vi "Actor Core.vi"(8 "error in":errorcluster, 11 "Machine Interface Actor in":refnum<class "Machine Interface.lvclass">) -> (0 "error out":errorcluster, 3 "Actor out":refnum<class "Actor.lvclass">)   [LabVIEW 2019, in "Machine Interface.lvclass"]
doc: "(<B>Filename</B>: Actor Framework.lvlib:Actor.lvclass:Actor Core.vi)\n\nReceives messages to the actor, reacts to them, and initiates any error handling that may shut the actor down.\n\nDescendant classes may override this VI to append parallel tasks for the actor to complete while it handles messages. Overrides use the Call Parent Method node."
uses:
  Machine Interface.lvclass
  <vilib>/event_ctls.llb/usereventprio.ctl
  <vilib>/ActorFramework/Actor/Actor.lvclass
  <vilib>/ActorFramework/Message Enqueuer/Message Enqueuer.lvclass
  Common/Controls/Acknowledgement.ctl
  Controls/Machine Interface Config File Structure_MI.ctl
  Controls/Local Data_MI.ctl
  Controls/Output Cluster_MI.ctl
  Common/Controls/Diagnostics Result.ctl
  <vilib>/Instr/_visa.llb/VISA Configure Serial Port (Instr).vi
  Controls/Response from Hardware_MI.ctl
  Common/Controls/Pop-up Input.ctl
  C:/Program Files/National Instruments/LabVIEW 2019/vi.lib/ActorFramework/Actor/Actor.lvclass
panel:
  out "LightCamSeqTriggerCount":i32
  in  "MI Offline?":bool
  out "VISA":refnum<visa-resource-name>
  out "VISA resource":refnum<visa-resource-name>
  in  "Message from Arduino":string(combo)
  out "Arduino Read buffer":string
  out "Bytes at Port":u32
  out "Number of Racks":i32
  out "Ping Response, Button Press, Incorrect Opcode":T1
  out "Rack1 Response":T2
  out "Rack2 Response":T2
  in  "OK":bool
  in  "Part Name":string(combo)
  in  "Inspection Status":string(combo)
  out "Label.Text":string
  in  "State Message from Inspection Statemachine":string(combo)
  # "Used for Offline MI Testing"
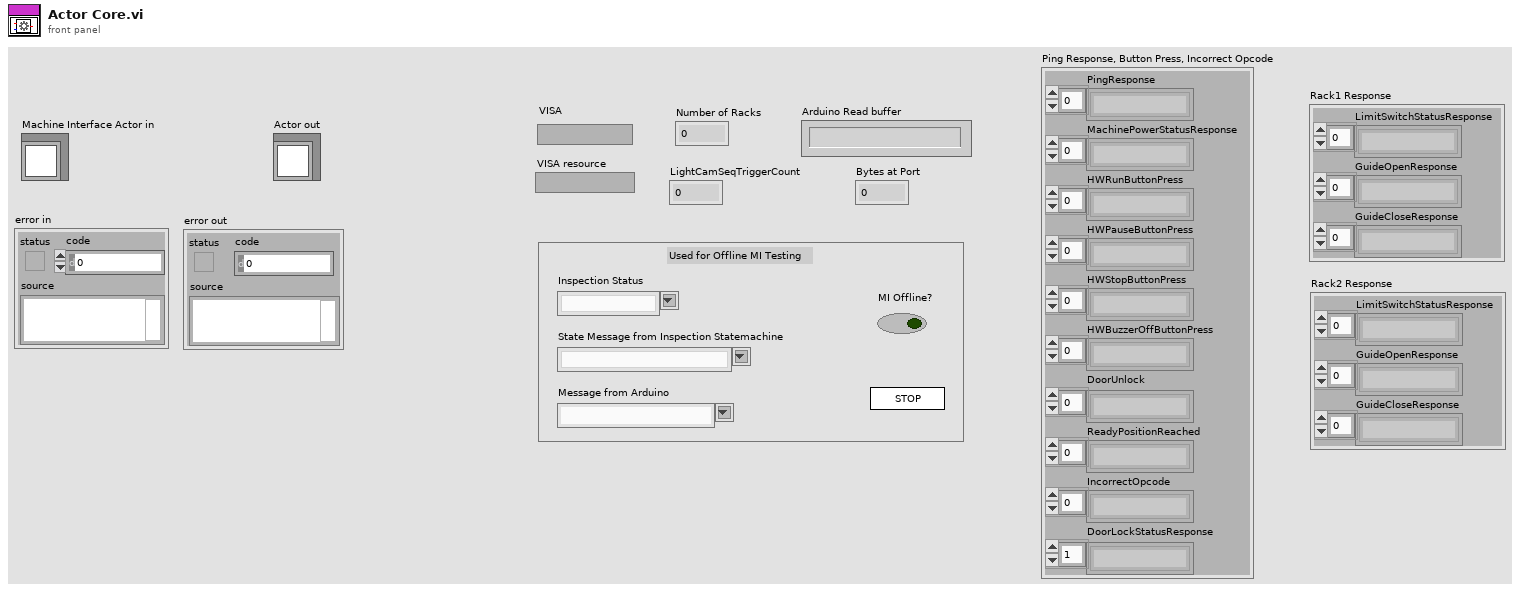
[diagram p1: front panel]
types:
  T1 = typedef "Machine Interface.lvclass/Response from Hardware_MI.ctl" = cluster{"PingResponse":string[], "MachinePowerStatusResponse":string[], "HWRunButtonPress":string[], "HWPauseButtonPress":string[], "HWStopButtonPress":string[], "HWBuzzerOffButtonPress":string[], "DoorUnlock":string[], "ReadyPositionReached":string[], "IncorrectOpcode":string[], "DoorLockStatusResponse":string[]}
  T2 = cluster{"LimitSwitchStatusResponse":string[], "GuideOpenResponse":string[], "GuideCloseResponse":string[]}
  T3 = typedef "Machine Interface.lvclass/Local Data_MI.ctl" = cluster{"Timeout":i32, "Core":cluster{"Current VI Reference":refnum<vi>, "Close Panel on Exit?":bool}, "MIParameters":T4, "Number of Racks":i32, "First Call?":bool, "Message to SM on Timeout":string, "Message from Hardware":string, "Part details":cluster{"Name":string, "RackDependentOpcodes":cluster{"MotorStepsForReadyToInsert":string[], "MotorStepsForReadyToRun":string[], "SetIndex":string[], "EnableSensor":string[], "PowerOnSensor":string[], "DisableSensor":string[], "StartReelerMotor":string[], "StopReelerMotor":string[]}[]}, "State":string, "Ping Response, Button Press, Incorrect Opcode":refnum<vi>[], "Rack1 Response":refnum<vi>[], "Rack2 Response":refnum<vi>[], "LightCamSeqTriggerCount":i32, "Pass after Pause on Fail":bool, "MI Offline?":bool, "Ping Response, Button Press, Incorrect Opcode":T1, "Rack1 Response":cluster{"LimitSwitchStatusResponse":string[], "GuideOpenResponse":string[], "GuideCloseResponse":string[]}, "Rack2 Response":cluster{"LimitSwitchStatusResponse":string[], "GuideOpenResponse":string[], "GuideCloseResponse":string[]}, "Output Cluster_MI":T5, "DisableRun":bool}
  T4 = typedef "Machine Interface.lvclass/Machine Interface Config File Structure_MI.ctl" = cluster{"SpecificationVersion":string, "CompatibleSoftwareVersions":string[], "FrontPanelOpen":bool, "DelayValuesInms":cluster{"TimingUnitSetup":i32, "Strobing":i32, "TowerLampDiagnostics":i32, "Run":i32, "DisableSensors":i32}, "HardwareConfigurationParameters":cluster{"BaudRate":dbl}, "MIRecipeOpcodes":cluster{"DeviceReadiness":cluster{"Ping":string[], "PingResponse":string[]}, "Initialization":cluster{string[]}[], "MachinePowerStatus":cluster{"MachinePowerStatusCheck":string[], "MachinePowerStatusResponse":string[]}, "DoorLockStatus":cluster{"DoorLockStatusCheck":string[], "DoorLockStatusResponse":string[], "Enable":string[], "Disable":string[]}, "OpenLimitSwitchStatus":cluster{"LimitSwitchStatusCheck":string[], "LimitSwitchStatusResponse":string[]}[], "MotorDiagnostics":cluster{"GuideOpen":string[], "GuideOpenResponse":string[], "GuideClose":string[], "GuideCloseResponse":string[], "RotateReelerMotor":string[]}[], "HardwareButtonDiagnostics":cluster{"Run":string[], "Pause":string[], "Stop":string[], "BuzzerOff":string[]}, "TriggerLightCameraSequence":cluster{"Name":string, "On":string[], "Off":string[]}[], "SensorDiagnostics":cluster{"Name":string, "Opcodes":string[]}[], "TowerLampDiagnostics":cluster{"RedLamp":string[], "YellowLamp":string[], "GreenLamp":string[], "Buzzer":string[]}, "Select":cluster{string[]}[], "Run":cluster{"HardwareButtonStatus":string[], "Pass":cluster{"TowerLampStatus":string[]}}, "Pause":cluster{"PauseButtonPress":cluster{string[]}[], "Fail":cluster{string[]}[], "BuzzerOffButtonPress":string[]}, "Exit":cluster{"Shutdown":string[]}, "DHBLS":cluster{string[]}[], "PartsList":cluster{"Name":string, "RackDependentOpcodes":cluster{"MotorStepsForReadyToInsert":string[], "MotorStepsForReadyToRun":string[], "SetIndex":string[], "EnableSensor":string[], "PowerOnSensor":string[], "DisableSensor":string[], "StartReelerMotor":string[], "StopReelerMotor":string[]}[]}[], "HardwareButtonPressed":cluster{"RunButtonPress":string[], "PauseButtonPress":string[], "StopButtonPress":string[], "BuzzerOffButtonPress":string[], "DoorUnlock":string[]}, "ReadyPositionReached":string[], "IncorrectOpcode":string[]}}
  T5 = typedef "Machine Interface.lvclass/Output Cluster_MI.ctl" = cluster{"Acknowledgement":T6, "Diagnostics Result":T7, "Message to SM":string, "Button Press":string, "Error Message":string, "Loading bar cluster":T8}
  T6 = typedef "Acknowledgement.ctl" = cluster{"Enqueuer":refnum<class "Message Enqueuer.lvclass">, "VIReference":refnum<vi>, "VIName":string}
  T7 = typedef "Diagnostics Result.ctl" = cluster{"Result":bool, "StateMessage":string}
  T8 = typedef "Pop-up Input.ctl" = cluster{"Pop-up Type":enum16{"Open Logo Display", "Close Logo Display", "Open Loading Bar", "Close Loading Bar", "Open Alert Display", "Close Alert Display", "One button dialog box", "Two button dialog box", "User Authentication"}, "Title":string, "Message":string, "Button 1 Text":string, "Button 2 Text":string, "Show Close? T/F":bool, "Title Blink? T/F":bool, "Title Blink Colour":u32}
  T9 = enum32{"invalid app kind", "Development System", "Run Time System", "Student Edition", "Embedded LabVIEW", "Evaluation", "Custom"}
  T10 = cluster{"Current VI Reference":refnum<vi>, "Close Panel on Exit?":bool}
  T11 = enum32{"Invalid", "Standard", "Closed", "Hidden", "Minimized", "Maximized"}
  T12 = cluster{"Name":string, "RackDependentOpcodes":cluster{"MotorStepsForReadyToInsert":string[], "MotorStepsForReadyToRun":string[], "SetIndex":string[], "EnableSensor":string[], "PowerOnSensor":string[], "DisableSensor":string[], "StartReelerMotor":string[], "StopReelerMotor":string[]}[]}
  T13 = cluster{"Name":string, "RackDependentOpcodes":cluster{"MotorStepsForReadyToInsert":string[], "MotorStepsForReadyToRun":string[], "SetIndex":string[], "EnableSensor":string[], "PowerOnSensor":string[], "DisableSensor":string[], "StartReelerMotor":string[], "StopReelerMotor":string[]}[]}[]
  T14 = cluster{"MotorStepsForReadyToInsert":string[], "MotorStepsForReadyToRun":string[], "SetIndex":string[], "EnableSensor":string[], "PowerOnSensor":string[], "DisableSensor":string[], "StartReelerMotor":string[], "StopReelerMotor":string[]}[]
  T15 = cluster{"MotorStepsForReadyToInsert":string[], "MotorStepsForReadyToRun":string[], "SetIndex":string[], "EnableSensor":string[], "PowerOnSensor":string[], "DisableSensor":string[], "StartReelerMotor":string[], "StopReelerMotor":string[]}
  T16 = typedef "usereventprio.ctl" = enum32{"high priority", "normal priority"}
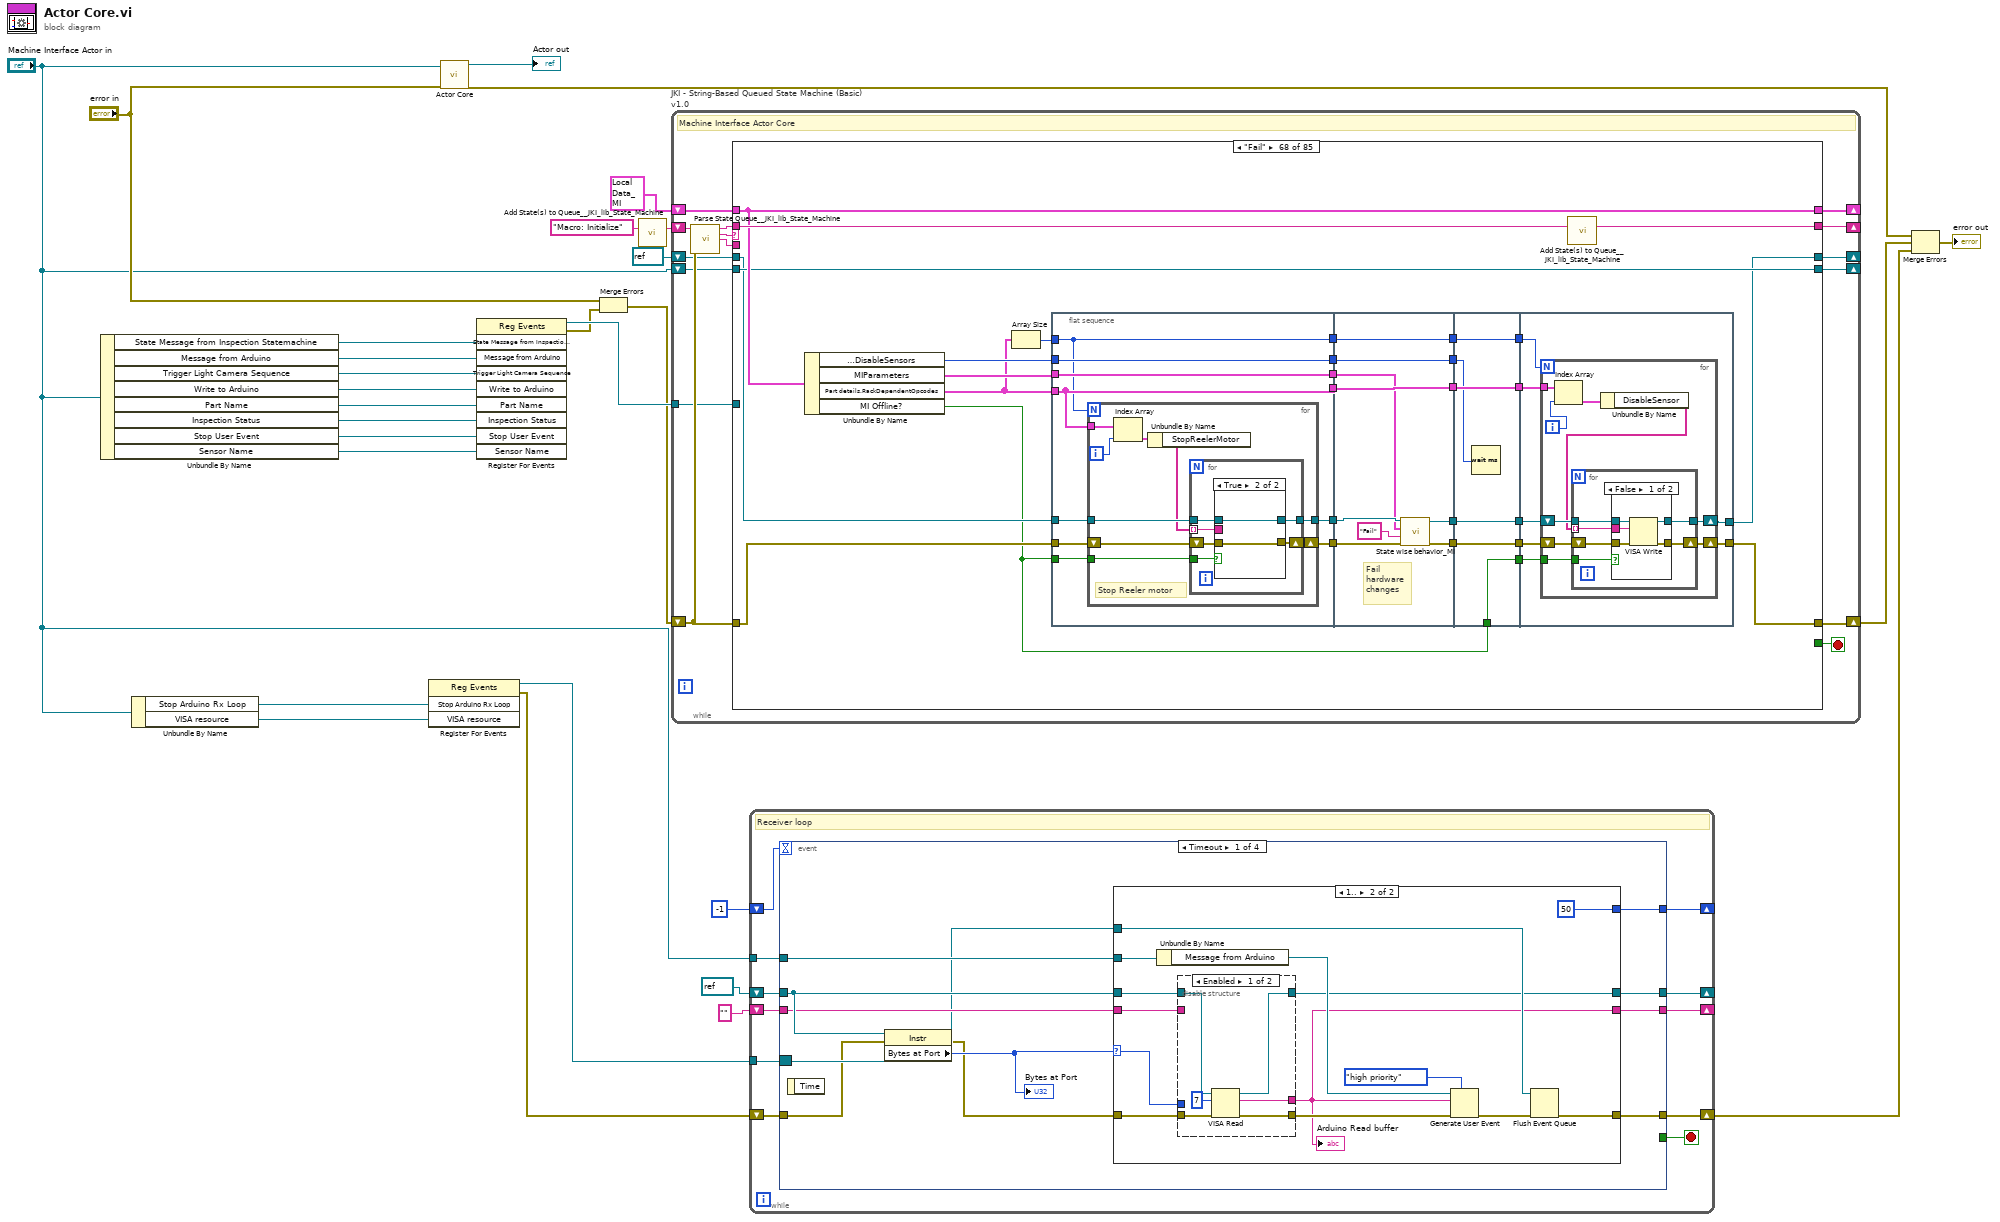
[diagram p0: block diagram]
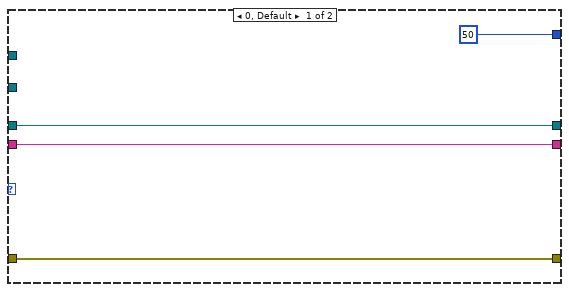
[diagram p2: hidden frame]
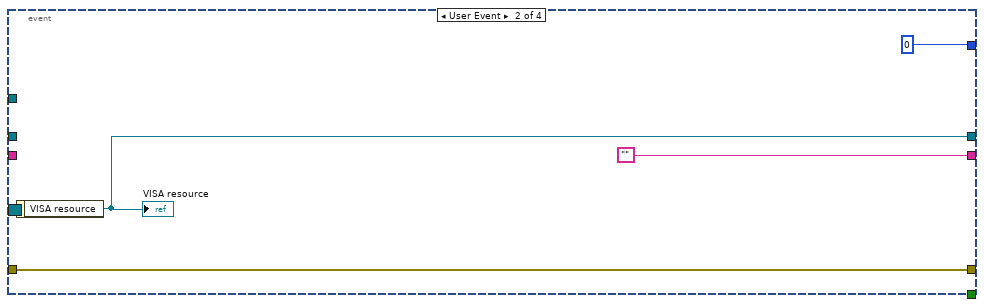
[diagram p4: hidden frame]
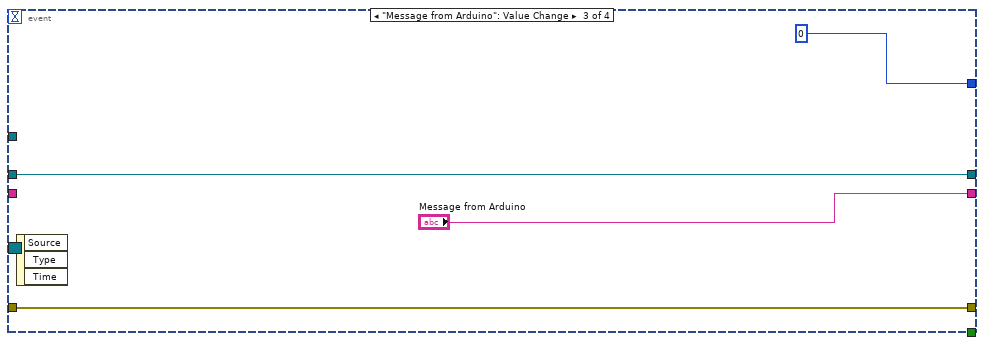
[diagram p5: hidden frame]
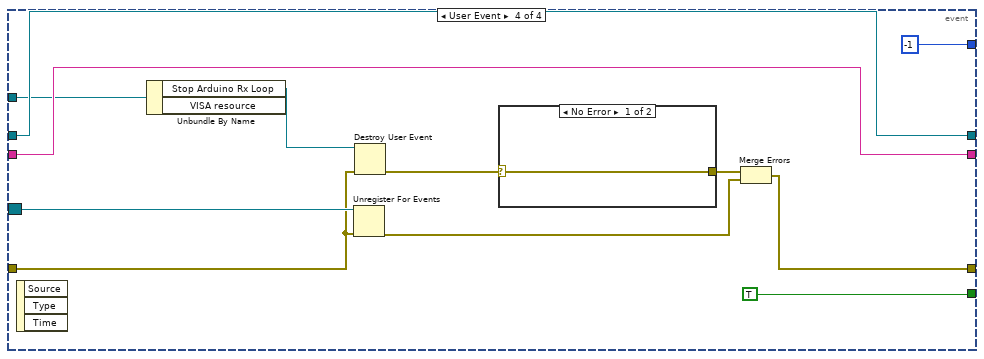
[diagram p6: hidden frame]
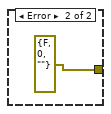
[diagram p7: hidden frame]
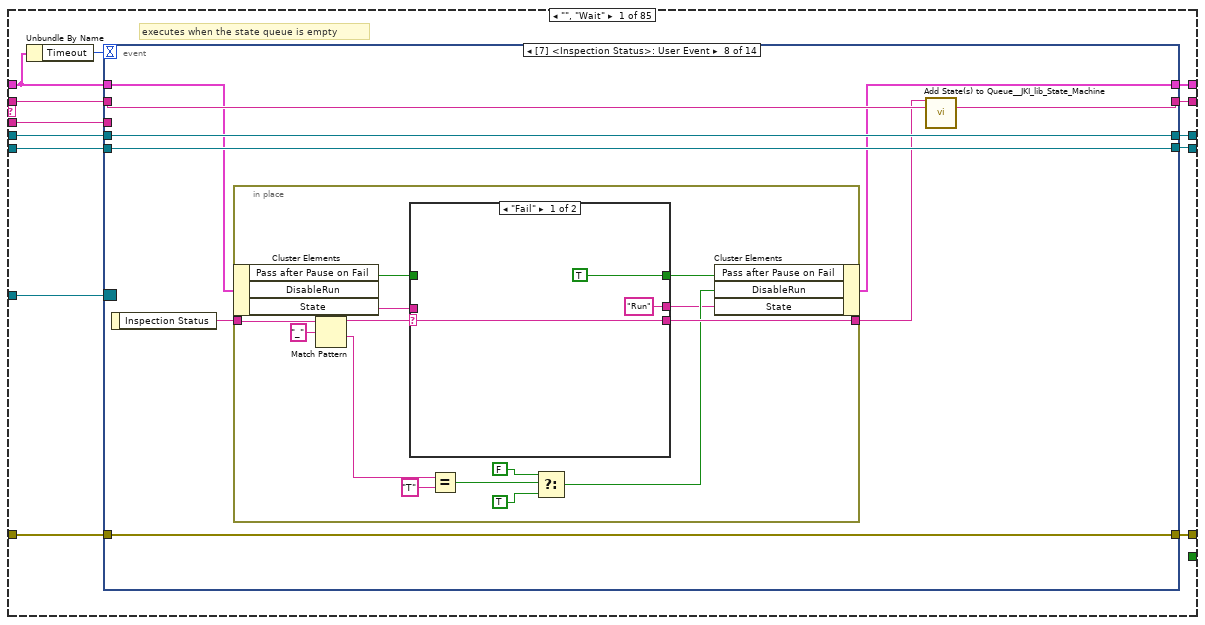
[diagram p8: hidden frame]
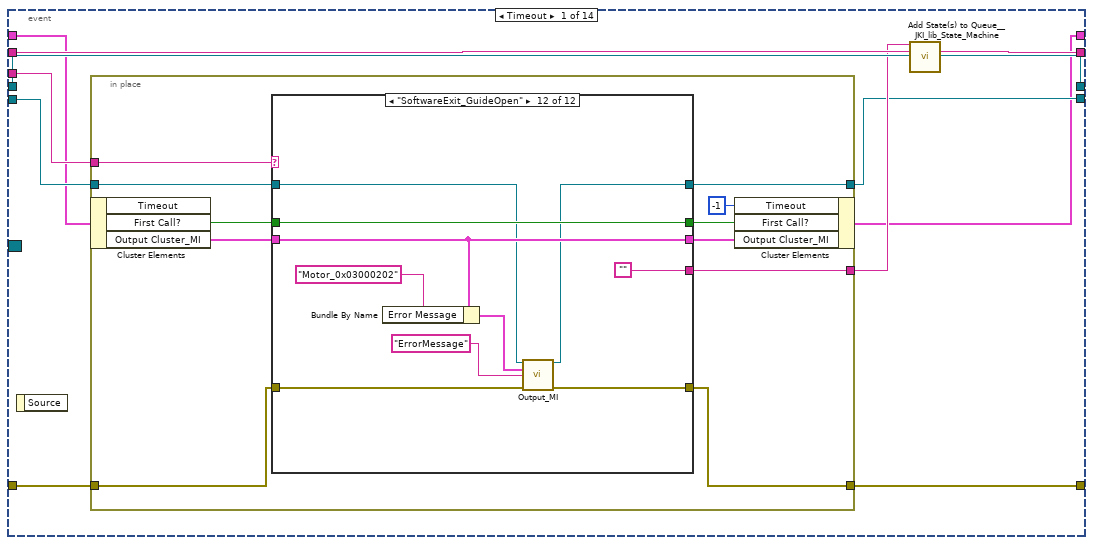
[diagram p9: hidden frame]
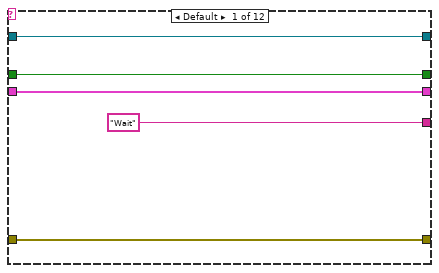
[diagram p10: hidden frame]
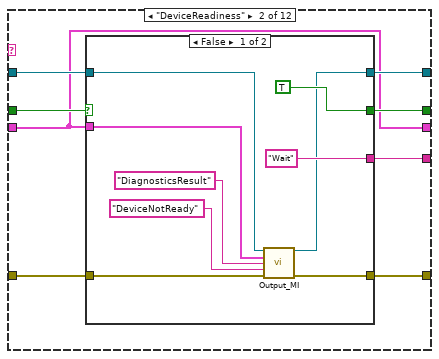
[diagram p11: hidden frame]
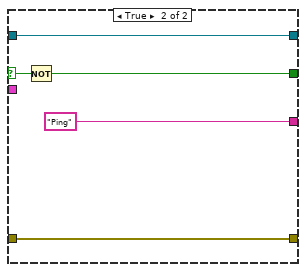
[diagram p12: hidden frame]
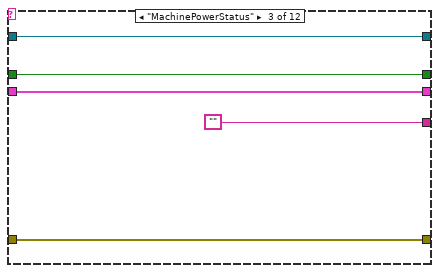
[diagram p13: hidden frame]
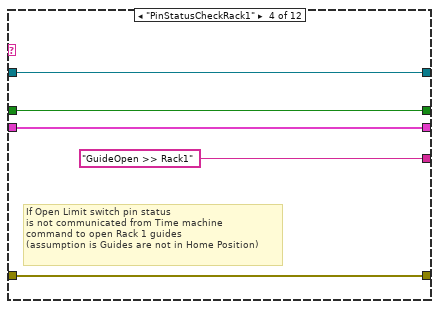
[diagram p14: hidden frame]
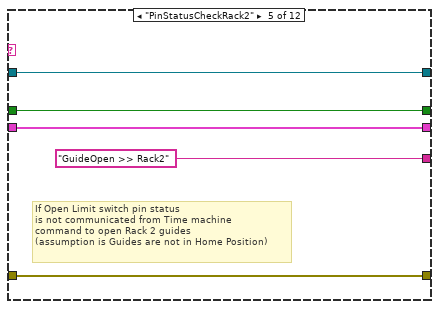
[diagram p15: hidden frame]
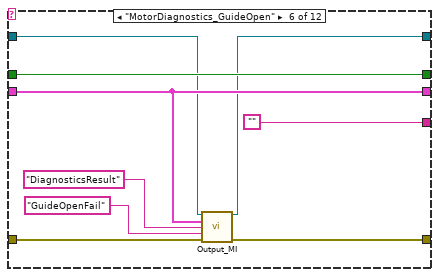
[diagram p16: hidden frame]
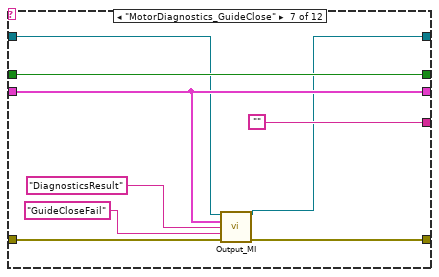
[diagram p17: hidden frame]
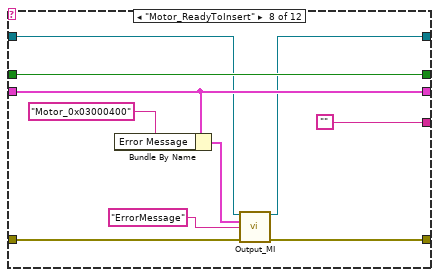
[diagram p18: hidden frame]
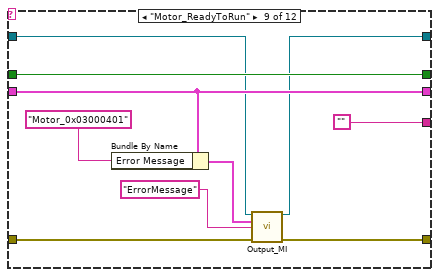
[diagram p19: hidden frame]
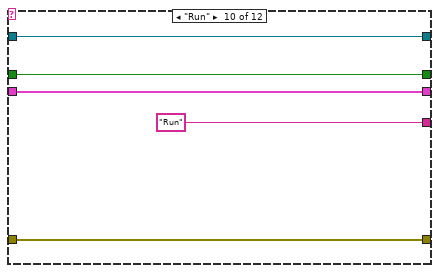
[diagram p20: hidden frame]
diagram:
  n1 = Unbundle By Name("Machine Interface Actor in") -> ("State Message from Inspection Statemachine"=w20:refnum<user-event>, "Message from Arduino"=w19:refnum<user-event>, "Trigger Light Camera Sequence"=w18:refnum<user-event>, "Write to Arduino"=w17:refnum<user-event>, "Part Name"=w16:refnum<user-event>, "Inspection Status"=w15:refnum<user-event>, "Stop User Event"=w12:refnum<user-event>, "Sensor Name"=w8:refnum<user-event>)
  n2 = Unbundle By Name("Machine Interface Actor in") -> ("Stop Arduino Rx Loop"=w6:refnum<user-event>, "VISA resource"=w5:refnum<user-event>)
  n3 = register-events(w6, w5) -> (reference out=w23:refnum<event-registration>, error out=w22:errorcluster)  [unwired: 2 in]
  n4 = call-parent "Actor Core.vi"("error in"="error in", "Actor in"="Machine Interface Actor in") -> ("error out"=w28:errorcluster, "Actor out"=→"Actor out":refnum<class "Actor.lvclass">)  [unwired: 8 in]
  n5 = register-events(w20, w19, w18, w17, w16, w15, w12, w8) -> (reference out=w24:refnum<event-registration>, error out=w14:errorcluster)  [unwired: 2 in]
  n6 = Merge Errors("error in", w14) -> (w13:errorcluster)
  n7 = call <vilib>:"Add State(s) to Queue__JKI_lib_State_Machine.vi"("State(s) in (\"\")"="Macro: Initialize") -> ("States Out"=w26:string)  [unwired: 14 in]
  n8 = while "JKI - String-Based Queued State Machine (Basic) v1.0" {
    shift-right: [w37] -> _
    shift-left: T3 {"Timeout"=0, "Core"={"Current VI Reference"=refnum, "Close Panel on Exit?"=FALSE}, "MIParameters"={"SpecificationVersion"="", "CompatibleSoftwareVersions"=[], "FrontPanelOpen"=FALSE, "DelayValuesInms"={"TimingUnitSetup"=0, "Strobing"=0, "TowerLampDiagnostics"=0, "Run"=0, "DisableSensors"=0}, "HardwareConfigurationParameters"={"BaudRate"=0.0}, "MIRecipeOpcodes"={"DeviceReadiness"={"Ping"=[], "PingResponse"=[]}, "Initialization"=[], "MachinePowerStatus"={"MachinePowerStatusCheck"=[], "MachinePowerStatusResponse"=[]}, "DoorLockStatus"={"DoorLockStatusCheck"=[], "DoorLockStatusResponse"=[], "Enable"=[], "Disable"=[]}, "OpenLimitSwitchStatus"=[], "MotorDiagnostics"=[], "HardwareButtonDiagnostics"={"Run"=[], "Pause"=[], "Stop"=[], "BuzzerOff"=[]}, "TriggerLightCameraSequence"=[], "SensorDiagnostics"=[], "TowerLampDiagnostics"={"RedLamp"=[], "YellowLamp"=[], "GreenLamp"=[], "Buzzer"=[]}, "Select"=[], "Run"={"HardwareButtonStatus"=[], "Pass"={"TowerLampStatus"=[]}}, "Pause"={"PauseButtonPress"=[], "Fail"=[], "BuzzerOffButtonPress"=[]}, "Exit"={"Shutdown"=[]}, "DHBLS"=[], "PartsList"=[], "HardwareButtonPressed"={"RunButtonPress"=[], "PauseButtonPress"=[], "StopButtonPress"=[], "BuzzerOffButtonPress"=[], "DoorUnlock"=[]}, "ReadyPositionReached"=[], "IncorrectOpcode"=[]}}, "Number of Racks"=0, "First Call?"=FALSE, "Message to SM on Timeout"="", "Message from Hardware"="", "Part details"={"Name"="", "RackDependentOpcodes"=[]}, "State"="", "Ping Response, Button Press, Incorrect Opcode"=[], "Rack1 Response"=[], "Rack2 Response"=[], "LightCamSeqTriggerCount"=0, "Pass after Pause on Fail"=FALSE, "MI Offline?"=FALSE, "Ping Response, Button Press, Incorrect Opcode"={"PingResponse"=[], "MachinePowerStatusResponse"=[], "HWRunButtonPress"=[], "HWPauseButtonPress"=[], "HWStopButtonPress"=[], "HWBuzzerOffButtonPress"=[], "DoorUnlock"=[], "ReadyPositionReached"=[], "IncorrectOpcode"=[], "DoorLockStatusResponse"=[]}, "Rack1 Response"={"LimitSwitchStatusResponse"=[], "GuideOpenResponse"=[], "GuideCloseResponse"=[]}, "Rack2 Response"={"LimitSwitchStatusResponse"=[], "GuideOpenResponse"=[], "GuideCloseResponse"=[]}, "Output Cluster_MI"={"Acknowledgement"={"Enqueuer"=refnum, "VIReference"=refnum, "VIName"=""}, "Diagnostics Result"={"Result"=FALSE, "StateMessage"=""}, "Message to SM"="", "Button Press"="", "Error Message"="", "Loading bar cluster"={"Pop-up Type"=enum."Open Logo Display", "Title"="", "Message"="", "Button 1 Text"="", "Button 2 Text"="", "Show Close? T/F"=FALSE, "Title Blink? T/F"=FALSE, "Title Blink Colour"=0}}, "DisableRun"=FALSE} ("Local Data_MI") -> [w36]
    shift-right: [w40] -> w10
    shift-left: w13 -> [w35]
    shift-right: [w39] -> _
    shift-left: w26 -> [w41]
    shift-right: [w34] -> _
    shift-left: refnum<visa-resource-name> refnum ("VISA resource name out") -> [w33]
    tunnel: w24 -> [w32]
    shift-right: [w30] -> _
    shift-left: "Machine Interface Actor in" -> [w31]
    stop <- w38 stop-if-true
    # "Machine Interface Actor Core"
    n9 = call <vilib>:"Parse State Queue__JKI_lib_State_Machine.vi"("State Queue"=w41, "Error In (no error)"=w35) -> ("Remaining States"=w43:string, "Current State"=w44:string, "Arguments"=w42:string)  [unwired: 11 in]
    n10 = case shown="\"Fail\"" w44 {
      selector: w44 -> [_ _ w475 _ _ _ _ _ _ _ _ _ _ _ _ _ _ _ _ _ _ _ _ _ _ _ _ _ _ _ _ _ _ _ _ _ _ _ _ _ _ _ _ _ _ _ _ _ _ _ _ _ _ _ _ _ _ _ _ _ _ _ _ _ _ _ _ _ _ _ _ _ _ _ _ _ _ _ _ _ _ _ _ _ _]
      tunnel: w43 -> [w57 w472 w479 w499 w509 w579 w585 w617 w650 w660 w666 w675 w703 w717 w729 w735 w751 w790 w804 w818 w824 w838 w844 w857 w873 w893 w903 w916 w936 w952 w960 w982 w998 w1052 w1100 w1344 w1372 w1427 w1434 w1449 w1455 w1468 w1474 w1485 w1491 w1501 w1513 w1522 w1537 w1593 w1605 w1658 w1670 w1676 w1685 w1700 w1715 w1749 w1804 w1818 w1870 w1922 w1977 w1987 w1993 w2008 w2058 w2162 w2253 w2285 w2300 w2331 w2341 w2351 w2361 w2368 w2374 w2387 w2402 w2409 w2415 w2428 w2437 w2455 w2470]
      tunnel: w42 -> [w49 _ _ _ _ _ _ _ _ _ _ w669 _ _ _ _ _ _ _ _ _ _ _ _ _ _ _ _ _ w944 w955 _ w988 w1046 w1093 w1338 w1369 w1420 _ _ _ _ _ _ _ _ w1505 _ w1535 _ w1603 _ _ _ _ _ _ w1747 _ w1816 w1868 w1920 _ _ _ _ _ _ _ _ _ _ _ _ _ _ _ _ _ _ _ _ _ _ _]
      tunnel: w36 -> [w45 w469 w477 w490 w503 w577 w582 _ w646 w657 w664 w671 w700 w709 w721 w732 w742 w787 w798 w811 w821 w833 w841 w848 w861 w890 w896 w910 w933 w940 w953 w979 w993 w1041 w1088 w1331 w1365 w1425 w1431 w1444 w1452 w1465 w1471 w1479 w1488 w1499 w1503 w1519 w1526 w1585 w1596 w1656 w1668 w1673 w1678 w1695 w1710 w1738 w1801 w1807 w1861 w1913 w1963 w1985 w1990 w2003 w2052 w2157 w2251 w2282 w2295 w2329 w2332 w2342 w2352 w2362 w2371 w2379 w2400 w2404 w2410 w2420 w2430 w2450 w2465]
      tunnel: [w55 w470 w481 w496 errorcluster {"status"=FALSE, "code"=0, "source"=""} ("error out") w576 w583 w592 w647 w658 w663 w672 w701 w712 w720 w733 w744 w788 w796 w810 w822 w832 w842 w852 w866 w891 w897 w906 w934 w946 w958 w980 w991 w1051 w1091 w1342 w1366 w1416 w1432 w1438 w1453 w1464 w1472 w1480 w1489 w1495 w1506 w1515 w1533 w1587 w1600 w1653 w1661 w1674 w1683 w1698 w1711 w1745 w1799 w1813 w1865 w1917 w1975 w1980 w1991 w2004 w2055 w2159 w2246 w2283 w2296 w2322 w2335 w2345 w2355 w2364 w2372 w2377 w2397 w2407 w2413 w2421 w2433 w2451 w2461] -> w40
      tunnel: w35 -> [w54 w470 w480 w496 w504 w576 w583 w602 w623 w658 w663 w673 w701 w713 w720 w733 w745 w788 w797 w812 w822 w829 w842 w853 w867 w891 w898 w907 w934 w947 w958 w980 w992 w1044 w1092 w1335 w1367 w1422 w1432 w1442 w1453 w1463 w1472 w1481 w1489 w1496 w1507 w1515 w1534 w1586 w1601 w1648 w1664 w1674 w1683 w1698 w1712 w1746 w1800 w1814 w1866 w1918 w1970 w1981 w1991 w2005 w2056 w2160 w2247 w2283 w2297 w2323 w2336 w2346 w2356 w2364 w2372 w2378 w2393 w2407 w2413 w2422 w2434 w2451 w2462]
      tunnel: [w56 w471 w478 w498 w508 w578 w584 w616 w649 w659 w665 w674 w702 w716 w728 w734 w750 w789 w803 w817 w823 w837 w843 w856 w872 w892 w902 w915 w935 w951 w959 w981 w997 w1053 w1099 w1343 w1371 w1428 w1433 w1448 w1454 w1467 w1473 w1484 w1490 w1500 w1512 w1521 w1536 w1592 w1604 w1657 w1669 w1675 w1684 w1699 w1714 w1748 w1803 w1817 w1869 w1921 w1976 w1986 w1992 w2007 w2057 w2161 w2252 w2284 w2299 w2330 w2340 w2350 w2360 w2367 w2373 w2386 w2401 w2408 w2414 w2427 w2436 w2454 w2469] -> w39
      tunnel: [_ _ _ _ _ TRUE _ _ _ _ _ _ _ _ _ _ _ _ _ _ _ _ _ _ _ _ _ _ _ _ _ _ _ _ _ _ _ _ _ _ _ _ _ _ _ _ _ _ _ _ _ _ _ _ _ _ _ _ _ _ _ _ _ _ _ _ _ _ _ _ _ _ _ _ _ _ _ _ _ _ _ _ _ _ _] -> w38
      tunnel: [w53 w469 w477 w497 w503 w577 w582 w615 w646 w657 w664 w671 w700 w709 w721 w732 w742 w787 w800 w814 w821 w833 w841 w847 w869 w890 w896 w910 w933 w939 w953 w979 w995 w1040 w1095 w1330 w1365 w1424 w1431 w1446 w1452 w1465 w1471 w1479 w1488 w1499 w1510 w1518 w1525 w1590 w1596 w1655 w1667 w1673 w1677 w1694 w1710 w1737 w1801 w1806 w1861 w1913 w1963 w1985 w1990 w2003 w2051 w2157 w2251 w2282 w2295 w2328 w2332 w2342 w2352 w2362 w2371 w2384 w2400 w2404 w2410 w2420 w2430 w2449 w2465] -> w37
      tunnel: w33 -> [w52 w468 w474 w488 w505 w575 w581 w603 w624 w656 w662 w668 w699 w714 w719 w731 _ w786 w792 w816 w820 w826 w840 w846 w871 w889 w895 w914 w932 w938 w957 w978 w989 w1038 w1098 w1329 w1370 w1413 w1430 w1436 w1451 w1458 w1470 w1476 w1487 w1493 w1511 w1520 w1532 w1588 w1599 w1649 w1660 w1672 w1682 w1697 w1705 w1744 w1802 w1812 w1864 w1916 w1967 w1979 w1989 w1998 w2049 w2155 w2249 w2281 w2290 w2321 w2334 w2344 w2354 w2366 w2370 w2376 w2391 w2406 w2412 w2426 w2435 w2453 w2468]
      tunnel: [w51 w468 w474 w488 w505 w575 w581 w603 w624 w656 w662 w668 w699 w714 w719 w731 w743 w786 w791 w816 w820 w825 w840 w845 w871 w889 w894 w914 w932 w937 w957 w978 w990 w1037 w1098 w1328 w1370 w1414 w1430 w1435 w1451 w1457 w1470 w1475 w1487 w1492 w1511 w1520 w1531 w1588 w1598 w1649 w1659 w1672 w1682 w1697 w1704 w1743 w1802 w1811 w1863 w1915 w1966 w1978 w1989 w1997 w2048 w2154 w2248 w2281 w2289 w2320 w2333 w2343 w2353 w2366 w2370 w2375 w2390 w2406 w2412 w2426 w2435 w2453 w2468] -> w34
      tunnel: w32 -> [w50 _ _ _ _ _ _ _ w622 _ _ _ _ _ _ _ _ _ _ _ _ _ _ _ _ _ _ _ _ _ _ _ _ _ _ _ _ _ _ _ _ _ _ _ _ _ _ _ _ _ _ _ _ _ _ _ _ _ _ _ _ _ _ _ _ _ _ _ _ _ _ _ _ _ _ _ _ _ _ _ _ _ _ _ _]
      tunnel: w31 -> [w48 w467 w473 w486 w501 w573 w580 w605 w621 w655 w661 w667 w698 w705 w718 w730 w737 w785 w799 w806 w819 w835 w839 w854 w859 w888 w901 w905 w931 w948 w954 w977 w984 w1036 w1085 w1327 w1359 w1426 w1429 w1445 w1450 w1466 w1469 w1482 w1486 w1498 w1509 w1517 w1528 w1581 w1595 w1647 w1665 w1671 w1679 w1696 w1702 w1740 w1795 w1809 w1860 w1912 w1965 w1984 w1988 w1995 w2050 w2156 w2240 w2280 w2287 w2326 w2339 w2349 w2359 w2363 w2369 w2382 w2389 w2403 w2411 w2417 w2432 w2452 w2457]
      tunnel: [w47 w467 w473 w486 w500 w573 w580 w605 w621 w655 w661 w667 w698 w704 w718 w730 w736 w785 w799 w805 w819 w835 w839 w854 w858 w888 w901 w904 w931 w948 w954 w977 w983 w1035 w1084 w1326 w1358 w1426 w1429 w1445 w1450 w1466 w1469 w1482 w1486 w1498 w1509 w1517 w1528 w1580 w1595 w1646 w1665 w1671 w1679 w1696 w1701 w1740 w1794 w1809 w1860 w1912 w1964 w1984 w1988 w1994 w2050 w2156 w2239 w2280 w2286 w2326 w2339 w2349 w2359 w2363 w2369 w2382 w2388 w2403 w2411 w2416 w2431 w2452 w2456] -> w30
      frame "", "Wait" {
        # "executes when the state queue is empty"
        # "executes when the state queue is empty"
        n11 = Unbundle By Name(w45) -> ("Timeout"=w46:i32)
        n12 = event shown="[7] <Inspection Status>: User Event" {
          selector: w50 -> [_ _ _ w269 _ _ _ _ _ _ _ _ _ _]
          dyn-events: _ -> [_ _ _ _ _ _ _ _ _ _ _ _ _ _]
          timeout: w46 -> [_ _ _ _ _ _ _ _ _ _ _ _ _ _]
          tunnel: w57 -> [w66 w196 w225 w278 w325 w354 w374 w383 w421 w432 w439 w442 w455 w464]
          tunnel: [w68 w195 w226 w277 w326 w353 w375 w384 w423 w431 w438 w441 w456 w465] -> w56
          tunnel: w45 -> [w59 w186 w212 w263 w315 w346 w376 w378 w424 w429 w434 w444 w457 w466]
          tunnel: [w61 w193 w217 w275 w320 w347 w372 w382 w419 w430 w437 w445 w451 w462] -> w55
          tunnel: w54 -> [w62 w193 w215 w276 w323 w352 w372 w382 w419 w430 w437 w446 w452 w463]
          tunnel: [w58 w188 w211 w266 w313 w346 w376 w377 w424 w429 w434 w444 w457 w466] -> w53
          tunnel: w52 -> [w67 w194 w221 w268 w324 w340 w373 w385 w422 w426 w435 w443 w450 w459]
          tunnel: [w67 w194 w221 w267 w322 w349 w373 w385 w422 w426 w435 w443 w450 w459] -> w51
          tunnel: w49 -> [w64 _ _ _ w312 _ _ _ _ _ _ _ _ _]
          tunnel: w48 -> [w63 w192 w208 w264 w316 w348 w368 w381 w418 w425 w433 w440 w449 w458]
          tunnel: [w60 w192 w208 w264 w316 w348 w368 w381 w418 w425 w433 w440 w449 w458] -> w47
          event Timeout {
            n13 = event-data() -> ()  [unwired: 1 in, 1 out]
            n14 = in-place {
              in-place-border: [w79] -> w65
              in-place-border: w64 -> [w78]
              in-place-border: w63 -> [w77]
              in-place-border: w62 -> [w76]
              in-place-border: [w75] -> w61
              in-place-border: [w74] -> w60
              n15 = in-place-cluster #1(w59) -> ("First Call?"=w73:bool, "Output Cluster_MI"=w72:T5)  [unwired: 1 out]
              n16 = case shown="\"SoftwareExit_GuideOpen\"" w78 {
                tunnel: ["Wait" w92 "" "GuideOpen >> Rack1" "GuideOpen >> Rack2" "" "" "" "" "Run" "" ""] -> w79
                tunnel: w73 -> [w83 w91 w111 w116 w121 w129 w138 w148 w159 w163 w173 w183]
                tunnel: [w83 w90 w111 w116 w121 w129 w138 w148 w159 w163 w173 w183] -> w71
                tunnel: w77 -> [w81 w89 w108 w113 w118 w123 w132 w141 w151 w162 w166 w176]
                tunnel: w76 -> [w82 w88 w109 w114 w119 w128 w136 w147 w154 w164 w168 w179]
                tunnel: [w82 w87 w109 w114 w119 w127 w137 w146 w153 w164 w167 w178] -> w75
                tunnel: [w81 w86 w108 w113 w118 w122 w131 w140 w150 w162 w165 w175] -> w74
                tunnel: w72 -> [w80 w85 w107 w112 w117 w124 w135 w144 w155 w160 w169 w177]
                tunnel: [w80 w85 w107 w112 w117 w124 w135 w144 w155 w160 w169 w177] -> w69
                frame Default {
                }
                frame "DeviceReadiness" {
                  n17 = case shown="False" w91 {
                    selector: w91 -> [_ w105]
                    tunnel: ["Wait" "Ping"] -> w92
                    tunnel: [TRUE w104] -> w90
                    tunnel: w89 -> [w94 w102]
                    tunnel: w88 -> [w99 w103]
                    tunnel: [w98 w103] -> w87
                    tunnel: [w93 w102] -> w86
                    tunnel: w85 -> [w97 _]
                    frame False {
                      n18 = call "Output_MI.vi"("Machine Interface Actor in"=w94, "Output Cluster_MI"=w97, "State"="DiagnosticsResult", "Sub State"="DeviceNotReady", "error in (no error)"=w99) -> ("Machine Interface Actor out"=w93:refnum<class "Machine Interface.lvclass">, "error out"=w98:errorcluster)  [unwired: 9 in]
                    }
                    frame True {
                      n19 = Not(x=w105) -> (.not. x?=w104:bool)
                    }
                  }
                }
                frame "MachinePowerStatus" {
                }
                frame "PinStatusCheckRack1" {
                  # "If Open Limit switch pin status\nis not communicated from Time machine\ncommand to open Rack 1 guides \n(assumption is Guides are not in Home Position)"
                }
                frame "PinStatusCheckRack2" {
                  # "If Open Limit switch pin status\nis not communicated from Time machine\ncommand to open Rack 2 guides \n(assumption is Guides are not in Home Position)"
                }
                frame "MotorDiagnostics_GuideOpen" {
                  n20 = call "Output_MI.vi"("Machine Interface Actor in"=w123, "Output Cluster_MI"=w124, "State"="DiagnosticsResult", "Sub State"="GuideOpenFail", "error in (no error)"=w128) -> ("Machine Interface Actor out"=w122:refnum<class "Machine Interface.lvclass">, "error out"=w127:errorcluster)  [unwired: 9 in]
                }
                frame "MotorDiagnostics_GuideClose" {
                  n21 = call "Output_MI.vi"("Machine Interface Actor in"=w132, "Output Cluster_MI"=w135, "State"="DiagnosticsResult", "Sub State"="GuideCloseFail", "error in (no error)"=w136) -> ("Machine Interface Actor out"=w131:refnum<class "Machine Interface.lvclass">, "error out"=w137:errorcluster)  [unwired: 9 in]
                }
                frame "Motor_ReadyToInsert" {
                  n22 = Bundle By Name(cluster=w144, "Error Message"="Motor_0x03000400") -> (w143:T5)
                  n23 = call "Output_MI.vi"("Machine Interface Actor in"=w141, "Output Cluster_MI"=w143, "State"="ErrorMessage", "error in (no error)"=w147) -> ("Machine Interface Actor out"=w140:refnum<class "Machine Interface.lvclass">, "error out"=w146:errorcluster)  [unwired: 10 in]
                }
                frame "Motor_ReadyToRun" {
                  n24 = Bundle By Name(cluster=w155, "Error Message"="Motor_0x03000401") -> (w158:T5)
                  n25 = call "Output_MI.vi"("Machine Interface Actor in"=w151, "Output Cluster_MI"=w158, "State"="ErrorMessage", "error in (no error)"=w154) -> ("Machine Interface Actor out"=w150:refnum<class "Machine Interface.lvclass">, "error out"=w153:errorcluster)  [unwired: 10 in]
                }
                frame "Run" {
                }
                frame "Stop_GuideOpen" {
                  n26 = Bundle By Name(cluster=w169, "Error Message"="Motor_0x03000201") -> (w172:T5)
                  n27 = call "Output_MI.vi"("Machine Interface Actor in"=w166, "Output Cluster_MI"=w172, "State"="ErrorMessage", "error in (no error)"=w168) -> ("Machine Interface Actor out"=w165:refnum<class "Machine Interface.lvclass">, "error out"=w167:errorcluster)  [unwired: 10 in]
                }
                frame "SoftwareExit_GuideOpen" {
                  n28 = Bundle By Name(cluster=w177, "Error Message"="Motor_0x03000202") -> (w182:T5)
                  n29 = call "Output_MI.vi"("Machine Interface Actor in"=w176, "Output Cluster_MI"=w182, "State"="ErrorMessage", "error in (no error)"=w179) -> ("Machine Interface Actor out"=w175:refnum<class "Machine Interface.lvclass">, "error out"=w178:errorcluster)  [unwired: 10 in]
                }
              }
              n30 = in-place-cluster #1("Timeout"=-1, "First Call?"=w71, "Output Cluster_MI"=w69) -> (w58:T3)
            }
            n31 = call <vilib>:"Add State(s) to Queue__JKI_lib_State_Machine.vi"("State(s) in Front (\"\")"=w65, "State(s) in (\"\")"=w66) -> ("States Out"=w68:string)  [unwired: 13 in]
          }
          event User Event {
            n32 = event-data() -> ("State Message from Inspection Statemachine"=w191:string)  [unwired: 1 in]
            n33 = Unbundle By Name(w186) -> ("MIParameters.DelayValuesInms.Run"=w189:i32)
            n34 = case shown="Default" w191 {
              selector: w191 -> [w198 _ w203]
              tunnel: [-1 w201 -1 ("Run")] -> w187
              tunnel: [w198 "Wait >> Run" ""] -> w190
              tunnel: w189 -> [_ w201 _]
              tunnel: w186 -> [w197 w200 w205]
              tunnel: [w197 w200 w204] -> w185
              frame Default {
              }
              frame "Run" {
                # "Run command will be executed after\ndelay of 50 ms. This is done to process\nqueued results (if any) before executing \nRun"
              }
              frame "MasterSample" {
                n35 = Bundle By Name(cluster=w205, "State"=w203) -> (w204:T3)
              }
            }
            n36 = Bundle By Name(cluster=w185, "Timeout"=w187) -> (w188:T3)
            n37 = call <vilib>:"Add State(s) to Queue__JKI_lib_State_Machine.vi"("State(s) in Front (\"\")"=w190, "State(s) in (\"\")"=w196) -> ("States Out"=w195:string)  [unwired: 13 in]
          }
          event User Event {
            # "Checks if message from Time Machine\nis Ping Response or Button press\nor incorrect opcode"
            n38 = event-data() -> ("Message from Arduino"=w210:string)  [unwired: 1 in]
            n39 = Unbundle By Name(w212) -> ("Ping Response, Button Press, Incorrect Opcode"=w209:refnum<vi>[], "Rack1 Response"=w214:refnum<vi>[], "Rack2 Response"=w213:refnum<vi>[])
            n40 = call "Response from Arduino_MI.vi"("error in (no error)"=w215, "Message from Arduino"=w210, "Controls[]"=w209) -> ("error out"=w222:errorcluster, "Opcode Present"=w223:bool, "Index"=w224:i32)  [unwired: 6 in]
            n41 = case shown="True" w223 {
              tunnel: w224 -> [_ w257]
              tunnel: [w250 w254] -> w216
              tunnel: w209 -> [_ w255]
              tunnel: w222 -> [w244 w253]
              tunnel: w210 -> [w249 _]
              tunnel: [w248 w253] -> w218
              tunnel: [w246 TRUE ("Opcode Present")] -> w219
              tunnel: w214 -> [w245 _]
              frame False {
                # "Rack 1 Response"
                n42 = call "Response from Arduino_MI.vi"("error in (no error)"=w244, "Message from Arduino"=w249, "Controls[]"=w245) -> ("error out"=w248:errorcluster, "Opcode Present"=w246:bool, "Index"=w247:i32)  [unwired: 6 in]
                n43 = Index Array(array=w245, index=w247) -> (element=w251:refnum<vi>)
                n44 = property class="Ctl"(reference=w251) -> ("Label.Text"=w243:string)  [unwired: 1 in, 2 out]
                n45 = Concatenate Strings(w243, " >> Rack1" ("string")) -> (w250:string)
              }
              frame True {
                n46 = Index Array(array=w255, index=w257) -> (element=w256:refnum<vi>)
                n47 = property class="Ctl"(reference=w256) -> ("Label.Text"=w254:string)  [unwired: 1 in, 2 out]
              }
            }
            n48 = case shown="False" w219 {
              tunnel: [w229 w240] -> w220
              tunnel: w218 -> [w232 w241]
              tunnel: w210 -> [w236 _]
              tunnel: [w235 w241] -> w217
              tunnel: w213 -> [w233 _]
              tunnel: w216 -> [_ w240]
              frame False {
                # "Rack 2 Response"
                n49 = call "Response from Arduino_MI.vi"("error in (no error)"=w232, "Message from Arduino"=w236, "Controls[]"=w233) -> ("error out"=w235:errorcluster, "Opcode Present"=w231:bool, "Index"=w234:i32)  [unwired: 6 in]
                n50 = Index Array(array=w233, index=w234) -> (element=w237:refnum<vi>)
                n51 = property class="Ctl"(reference=w237) -> ("Label.Text"=w228:string)  [unwired: 1 in, 2 out]
                n52 = Concatenate Strings(w228, " >> Rack2" ("string")) -> (w230:string)
                n53 = case shown="False" w231 {
                  tunnel: w230 -> [_ w239]
                  tunnel: ["Unknown Response" w239] -> w229
                  frame False {
                  }
                  frame True {
                  }
                }
              }
              frame True {
              }
            }
            "Label.Text" <- w220
            n54 = Bundle By Name(cluster=w212, "Message from Hardware"=w210) -> (w211:T3)
            n55 = call <vilib>:"Add State(s) to Queue__JKI_lib_State_Machine.vi"("State(s) in Front (\"\")"=w220, "State(s) in (\"\")"=w225) -> ("States Out"=w226:string)  [unwired: 13 in]
          }
          event User Event {
            n56 = event-data() -> ("Mode"=w260:string, "Light Sequence Trigger"=w274:string, "Status"=w273:string)  [unwired: 1 in]
            n57 = in-place {
              in-place-border: [w279] -> w262
              n58 = in-place-cluster #2(w263) -> ("LightCamSeqTriggerCount"=w281:i32, "MIParameters"=w279:T4)
              n59 = Increment(x=w281) -> (x+1=w280:i32)
              n60 = in-place-cluster #2("LightCamSeqTriggerCount"=w280, "MIParameters"=w279) -> (w261:T3)
            }
            n61 = call "Read Trigger Light Camera Sequence Opcode_MI.vi"("error in (no error)"=w276, "Status"=w273, "Light Sequence Trigger"=w274, "MachineInterfaceRecipeOpcodes"=w262) -> ("error out"=w272:errorcluster, "Trigger Light Camera Sequence Opcode"=w271:string[])  [unwired: 6 in]
            n62 = Unbundle By Name(w262) -> ("DelayValuesInms.Strobing"=w265:i32)
            n63 = Unbundle By Name(w264) -> ("Write to Arduino"=w270:refnum<user-event>)
            n64 = case shown="\"On\"" w273 {
              tunnel: w272 -> [w287 w303]
              tunnel: [w289 w302] -> w275
              tunnel: w271 -> [w291 w301]
              tunnel: w270 -> [_ w300]
              tunnel: w269 -> [w290 _]
              tunnel: w268 -> [w288 w298]
              tunnel: [w285 w298] -> w267
              tunnel: w261 -> [w284 w299]
              tunnel: [w283 w299] -> w266
              tunnel: w265 -> [_ w297]
              frame "Off", Default {
                n65 = for {
                  tunnel: w291 -> [w292] mode=indexing
                  tunnel: w288 -> [w296]
                  tunnel: [w293] -> w285
                  shift-right: [w294] -> w286
                  shift-left: w287 -> [w295]
                  n66 = VISA Write(VISA resource name=w296, write buffer=w292, error in (no error)=w295) -> (VISA resource name out=w293:refnum<visa-resource-name>, error out=w294:errorcluster)  [unwired: 1 out]
                }
                n67 = Bundle By Name(cluster=w284, "LightCamSeqTriggerCount"=0) -> (w283:T3)
                n68 = Flush Event Queue(0:w290, 3:w286) -> (11:w289:errorcluster)  [unwired: 4 in, 2 out]
              }
              frame "On" {
                n69 = for {
                  tunnel: w301 -> [w305] mode=indexing
                  tunnel: w300 -> [w307]
                  shift-right: [w308] -> w302
                  shift-left: w303 -> [w306]
                  tunnel: w297 -> [w304]
                  n70 = Wait (ms)(milliseconds to wait=w304) -> ()  [unwired: 1 out]
                  n71 = Generate User Event(user event=w307, event data cluster=w305, error in=w306) -> (error out=w308:errorcluster)  [unwired: 1 in, 1 out]
                }
              }
            }
            n72 = call <vilib>:"Build State String with Arguments__JKI_lib_State_Machine.vi"("Arguments (\"\")"=w260, "State"="Wait") -> ("State with Arguments"=w258:string)  [unwired: 4 in]
            n73 = call <vilib>:"Add State(s) to Queue__JKI_lib_State_Machine.vi"("State(s) in Front (\"\")"=w258, "State(s) in (\"\")"=w278) -> ("States Out"=w277:string)  [unwired: 13 in]
          }
          event User Event {
            n74 = event-data() -> ("Write to Arduino"=w321:string)  [unwired: 1 in]
            n75 = Unbundle By Name(w316) -> ("Write to Arduino"=w319:refnum<user-event>)
            n76 = in-place {
              in-place-border: [w334] -> w314
              n77 = in-place-cluster #3(w315) -> ("LightCamSeqTriggerCount"=w335:i32, "MIParameters.DelayValuesInms.Strobing"=w334:i32)
              "LightCamSeqTriggerCount" <- w335
              n78 = Increment(x=w335) -> (x+1=w336:i32)
              n79 = in-place-cluster #3("LightCamSeqTriggerCount"=w336, "MIParameters.DelayValuesInms.Strobing"=w334) -> (w313:T3)
            }
            n80 = VISA Write(VISA resource name=w324, write buffer=w321, error in (no error)=w323) -> (VISA resource name out=w322:refnum<visa-resource-name>, error out=w317:errorcluster)  [unwired: 1 out]
            n81 = flat-sequence {
              tunnel: [w338] -> w318
              tunnel: w317 -> [w338]
              tunnel: w314 -> [w337]
              frame #0 {
                n82 = Wait (ms)(milliseconds to wait=w337) -> ()  [unwired: 1 out]
              }
            }
            n83 = case shown="\"Continuous\"" w312 {
              selector: w312 -> [_ w329]
              tunnel: w321 -> [_ w333]
              tunnel: [w328 w332] -> w320
              tunnel: w319 -> [_ w331]
              tunnel: w318 -> [w328 w330]
              tunnel: ["" w329] -> w310
              frame "OneShot", Default {
              }
              frame "Continuous" {
                n84 = Generate User Event(user event=w331, event data cluster=w333, error in=w330) -> (error out=w332:errorcluster)  [unwired: 1 in, 1 out]
              }
            }
            n85 = call <vilib>:"Build State String with Arguments__JKI_lib_State_Machine.vi"("Arguments (\"\")"=w310, "State"="Wait" ("State(s) in Front (\"\")")) -> ("State with Arguments"=w309:string)  [unwired: 4 in]
            n86 = call <vilib>:"Add State(s) to Queue__JKI_lib_State_Machine.vi"("State(s) in Front (\"\")"=w309, "State(s) in (\"\")"=w325) -> ("States Out"=w326:string)  [unwired: 13 in]
          }
          event User Event {
            n87 = event-data() -> ("Sensor"=w351:string)  [unwired: 1 in]
            n88 = Unbundle By Name(w346) -> ("MIParameters"=w345:T4, "MI Offline?"=w341:bool)
            n89 = call "Read Enable and Power On Sensor Opcode_MI.vi"("error in (no error)"=w352, "Sensor name"=w351, "MachineInterfaceRecipeOpcodes"=w345) -> ("error out"=w343:errorcluster, "Enable and Power On Sensor Opcodes"=w350:string[])  [unwired: 7 in]
            n90 = call "State wise behavior_MI.vi"("error in (no error)"=w343, "State"="DHBLS", "MIRecipeOpcodes"=w345, "VISA Refnum in"=w340) -> ("error out"=w342:errorcluster, "VISA Refnum out"=w339:refnum<visa-resource-name>)  [unwired: 6 in]
            n91 = for {
              tunnel: w350 -> [w360] mode=indexing
              tunnel: w339 -> [w359]
              tunnel: [w356] -> w349
              shift-right: [w357] -> w347
              shift-left: w342 -> [w358]
              tunnel: w341 -> [w355]
              n92 = case shown="True" w355 {
                tunnel: w360 -> [w365 _]
                tunnel: w359 -> [w364 w367]
                tunnel: w358 -> [w363 w366]
                tunnel: [w362 w366] -> w357
                tunnel: [w361 w367] -> w356
                frame False {
                  n93 = VISA Write(VISA resource name=w364, write buffer=w365, error in (no error)=w363) -> (VISA resource name out=w361:refnum<visa-resource-name>, error out=w362:errorcluster)  [unwired: 1 out]
                }
                frame True {
                }
              }
            }
            n94 = call <vilib>:"Add State(s) to Queue__JKI_lib_State_Machine.vi"("State(s) in (\"\")"=w354) -> ("States Out"=w353:string)  [unwired: 14 in]
          }
          event User Event {
            n95 = event-data() -> ("Part Name"=w370:string)  [unwired: 1 in]
            n96 = Concatenate Strings("PartSelected >> " ("string"), w370) -> (w369:string)
            n97 = call <vilib>:"Add State(s) to Queue__JKI_lib_State_Machine.vi"("State(s) in Front (\"\")"=w369, "State(s) in (\"\")"=w374) -> ("States Out"=w375:string)  [unwired: 13 in]
          }
          event User Event {
            n98 = event-data() -> ("Inspection Status"=w380:string)  [unwired: 1 in]
            n99 = in-place {
              in-place-border: w380 -> [w395]
              in-place-border: [w399] -> w379
              n100 = in-place-cluster #4(w378) -> ("Pass after Pause on Fail"=w398:bool, "State"=w387:string)  [unwired: 1 out]
              n101 = Match Pattern(string=w395, regular expression="_") -> (before substring=w394:string, after substring=w393:string)  [unwired: 1 in, 2 out]
              n102 = case shown="\"Fail\"" w394 {
                selector: w394 -> [w402 w406]
                tunnel: w398 -> [_ w408]
                tunnel: [w402 w407] -> w399
                tunnel: [TRUE FALSE] -> w397
                tunnel: w387 -> [_ w404]
                tunnel: ["Run" w403] -> w386
                frame "Fail" {
                }
                frame "Pass", Default {
                  n103 = case shown="True" w408 {
                    tunnel: [w410 w413] -> w407
                    tunnel: w406 -> [w410 _]
                    tunnel: w404 -> [_ w412]
                    tunnel: ["Run" w411] -> w403
                    frame False {
                    }
                    frame True {
                      n104 = case shown="Default" w412 {
                        selector: w412 -> [w414 _]
                        tunnel: ["Pass" "Pass"] -> w413
                        tunnel: [w414 "Run"] -> w411
                        frame "MasterSample" {
                        }
                        frame Default {
                        }
                      }
                    }
                  }
                }
              }
              n105 = Equal?(x=w393, y="T") -> (x = y?=w391:bool)
              n106 = Select(t=FALSE, s=w391, f=TRUE) -> (s? t:f=w388:bool)
              n107 = in-place-cluster #4("Pass after Pause on Fail"=w397, "DisableRun"=w388, "State"=w386) -> (w377:T3)
            }
            n108 = call <vilib>:"Add State(s) to Queue__JKI_lib_State_Machine.vi"("State(s) in Front (\"\")"=w379, "State(s) in (\"\")"=w383) -> ("States Out"=w384:string)  [unwired: 13 in]
          }
          event User Event {
            n109 = event-data() -> ()  [unwired: 1 in, 1 out]
            n110 = call <vilib>:"Add State(s) to Queue__JKI_lib_State_Machine.vi"("State(s) in Front (\"\")"="Macro: Exit" ("State(s) in Front (\"\")"), "State(s) in (\"\")"=w421) -> ("States Out"=w423:string)  [unwired: 13 in]
          }
          event Panel Close? {
            # "Close Panel button (pressed) Event\n(this executes Macro: Exit to terminate the VI)"
            n111 = event-data() -> ()  [unwired: 1 in, 1 out]
            n112 = call <vilib>:"Add State(s) to Queue__JKI_lib_State_Machine.vi"("State(s) in Front (\"\")"="Macro: Exit", "State(s) in (\"\")"=w432) -> ("States Out"=w431:string)  [unwired: 13 in]
            n113 = event-data("Discard?"=TRUE) -> ()  [unwired: 1 in, 1 out]
          }
          event "OK": Value Change {
            # "Exit Button Value Change (pressed) Event\n(this executes Macro: Exit to terminate the VI)"
            n114 = event-data() -> ()  [unwired: 1 in, 1 out]
            n115 = call <vilib>:"Add State(s) to Queue__JKI_lib_State_Machine.vi"("State(s) in Front (\"\")"="Macro: Exit", "State(s) in (\"\")"=w439) -> ("States Out"=w438:string)  [unwired: 13 in]
          }
          event "State Message from Inspection Statemachine": Value Change {
            n116 = event-data() -> ()  [unwired: 1 in, 2 out]
            n117 = Unbundle By Name(w440) -> ("State Message from Inspection Statemachine"=w447:refnum<user-event>)
            n118 = Generate User Event(user event=w447, event data cluster="State Message from Inspection Statemachine", error in=w446) -> (error out=w445:errorcluster)  [unwired: 1 in, 1 out]
            n119 = call <vilib>:"Add State(s) to Queue__JKI_lib_State_Machine.vi"("State(s) in (\"\")"=w442) -> ("States Out"=w441:string)  [unwired: 14 in]
          }
          event "Part Name": Value Change {
            n120 = event-data() -> ("NewVal"=w453:string)  [unwired: 1 in]
            n121 = Unbundle By Name(w449) -> ("Part Name"=w454:refnum<user-event>)
            n122 = Generate User Event(user event=w454, event data cluster=w453, error in=w452) -> (error out=w451:errorcluster)  [unwired: 1 in, 1 out]
            n123 = call <vilib>:"Add State(s) to Queue__JKI_lib_State_Machine.vi"("State(s) in (\"\")"=w455) -> ("States Out"=w456:string)  [unwired: 14 in]
          }
          event "Inspection Status": Value Change {
            n124 = event-data() -> ()  [unwired: 1 in, 1 out]
            n125 = Unbundle By Name(w458) -> ("Inspection Status"=w460:refnum<user-event>)
            n126 = Generate User Event(user event=w460, event data cluster="Inspection Status", error in=w463) -> (error out=w462:errorcluster)  [unwired: 1 in, 1 out]
            n127 = call <vilib>:"Add State(s) to Queue__JKI_lib_State_Machine.vi"("State(s) in (\"\")"=w464) -> ("States Out"=w465:string)  [unwired: 14 in]
          }
        }
      }
      frame "---------- Core ----------" {
        # "Do not put any code in this frame.\n(It is a separator no-op. You can make a copy of this frame to create a new Data frame)"
        n128 = call <vilib>:"Add State(s) to Queue__JKI_lib_State_Machine.vi"("State(s) in (\"\")"=w472) -> ("States Out"=w471:string)  [unwired: 14 in]
      }
      frame Default {
        w484 = 42 items=["No error", "Argument error", "Memory is full", "Out of zone", "End of file", "File already open", "Generic file I/O error", "File not found", "File permission error", "Disk is full", "Duplicate path", "Too many files open", "System feature not enabled", "Resource file not found", "Cannot add resource", "Resource not found", "Image not found", "Image memory error", "Pen does not exist", "Config type invalid", "Config token not found", "Config parse error", "Config memory error", "Bad external code format", "Bad external code offset", "External code not present", "Null window", "Destroy window error", "Null menu", "Print aborted", "Bad print record", "Print driver error", "Windows error during printing", "Memory error during printing", "Print dialog error", "Generic print error", "Invalid device refnum", "Device not found", "Device parameter error", "Device unit error", "Cannot open device", "Device call aborted", "Generic error", "Cancelled by user", "Object ID too low", "Object ID too high", "Object not in heap", "Unknown heap", "Unknown object (invalid DefProc)", "Unknown object (DefProc not in table)", "Message out of range", "Invalid (null) method", "Unknown message", "Manager call not supported", "Bad address", "Network operation in progress", "Network operation timed out", "Connection is busy", "Network attribute not supported", "Network error", "Address in use", "System out of memory", "Connection aborted", "Connection refused", "Not connected", "Already connected", "Connection closed", "Initialization error (interapplication manager)", "Bad occurrence", "Wait on unbound occurrence handler", "Occurrence queue overflow", "Datalog type conflict", "Unused", "Unrecognized type (interapplication manager)", "Memory corrupt", "Failed to make temporary DLL", "Old CIN version", "Drag socket not found", "Failed to load drop-object", "Failed to register OLE object", "Failed to release OLE object", "Format specifier type mismatch", "Unknown format specifier", "Too few format specifiers", "Too many format specifiers", "Scan failed", "Newer CIN version", "Error converting to variant", "Runtime menu error", "Password tampered", "Variant attribute not found", "Incompatible variant data type", "Event data is not available", "Event Store is not present", "Occurrence is not found", "Event Queue is not created", "Event info is not available", "Refnum passed is NULL", "Error retrieving Class GUID", "Error retrieving CoClass GUID", "Error retrieving TypeLib GUID.", "Bad built application magic bytes.", "Specific driver is different from the specific driver associated with the Logical Name.", "There is no session opened to the class driver.", "Max Error", "MAX - Error with config objects", "MAX - Error loading configuration", "MAX - Group not supported"]
        # "Current State"
        # "Do not delete, rename, or modify this frame.\n(this is used to capture unhandled states and typos)"
        # "Handle mistyped state name (developer tool)"
        n129 = Format Into String(format string="Software Exception: Unhandled State \"%s\"." ("message"), error in=w480, w475) -> (resulting string=w483:string, error out=w482:errorcluster)  [unwired: 1 in]
        n130 = call <vilib>:"Error Cluster From Error Code.vi"("show call chain? (False)"=TRUE, "error in (no error)"=w482, "error message (\"\")"=w483, "error code (0)"=w484) -> ("error out"=w481:errorcluster)  [unwired: 5 in]
        n131 = call <vilib>:"Add State(s) to Queue__JKI_lib_State_Machine.vi"("State(s) in (\"\")"=w479) -> ("States Out"=w478:string)  [unwired: 14 in]
      }
      frame "Initialize Core Data" {
        # "Do not delete, rename, or modify this frame.\n(this is used to determine panel behavior on exit)"
        # "originally closed?"
        # "exe?"
        # "If panel starts closed or is an EXE, then close it when we exit"
        n132 = property class="VI"() -> ("Front Panel.Open"=w495:bool)  [unwired: 2 in, 2 out]
        n133 = property class="App"() -> ("App.Kind"=w494:T9)  [unwired: 2 in, 2 out]
        n134 = control-ref of="Current VI Reference"() -> (w489:refnum<vi>)
        n135 = Not(x=w495) -> (.not. x?=w492:bool)
        n136 = Equal?(x=w494, y=T9."Run Time System" ("Application:Kind")) -> (x = y?=w491:bool)
        n137 = Or(x=w492, y=w491) -> (x .or. y?=w487:bool)
        n138 = Bundle By Name(cluster=w490, "Core.Current VI Reference"=w489, "Core.Close Panel on Exit?"=w487) -> (w497:T3)
        n139 = call <vilib>:"Add State(s) to Queue__JKI_lib_State_Machine.vi"("State(s) in (\"\")"=w499) -> ("States Out"=w498:string)  [unwired: 14 in]
      }
      frame "Error Handler" {
        # "Handle any errors here.\nYou can also output any states to clean-up after errors occur"
        n140 = Unbundle By Name(w503) -> ("Output Cluster_MI"=w502:T5)
        n141 = case shown="Error" w504 {
          selector: w504 -> [_ w515]
          tunnel: w501 -> [w510 w514]
          tunnel: w502 -> [_ w512]
          tunnel: [w510 w511] -> w500
          frame No Error {
          }
          frame Error {
            n142 = Unbundle By Name(w515) -> ("code"=w513:i32)
            n143 = case shown="91" w513 {
              selector: w513 -> [w524 w533 w540 w549 w558 _ _]
              tunnel: w514 -> [w518 w528 w536 w544 w554 w563 w569]
              tunnel: w512 -> [w517 w527 w537 w545 w555 w564 w570]
              tunnel: [w516 w525 w534 w543 w552 w561 w567] -> w511
              frame Default {
                # "Unknown Error"
                n144 = Number To Decimal String(number=w524) -> (decimal integer string=w522:string)  [unwired: 1 in]
                n145 = Concatenate Strings("0x03000105_", w522) -> (w519:string)
                n146 = Bundle By Name(cluster=w517, "Error Message"=w519) -> (w521:T5)
                n147 = call "Output_MI.vi"("Machine Interface Actor in"=w518, "Output Cluster_MI"=w521, "State"="ErrorMessage") -> ("Machine Interface Actor out"=w516:refnum<class "Machine Interface.lvclass">)  [unwired: 11 in, 1 out]
              }
              frame -1073807346 {
                # "The given session or object reference is invalid"
                n148 = Number To Decimal String(number=w533) -> (decimal integer string=w532:string)  [unwired: 1 in]
                n149 = Concatenate Strings("ArduinoDisconnection_0x03000104", w532) -> (w526:string)
                n150 = Bundle By Name(cluster=w527, "Error Message"=w526) -> (w530:T5)
                n151 = call "Output_MI.vi"("Machine Interface Actor in"=w528, "Output Cluster_MI"=w530, "State"="ErrorMessage") -> ("Machine Interface Actor out"=w525:refnum<class "Machine Interface.lvclass">)  [unwired: 11 in, 1 out]
              }
              frame -1073807339 {
                # "Timeout expired before operation completed"
                n152 = Number To Decimal String(number=w540) -> (decimal integer string=w542:string)  [unwired: 1 in]
                n153 = Concatenate Strings("ArduinoError_0x03000106", w542) -> (w535:string)
                n154 = Bundle By Name(cluster=w537, "Error Message"=w535) -> (w539:T5)
                n155 = call "Output_MI.vi"("Machine Interface Actor in"=w536, "Output Cluster_MI"=w539, "State"="ErrorMessage") -> ("Machine Interface Actor out"=w534:refnum<class "Machine Interface.lvclass">)  [unwired: 11 in, 1 out]
              }
              frame -1073807246 {
                # "The resource is valid, but VISA cannot currently access it"
                n156 = Number To Decimal String(number=w549) -> (decimal integer string=w551:string)  [unwired: 1 in]
                n157 = Concatenate Strings("ArduinoError_0x03000107", w551) -> (w546:string)
                n158 = Bundle By Name(cluster=w545, "Error Message"=w546) -> (w548:T5)
                n159 = call "Output_MI.vi"("Machine Interface Actor in"=w544, "Output Cluster_MI"=w548, "State"="ErrorMessage") -> ("Machine Interface Actor out"=w543:refnum<class "Machine Interface.lvclass">)  [unwired: 11 in, 1 out]
              }
              frame -1073807194 {
                # "The connection for the given session has been lost"
                n160 = Number To Decimal String(number=w558) -> (decimal integer string=w560:string)  [unwired: 1 in]
                n161 = Concatenate Strings("ArduinoError_0x03000108", w560) -> (w553:string)
                n162 = Bundle By Name(cluster=w555, "Error Message"=w553) -> (w557:T5)
                n163 = call "Output_MI.vi"("Machine Interface Actor in"=w554, "Output Cluster_MI"=w557, "State"="ErrorMessage") -> ("Machine Interface Actor out"=w552:refnum<class "Machine Interface.lvclass">)  [unwired: 11 in, 1 out]
              }
              frame 3000001 {
                # "MI Software is not compatible"
                n164 = Bundle By Name(cluster=w564, "Error Message"="0x03000001") -> (w566:T5)
                n165 = call "Output_MI.vi"("Machine Interface Actor in"=w563, "Output Cluster_MI"=w566, "State"="ErrorMessage") -> ("Machine Interface Actor out"=w561:refnum<class "Machine Interface.lvclass">)  [unwired: 11 in, 1 out]
              }
              frame 91 {
                # "Variant To Data conversion error"
                n166 = Bundle By Name(cluster=w570, "Error Message"="0x03000002") -> (w572:T5)
                n167 = call "Output_MI.vi"("Machine Interface Actor in"=w569, "Output Cluster_MI"=w572, "State"="ErrorMessage") -> ("Machine Interface Actor out"=w567:refnum<class "Machine Interface.lvclass">)  [unwired: 11 in, 1 out]
              }
            }
          }
        }
        n168 = call <vilib>:"Add State(s) to Queue__JKI_lib_State_Machine.vi"("State(s) in Front (\"\")"="/* Post Error States", "State(s) in (\"\")"=w509) -> ("States Out"=w508:string)  [unwired: 13 in]
      }
      frame "Exit" {
        # "Do not put any code in this frame.\n(No errors that occur here will be handled.)"
        n169 = call <vilib>:"Add State(s) to Queue__JKI_lib_State_Machine.vi"("State(s) in (\"\")"=w579) -> ("States Out"=w578:string)  [unwired: 14 in]
      }
      frame "---------- Data ----------" {
        # "Do not put any code in this frame.\n(It is a separator no-op. You can make a copy of this frame to create a new Data frame)"
        n170 = call <vilib>:"Add State(s) to Queue__JKI_lib_State_Machine.vi"("State(s) in (\"\")"=w585) -> ("States Out"=w584:string)  [unwired: 14 in]
      }
      frame "Data: Initialize" {
        w588 = "UI: Front Panel State >> Close"  # UI: Front Panel State >> Close
        w589 = "UI: Front Panel State >> Open"  # UI: Front Panel State >> Open
        w594 = T5 {"Acknowledgement"={"Enqueuer"=refnum, "VIReference"=refnum, "VIName"=""}, "Diagnostics Result"={"Result"=FALSE, "StateMessage"=""}, "Message to SM"="", "Button Press"="", "Error Message"="", "Loading bar cluster"={"Pop-up Type"=enum."Open Logo Display", "Title"="", "Message"="", "Button 1 Text"="", "Button 2 Text"="", "Show Close? T/F"=FALSE, "Title Blink? T/F"=FALSE, "Title Blink Colour"=0}}  # Output Cluster_MI
        w593 = T3 {"Timeout"=0, "Core"={"Current VI Reference"=refnum, "Close Panel on Exit?"=FALSE}, "MIParameters"={"SpecificationVersion"="", "CompatibleSoftwareVersions"=[], "FrontPanelOpen"=FALSE, "DelayValuesInms"={"TimingUnitSetup"=0, "Strobing"=0, "TowerLampDiagnostics"=0, "Run"=0, "DisableSensors"=0}, "HardwareConfigurationParameters"={"BaudRate"=0.0}, "MIRecipeOpcodes"={"DeviceReadiness"={"Ping"=[], "PingResponse"=[]}, "Initialization"=[], "MachinePowerStatus"={"MachinePowerStatusCheck"=[], "MachinePowerStatusResponse"=[]}, "DoorLockStatus"={"DoorLockStatusCheck"=[], "DoorLockStatusResponse"=[], "Enable"=[], "Disable"=[]}, "OpenLimitSwitchStatus"=[], "MotorDiagnostics"=[], "HardwareButtonDiagnostics"={"Run"=[], "Pause"=[], "Stop"=[], "BuzzerOff"=[]}, "TriggerLightCameraSequence"=[], "SensorDiagnostics"=[], "TowerLampDiagnostics"={"RedLamp"=[], "YellowLamp"=[], "GreenLamp"=[], "Buzzer"=[]}, "Select"=[], "Run"={"HardwareButtonStatus"=[], "Pass"={"TowerLampStatus"=[]}}, "Pause"={"PauseButtonPress"=[], "Fail"=[], "BuzzerOffButtonPress"=[]}, "Exit"={"Shutdown"=[]}, "DHBLS"=[], "PartsList"=[], "HardwareButtonPressed"={"RunButtonPress"=[], "PauseButtonPress"=[], "StopButtonPress"=[], "BuzzerOffButtonPress"=[], "DoorUnlock"=[]}, "ReadyPositionReached"=[], "IncorrectOpcode"=[]}}, "Number of Racks"=0, "First Call?"=FALSE, "Message to SM on Timeout"="", "Message from Hardware"="", "Part details"={"Name"="", "RackDependentOpcodes"=[]}, "State"="", "Ping Response, Button Press, Incorrect Opcode"=[], "Rack1 Response"=[], "Rack2 Response"=[], "LightCamSeqTriggerCount"=0, "Pass after Pause on Fail"=FALSE, "MI Offline?"=FALSE, "Ping Response, Button Press, Incorrect Opcode"={"PingResponse"=[], "MachinePowerStatusResponse"=[], "HWRunButtonPress"=[], "HWPauseButtonPress"=[], "HWStopButtonPress"=[], "HWBuzzerOffButtonPress"=[], "DoorUnlock"=[], "ReadyPositionReached"=[], "IncorrectOpcode"=[], "DoorLockStatusResponse"=[]}, "Rack1 Response"={"LimitSwitchStatusResponse"=[], "GuideOpenResponse"=[], "GuideCloseResponse"=[]}, "Rack2 Response"={"LimitSwitchStatusResponse"=[], "GuideOpenResponse"=[], "GuideCloseResponse"=[]}, "Output Cluster_MI"={"Acknowledgement"={"Enqueuer"=refnum, "VIReference"=refnum, "VIName"=""}, "Diagnostics Result"={"Result"=FALSE, "StateMessage"=""}, "Message to SM"="", "Button Press"="", "Error Message"="", "Loading bar cluster"={"Pop-up Type"=enum."Open Logo Display", "Title"="", "Message"="", "Button 1 Text"="", "Button 2 Text"="", "Show Close? T/F"=FALSE, "Title Blink? T/F"=FALSE, "Title Blink Colour"=0}}, "DisableRun"=FALSE}  # Local Data_MI
        w598 = T12 {"Name"="", "RackDependentOpcodes"=[]}  # Part details
        w600 = FALSE  # Pass after Pause on Fail
        w606 = 0  # LightCamSeqTriggerCount
        w607 = ""  # State
        w612 = ""  # Message from Hardware
        w613 = ""  # Message to SM on Timeout
        w614 = TRUE  # First Call?
        w586 = -1  # Timeout
        # "Initialize the shift-register data, here.\n(data names are defined by what you wire into the bundle function)"
        n171 = Unbundle By Name(w605) -> ("Machine Interface Parameters File Path"=w601:path)
        n172 = call "Read Machine Interface Opcodes_MI.vi"("error in (no error)"=w602, "Machine Interface Parameters File Path"=w601) -> ("error out"=w592:errorcluster, "MachineInterfaceParameters"=w591:T4)  [unwired: 7 in]
        n173 = call "Arduino Response List_MI.vi"("MachineInterfaceRecipeOpcodes"=w591) -> ("Number of Racks"=w604:i32, "Rack2 Response"=w595:T2, "Rack1 Response"=w596:T2, "Ping Response, Button Press, Incorrect Opcode"=w597:T1)  [unwired: 7 in]
        "Number of Racks" <- w604
        "Ping Response, Button Press, Incorrect Opcode" <- w597
        "Rack1 Response" <- w596
        "Rack2 Response" <- w595
        n174 = Unbundle By Name(w591) -> ("FrontPanelOpen"=w590:bool)
        n175 = property on="Ping Response, Button Press, Incorrect Opcode" class="Clust (strict)"() -> ("Controls[]"=w608:refnum<vi>[])  [unwired: 2 in, 2 out]
        n176 = property on="Rack1 Response" class="Clust (strict)"() -> ("Controls[]"=w609:refnum<vi>[])  [unwired: 2 in, 2 out]
        n177 = property on="Rack2 Response" class="Clust (strict)"() -> ("Controls[]"=w610:refnum<vi>[])  [unwired: 2 in, 2 out]
        n178 = Select(t=w589, s=w590, f=w588) -> (s? t:f=w587:string)
        n179 = Bundle(cluster=w593, "Timeout"=w586, "Core"=T10 {"Current VI Reference"=refnum, "Close Panel on Exit?"=FALSE}, "MIParameters"=w591, "Number of Racks"=w604, "First Call?"=w614, "Message to SM on Timeout"=w613, "Message from Hardware"=w612, "Part details"=w598, "State"=w607, "Ping Response, Button Press, Incorrect Opcode"=w608, "Rack1 Response"=w609, "Rack2 Response"=w610, "LightCamSeqTriggerCount"=w606, "Pass after Pause on Fail"=w600, "MI Offline?"="MI Offline?", "Ping Response, Button Press, Incorrect Opcode"=w597, "Rack1 Response"=w596, "Rack2 Response"=w595, "Output Cluster_MI"=w594) -> (w615:T3)  [unwired: 1 in]
        n180 = call <vilib>:"Add State(s) to Queue__JKI_lib_State_Machine.vi"("State(s) in (\"\")"=w617, "State(s) at Back (\"\")"=w587) -> ("States Out"=w616:string)  [unwired: 13 in]
      }
      frame "Data: Cleanup" {
        # "Cleanup any data and references, here.\n(this is called automatically, by the Macro: Exit)"
        n181 = Unbundle By Name(w646) -> ("Core.Current VI Reference"=w648:refnum<vi>)
        n182 = Unbundle By Name(w621) -> ("Sensor Name"=w620:refnum<user-event>, "State Message from Inspection Statemachine"=w645:refnum<user-event>, "Message from Arduino"=w644:refnum<user-event>, "Trigger Light Camera Sequence"=w643:refnum<user-event>, "Write to Arduino"=w642:refnum<user-event>, "Part Name"=w641:refnum<user-event>, "Inspection Status"=w640:refnum<user-event>, "VISA resource"=w639:refnum<user-event>, "Stop Arduino Rx Loop"=w630:refnum<user-event>)
        n183 = VISA Flush I/O Buffer(VISA resource name=w624, error in (no error)=w623) -> (VISA resource name out=w627:refnum<visa-resource-name>, error out=w626:errorcluster)  [unwired: 1 in]
        n184 = case shown="No Error" w626 {
          selector: w626 -> [w652 _]
          tunnel: [w651 errorcluster {"status"=FALSE, "code"=0, "source"=""} ("error constant")] -> w628
          tunnel: w627 -> [w653 _]
          frame No Error {
            n185 = VISA Close(VISA resource name=w653, error in (no error)=w652) -> (error out=w651:errorcluster)
          }
          frame Error {
          }
        }
        n186 = Generate User Event(user event=w630, event data cluster=TRUE, error in=w628) -> (error out=w629:errorcluster)  [unwired: 1 in, 1 out]
        n187 = Unregister For Events(event registration refnum=w622, error in=w629) -> (error out=w619:errorcluster)
        n188 = Destroy User Event(user event=w645, error in=w619) -> (error out=w638:errorcluster)
        n189 = Destroy User Event(user event=w644, error in=w619) -> (error out=w637:errorcluster)
        n190 = Destroy User Event(user event=w643, error in=w619) -> (error out=w636:errorcluster)
        n191 = Destroy User Event(user event=w642, error in=w619) -> (error out=w635:errorcluster)
        n192 = Destroy User Event(user event=w641, error in=w619) -> (error out=w634:errorcluster)
        n193 = Destroy User Event(user event=w640, error in=w619) -> (error out=w633:errorcluster)
        n194 = Destroy User Event(user event=w639, error in=w619) -> (error out=w632:errorcluster)
        n195 = Destroy User Event(user event=w620, error in=w619) -> (error out=w618:errorcluster)
        n196 = Merge Errors(w618, w638, w637, w636, w635, w634, w633, w632) -> (w625:errorcluster)
        n197 = Close Reference(reference=w648, error in (no error)=w625) -> (error out=w647:errorcluster)
        n198 = call <vilib>:"Add State(s) to Queue__JKI_lib_State_Machine.vi"("State(s) in (\"\")"=w650) -> ("States Out"=w649:string)  [unwired: 14 in]
      }
      frame "---------- UI ----------" {
        # "Do not put any code in this frame.\n(It is a separator no-op. You can make a copy of this frame to create a new UI frame)"
        n199 = call <vilib>:"Add State(s) to Queue__JKI_lib_State_Machine.vi"("State(s) in (\"\")"=w660) -> ("States Out"=w659:string)  [unwired: 14 in]
      }
      frame "UI: Initialize" {
        # "Initialize the User Interface, here.\n(this is called automatically, by the Macro: Init)"
        n200 = call <vilib>:"Add State(s) to Queue__JKI_lib_State_Machine.vi"("State(s) in (\"\")"=w666) -> ("States Out"=w665:string)  [unwired: 14 in]
      }
      frame "UI: Front Panel State" {
        # "Argument"
        # "Set Front Panel Open or Closed\n(Usage: \"UI: Front Panel State >> Open|Close\")"
        n201 = Unbundle By Name(w671) -> ("Core.Current VI Reference"=w670:refnum<vi>)
        n202 = case shown="\"Close\"" w669 {
          tunnel: w673 -> [w679 w692]
          tunnel: [w681 w693] -> w672
          tunnel: w670 -> [w680 w690]
          frame "Open", Default {
            n203 = property class="VI"(reference=w680, error in=w679) -> (reference out=w677:refnum<vi>, error out=w678:errorcluster, "Front Panel.Open"=w676:bool)
            n204 = case shown="False" w676 {
              tunnel: [w684 w687] -> w681
              tunnel: w678 -> [w683 w687]
              tunnel: w677 -> [w682 _]
              frame False {
                n205 = invoke class="VI" method="FP.Open"(reference=w682, error in=w683, "Activate"=TRUE, "State"=T11."Standard") -> (error out=w684:errorcluster)  [unwired: 1 in, 4 out]
              }
              frame True {
              }
            }
          }
          frame "Close" {
            n206 = property class="VI"(reference=w690, error in=w692) -> (reference out=w689:refnum<vi>, error out=w691:errorcluster, "Front Panel.Open"=w688:bool)
            n207 = case shown="True" w688 {
              tunnel: [w694 w697] -> w693
              tunnel: w691 -> [w694 w696]
              tunnel: w689 -> [_ w695]
              frame False {
              }
              frame True {
                n208 = invoke class="VI" method="FP.Close"(reference=w695, error in=w696) -> (error out=w697:errorcluster)  [unwired: 1 in, 2 out]
              }
            }
          }
        }
        n209 = call <vilib>:"Add State(s) to Queue__JKI_lib_State_Machine.vi"("State(s) in (\"\")"=w675) -> ("States Out"=w674:string)  [unwired: 14 in]
      }
      frame "---------- Macro ----------" {
        # "Do not put any code in this frame.\n(It is a separator )"
        n210 = call <vilib>:"Add State(s) to Queue__JKI_lib_State_Machine.vi"("State(s) in (\"\")"=w703) -> ("States Out"=w702:string)  [unwired: 14 in]
      }
      frame "Macro: Initialize" {
        # "Initialization Macro\n(This is called once, when the VI starts)"
        n211 = control-ref of="This VI"() -> (w710:refnum<vi>)
        n212 = call <vilib>:"Read Self Enqueuer.vi"("Actor"=w705) -> ("Self Enqueuer"=w711:refnum<class "Message Enqueuer.lvclass">)  [unwired: 10 in]
        n213 = Unbundle By Name(w709) -> ("Output Cluster_MI"=w708:T5)
        n214 = Bundle By Name(cluster=w708, "Acknowledgement.Enqueuer"=w711, "Acknowledgement.VIReference"=w710) -> (w707:T5)
        n215 = call "Output_MI.vi"("Machine Interface Actor in"=w705, "Output Cluster_MI"=w707, "State"="Acknowledgement", "error in (no error)"=w713) -> ("Machine Interface Actor out"=w704:refnum<class "Machine Interface.lvclass">, "error out"=w712:errorcluster)  [unwired: 10 in]
        n216 = call <vilib>:"Add State(s) to Queue__JKI_lib_State_Machine.vi"("State(s) in Front (\"\")"="Data: Initialize\nInitialize Core Data\nUI: Initialize", "State(s) in (\"\")"=w717) -> ("States Out"=w716:string)  [unwired: 13 in]
      }
      frame "Macro: Exit" {
        # "Exit Macro\n(This is called once, when the VI exits)"
        n217 = Unbundle By Name(w721) -> ("Core.Close Panel on Exit?"=w727:bool)
        n218 = Select(t="UI: Front Panel State >> Close", s=w727, f="") -> (s? t:f=w724:string)
        n219 = call <vilib>:"Add State(s) to Queue__JKI_lib_State_Machine.vi"("State(s) in (\"\")"=w724, "State(s) at Back (\"\")"="Data: Cleanup\nExit") -> ("States Out"=w722:string)  [unwired: 13 in]
        n220 = call <vilib>:"Add State(s) to Queue__JKI_lib_State_Machine.vi"("State(s) in Front (\"\")"=w722, "State(s) in (\"\")"=w729) -> ("States Out"=w728:string)  [unwired: 13 in]
      }
      frame "---------- Device Readiness State ----------" {
        # "Do not put any code in this frame.\n(It is a separator )"
        n221 = call <vilib>:"Add State(s) to Queue__JKI_lib_State_Machine.vi"("State(s) in (\"\")"=w735) -> ("States Out"=w734:string)  [unwired: 14 in]
      }
      frame "CheckArduinoPort" {
        # "Ping State is added to State-Queue"
        n222 = Unbundle By Name(w742) -> ("Output Cluster_MI"=w739:T5, "MI Offline?"=w741:bool, "MIParameters.HardwareConfigurationParameters.BaudRate"=w740:dbl, "MIParameters.DelayValuesInms.TimingUnitSetup"=w738:i32)
        n223 = case shown="False" w741 {
          tunnel: [w755 w765] -> w748
          tunnel: [w761 refnum<visa-resource-name> refnum ("VISA resource name out")] -> w746
          tunnel: w745 -> [w760 w765]
          tunnel: w740 -> [w753 _]
          tunnel: w738 -> [w752 _]
          frame False {
            # "MI Online"
            n224 = call "Check Arduino Port_MI.vi"("error in (no error)"=w760) -> ("error out"=w758:errorcluster, "VISA Refnum out"=w759:refnum<visa-resource-name>)  [unwired: 7 in, 2 out]
            n225 = VISA Open(error in (no error)=w758, VISA resource name=w759) -> (VISA resource name=w757:refnum<visa-resource-name>, error out=w756:errorcluster)  [unwired: 3 in]
            n226 = call-poly "VISA Configure Serial Port"("VISA resource name"=w757, "baud rate (9600)"=w753, "error in (no error)"=w756) -> ("VISA resource name out"=w761:refnum<visa-resource-name>, "error out"=w754:errorcluster)  [unwired: 11 in]
            "VISA" <- w761
            n227 = flat-sequence {
              tunnel: [w763] -> w755
              tunnel: w754 -> [w763]
              tunnel: w752 -> [w762]
              frame #0 {
                n228 = Wait (ms)(milliseconds to wait=w762) -> ()  [unwired: 1 out]
              }
            }
          }
          frame True {
            # "MI Offline"
          }
        }
        n229 = Unbundle By Name(w737) -> ("VISA resource"=w747:refnum<user-event>)
        n230 = case shown="Error" w748 {
          selector: w748 -> [w774 _]
          tunnel: w747 -> [w775 _]
          tunnel: w746 -> [w773 w783]
          tunnel: [w772 w780] -> w744
          tunnel: [w773 w783] -> w743
          tunnel: w737 -> [w770 w782]
          tunnel: w739 -> [w767 w777]
          tunnel: [w766 w776] -> w736
          frame No Error {
            n231 = Generate User Event(user event=w775, event data cluster=w773, error in=w774) -> (error out=w771:errorcluster)  [unwired: 1 in, 1 out]
            n232 = call "Output_MI.vi"("Machine Interface Actor in"=w770, "Output Cluster_MI"=w767, "State"="DiagnosticsResult", "Sub State"="ComPortAvailable", "error in (no error)"=w771) -> ("Machine Interface Actor out"=w766:refnum<class "Machine Interface.lvclass">, "error out"=w772:errorcluster)  [unwired: 9 in]
          }
          frame Error {
            n233 = call "Output_MI.vi"("Machine Interface Actor in"=w782, "Output Cluster_MI"=w777, "State"="DiagnosticsResult", "Sub State"="ComPortNotAvailable", "error in (no error)"=errorcluster {"status"=FALSE, "code"=0, "source"=""} ("error constant")) -> ("Machine Interface Actor out"=w776:refnum<class "Machine Interface.lvclass">, "error out"=w780:errorcluster)  [unwired: 9 in]
          }
        }
        n234 = call <vilib>:"Add State(s) to Queue__JKI_lib_State_Machine.vi"("State(s) in Front (\"\")"="Wait" ("State(s) in Front (\"\")"), "State(s) in (\"\")"=w751) -> ("States Out"=w750:string)  [unwired: 13 in]
      }
      frame "DeviceReadiness" {
        n235 = call <vilib>:"Add State(s) to Queue__JKI_lib_State_Machine.vi"("State(s) in Front (\"\")"="Ping" ("State(s) in Front (\"\")"), "State(s) in (\"\")"=w790) -> ("States Out"=w789:string)  [unwired: 13 in]
      }
      frame "Ping" {
        # "Wait for Ping Response"
        n236 = Unbundle By Name(w798) -> ("MIParameters"=w795:T4)
        n237 = call "State wise behavior_MI.vi"("error in (no error)"=w797, "State"="Ping", "MIRecipeOpcodes"=w795, "VISA Refnum in"=w792) -> ("error out"=w796:errorcluster, "VISA Refnum out"=w791:refnum<visa-resource-name>)  [unwired: 6 in]
        n238 = Bundle By Name(cluster=w798, "Message to SM on Timeout"="Arduino Not Connected", "Timeout"=5000) -> (w800:T3)
        n239 = call <vilib>:"Add State(s) to Queue__JKI_lib_State_Machine.vi"("State(s) in Front (\"\")"="Wait >> DeviceReadiness" ("State(s) in Front (\"\")"), "State(s) in (\"\")"=w804) -> ("States Out"=w803:string)  [unwired: 13 in]
      }
      frame "PingResponse" {
        n240 = Unbundle By Name(w811) -> ("Output Cluster_MI"=w807:T5)
        n241 = Bundle By Name(cluster=w811, "State"="DeviceReadiness") -> (w814:T3)
        n242 = call "Output_MI.vi"("Machine Interface Actor in"=w806, "Output Cluster_MI"=w807, "State"="DiagnosticsResult", "Sub State"="DeviceReady", "error in (no error)"=w812) -> ("Machine Interface Actor out"=w805:refnum<class "Machine Interface.lvclass">, "error out"=w810:errorcluster)  [unwired: 9 in]
        n243 = call <vilib>:"Add State(s) to Queue__JKI_lib_State_Machine.vi"("State(s) in Front (\"\")"="Wait" ("State(s) in Front (\"\")"), "State(s) in (\"\")"=w818) -> ("States Out"=w817:string)  [unwired: 13 in]
      }
      frame "---------- Initialization State ----------" {
        # "Do not put any code in this frame.\n(It is a separator )"
        n244 = call <vilib>:"Add State(s) to Queue__JKI_lib_State_Machine.vi"("State(s) in (\"\")"=w824) -> ("States Out"=w823:string)  [unwired: 14 in]
      }
      frame "Initialization" {
        n245 = Unbundle By Name(w833) -> ("MIParameters"=w831:T4)
        n246 = call "State wise behavior_MI.vi"("error in (no error)"=w829, "State"="Initialization", "MIRecipeOpcodes"=w831, "VISA Refnum in"=w826) -> ("error out"=w828:errorcluster, "VISA Refnum out"=w827:refnum<visa-resource-name>)  [unwired: 6 in]
        n247 = call "State wise behavior_MI.vi"("error in (no error)"=w828, "State"="DHBLS", "MIRecipeOpcodes"=w831, "VISA Refnum in"=w827) -> ("error out"=w832:errorcluster, "VISA Refnum out"=w825:refnum<visa-resource-name>)  [unwired: 6 in]
        n248 = call <vilib>:"Add State(s) to Queue__JKI_lib_State_Machine.vi"("State(s) in Front (\"\")"="Wait" ("State(s) in Front (\"\")"), "State(s) in (\"\")"=w838) -> ("States Out"=w837:string)  [unwired: 13 in]
      }
      frame "---------- Machine Power Status Check State----------" {
        # "Do not put any code in this frame.\n(It is a separator )"
        n249 = call <vilib>:"Add State(s) to Queue__JKI_lib_State_Machine.vi"("State(s) in (\"\")"=w844) -> ("States Out"=w843:string)  [unwired: 14 in]
      }
      frame "MachinePowerStatusCheck" {
        # "Wait for MachinePowerStatusResponse"
        n250 = Unbundle By Name(w848) -> ("MIParameters"=w851:T4)
        n251 = call "State wise behavior_MI.vi"("error in (no error)"=w853, "State"="MachinePowerStatusCheck", "MIRecipeOpcodes"=w851, "VISA Refnum in"=w846) -> ("error out"=w852:errorcluster, "VISA Refnum out"=w845:refnum<visa-resource-name>)  [unwired: 6 in]
        n252 = Bundle By Name(cluster=w848, "Timeout"=5000) -> (w847:T3)
        n253 = call <vilib>:"Add State(s) to Queue__JKI_lib_State_Machine.vi"("State(s) in Front (\"\")"="Wait >> MachinePowerStatus" ("State(s) in Front (\"\")"), "State(s) in (\"\")"=w857) -> ("States Out"=w856:string)  [unwired: 13 in]
      }
      frame "MachinePowerStatusResponse" {
        n254 = Unbundle By Name(w861) -> ("Output Cluster_MI"=w860:T5, "Message from Hardware"=w865:string)
        n255 = String Subset(string=w865, offset (0)=4, length (rest)=1 ("length (rest)")) -> (substring=w862:string)
        n256 = case shown="\"1\"" w862 {
          tunnel: w867 -> [w880 w887]
          tunnel: [w879 w886] -> w866
          tunnel: w859 -> [w876 w885]
          tunnel: w860 -> [w875 w882]
          tunnel: [w874 w881] -> w858
          frame Default {
            # "Machine not powered ON"
            n257 = call "Output_MI.vi"("Machine Interface Actor in"=w876, "Output Cluster_MI"=w875, "State"="DiagnosticsResult", "Sub State"="MachineNotPoweredON", "error in (no error)"=w880) -> ("Machine Interface Actor out"=w874:refnum<class "Machine Interface.lvclass">, "error out"=w879:errorcluster)  [unwired: 9 in]
          }
          frame "1" {
            # "Machine Powered ON"
            n258 = call "Output_MI.vi"("Machine Interface Actor in"=w885, "Output Cluster_MI"=w882, "State"="DiagnosticsResult", "Sub State"="MachinePoweredOn", "error in (no error)"=w887) -> ("Machine Interface Actor out"=w881:refnum<class "Machine Interface.lvclass">, "error out"=w886:errorcluster)  [unwired: 9 in]
          }
        }
        n259 = Bundle By Name(cluster=w861, "State"="MachinePowerStatus") -> (w869:T3)
        n260 = call <vilib>:"Add State(s) to Queue__JKI_lib_State_Machine.vi"("State(s) in Front (\"\")"="Wait" ("State(s) in Front (\"\")"), "State(s) in (\"\")"=w873) -> ("States Out"=w872:string)  [unwired: 13 in]
      }
      frame "---------- Door Lock Status Check ----------" {
        # "Do not put any code in this frame.\n(It is a separator )"
        n261 = call <vilib>:"Add State(s) to Queue__JKI_lib_State_Machine.vi"("State(s) in (\"\")"=w893) -> ("States Out"=w892:string)  [unwired: 14 in]
      }
      frame "DoorLockStatusCheck" {
        n262 = Unbundle By Name(w896) -> ("MIParameters"=w900:T4)
        n263 = call "State wise behavior_MI.vi"("error in (no error)"=w898, "State"="DoorLockStatusCheck", "MIRecipeOpcodes"=w900, "VISA Refnum in"=w895) -> ("error out"=w897:errorcluster, "VISA Refnum out"=w894:refnum<visa-resource-name>)  [unwired: 6 in]
        n264 = call <vilib>:"Add State(s) to Queue__JKI_lib_State_Machine.vi"("State(s) in (\"\")"=w903) -> ("States Out"=w902:string)  [unwired: 14 in]
      }
      frame "DoorLockStatusResponse" {
        n265 = Unbundle By Name(w910) -> ("Output Cluster_MI"=w908:T5, "Message from Hardware"=w912:string, "MIParameters.MIRecipeOpcodes.DoorLockStatus.DoorLockStatusResponse"=w913:string[])
        n266 = Index Array(array=w913) -> (element=w911:string)  [unwired: 1 in]
        n267 = Equal?(x=w912, y=w911) -> (x = y?=w909:bool)
        n268 = case shown="False" w909 {
          tunnel: w907 -> [w923 w930]
          tunnel: [w922 w929] -> w906
          tunnel: w905 -> [w921 w926]
          tunnel: w908 -> [w918 w925]
          tunnel: [w917 w924] -> w904
          frame True {
            # "Door Locked"
            n269 = call "Output_MI.vi"("Machine Interface Actor in"=w921, "Output Cluster_MI"=w918, "State"="DiagnosticsResult", "Sub State"="DoorLocked", "error in (no error)"=w923) -> ("Machine Interface Actor out"=w917:refnum<class "Machine Interface.lvclass">, "error out"=w922:errorcluster)  [unwired: 9 in]
          }
          frame False {
            # "Door Unlock"
            n270 = call "Output_MI.vi"("Machine Interface Actor in"=w926, "Output Cluster_MI"=w925, "State"="DiagnosticsResult", "Sub State"="DoorUnlocked", "error in (no error)"=w930) -> ("Machine Interface Actor out"=w924:refnum<class "Machine Interface.lvclass">, "error out"=w929:errorcluster)  [unwired: 9 in]
          }
        }
        n271 = call <vilib>:"Add State(s) to Queue__JKI_lib_State_Machine.vi"("State(s) in (\"\")"=w916) -> ("States Out"=w915:string)  [unwired: 14 in]
      }
      frame "---------- Limit Switch Status Check State----------" {
        # "Do not put any code in this frame.\n(It is a separator )"
        n272 = call <vilib>:"Add State(s) to Queue__JKI_lib_State_Machine.vi"("State(s) in (\"\")"=w936) -> ("States Out"=w935:string)  [unwired: 14 in]
      }
      frame "LimitSwitchStatusCheck" {
        n273 = Unbundle By Name(w940) -> ("MIParameters"=w945:T4)
        n274 = Concatenate Strings("LimitSwitchStatusCheck >>" ("string"), w944) -> (w943:string)
        n275 = call "State wise behavior_MI.vi"("error in (no error)"=w947, "State"=w943, "MIRecipeOpcodes"=w945, "VISA Refnum in"=w938) -> ("error out"=w946:errorcluster, "VISA Refnum out"=w937:refnum<visa-resource-name>)  [unwired: 6 in]
        n276 = Bundle By Name(cluster=w940, "Timeout"=2000) -> (w939:T3)
        n277 = Concatenate Strings("Wait >> PinStatusCheck" ("State(s) in Front (\"\")"), w944) -> (w949:string)
        n278 = call <vilib>:"Add State(s) to Queue__JKI_lib_State_Machine.vi"("State(s) in Front (\"\")"=w949, "State(s) in (\"\")"=w952) -> ("States Out"=w951:string)  [unwired: 13 in]
      }
      frame "LimitSwitchStatusResponse" {
        n279 = case shown="\"Rack1\", Default" w955 {
          tunnel: [w966 w974] -> w956
          tunnel: w953 -> [w965 w973]
          frame "Rack1", Default {
            # "Rack 1 Open Limit switch status response"
            n280 = Unbundle By Name(w965) -> ("Message from Hardware"=w963:string, "Rack1 Response.LimitSwitchStatusResponse"=w964:string[])
            n281 = Index Array(array=w964) -> (element=w962:string)  [unwired: 1 in]
            n282 = Equal?(x=w963, y=w962) -> (x = y?=w961:bool)
            n283 = case shown="False" w961 {
              tunnel: ["GuideOpen >> Rack1" "GuideOpenResponse >> Rack1"] -> w966
              frame True {
                # "Guides are not in Home position"
              }
              frame False {
                # "Guides are in Home position"
              }
            }
          }
          frame "Rack2" {
            # "Rack 2 Open Limit switch status response"
            n284 = Unbundle By Name(w973) -> ("Message from Hardware"=w971:string, "Rack2 Response.LimitSwitchStatusResponse"=w972:string[])
            n285 = Index Array(array=w972) -> (element=w970:string)  [unwired: 1 in]
            n286 = Equal?(x=w971, y=w970) -> (x = y?=w969:bool)
            n287 = case shown="True" w969 {
              tunnel: ["GuideOpen >> Rack2" "GuideOpenResponse >> Rack2"] -> w974
              frame True {
                # "Guides are not in Home position"
              }
              frame False {
                # "Guides are in Home position"
              }
            }
          }
        }
        n288 = call <vilib>:"Add State(s) to Queue__JKI_lib_State_Machine.vi"("State(s) in Front (\"\")"=w956, "State(s) in (\"\")"=w960) -> ("States Out"=w959:string)  [unwired: 13 in]
      }
      frame "---------- Motor Diagnostics State ----------" {
        # "Do not put any code in this frame.\n(It is a separator )"
        n289 = call <vilib>:"Add State(s) to Queue__JKI_lib_State_Machine.vi"("State(s) in (\"\")"=w982) -> ("States Out"=w981:string)  [unwired: 14 in]
      }
      frame "MotorDiagnostics" {
        n290 = Unbundle By Name(w993) -> ("Output Cluster_MI"=w987:T5, "Number of Racks"=w985:i32, "MIParameters"=w986:T4)
        n291 = case shown="\"Rack2 Diagnostics Done\"" w988 {
          tunnel: [w1006 "Wait" ("State(s) in Front (\"\")") "LimitSwitchStatusCheck >> Rack1 " ("State(s) in Front (\"\")")] -> w996
          tunnel: w985 -> [w1005 _ _]
          tunnel: w992 -> [w1002 w1023 w1032]
          tunnel: [w1001 w1022 w1031] -> w991
          tunnel: [w1004 w1025 w1028] -> w990
          tunnel: w989 -> [w1004 w1025 w1029]
          tunnel: w984 -> [w1003 w1024 w1027]
          tunnel: w987 -> [w1000 w1021 _]
          tunnel: w986 -> [_ _ w1030]
          tunnel: [w999 w1018 w1027] -> w983
          frame "Rack1 Diagnostics Done" {
            n292 = case shown="1, Default" w1005 {
              tunnel: ["Wait" ("State(s) in Front (\"\")") "LimitSwitchStatusCheck >> Rack2 " ("State(s) in Front (\"\")")] -> w1006
              tunnel: w1003 -> [w1013 w1015]
              tunnel: w1002 -> [w1012 w1016]
              tunnel: [w1011 w1016] -> w1001
              tunnel: w1000 -> [w1008 _]
              tunnel: [w1007 w1015] -> w999
              frame 1, Default {
                n293 = call "Output_MI.vi"("Machine Interface Actor in"=w1013, "Output Cluster_MI"=w1008, "State"="DiagnosticsResult", "Sub State"="MotorDiagnosticsDone", "error in (no error)"=w1012) -> ("Machine Interface Actor out"=w1007:refnum<class "Machine Interface.lvclass">, "error out"=w1011:errorcluster)  [unwired: 9 in]
              }
              frame 2 {
              }
            }
          }
          frame "Rack2 Diagnostics Done" {
            n294 = call "Output_MI.vi"("Machine Interface Actor in"=w1024, "Output Cluster_MI"=w1021, "State"="DiagnosticsResult", "Sub State"="MotorDiagnosticsDone", "error in (no error)"=w1023) -> ("Machine Interface Actor out"=w1018:refnum<class "Machine Interface.lvclass">, "error out"=w1022:errorcluster)  [unwired: 9 in]
          }
          frame "", Default {
            n295 = call "State wise behavior_MI.vi"("error in (no error)"=w1032, "State"="DHBLS", "MIRecipeOpcodes"=w1030, "VISA Refnum in"=w1029) -> ("error out"=w1031:errorcluster, "VISA Refnum out"=w1028:refnum<visa-resource-name>)  [unwired: 6 in]
          }
        }
        n296 = Bundle By Name(cluster=w993, "State"="MotorDiagnostics") -> (w995:T3)
        n297 = call <vilib>:"Add State(s) to Queue__JKI_lib_State_Machine.vi"("State(s) in Front (\"\")"=w996, "State(s) in (\"\")"=w998) -> ("States Out"=w997:string)  [unwired: 13 in]
      }
      frame "GuideOpen" {
        n298 = Unbundle By Name(w1041) -> ("State"=w1042:string, "Output Cluster_MI"=w1049:T5, "MIParameters"=w1048:T4)
        n299 = Concatenate Strings("GuideOpen >> " ("string"), w1046) -> (w1047:string)
        n300 = call "State wise behavior_MI.vi"("error in (no error)"=w1044, "State"=w1047, "MIRecipeOpcodes"=w1048, "VISA Refnum in"=w1038) -> ("error out"=w1043:errorcluster, "VISA Refnum out"=w1037:refnum<visa-resource-name>)  [unwired: 6 in]
        n301 = case shown="\"MotorDiagnostics\"" w1042 {
          tunnel: w1043 -> [w1056 w1066 w1079 w1083]
          tunnel: [w1056 w1067 w1080 w1083] -> w1051
          tunnel: ["Wait" ("State(s) in Front (\"\")") "Wait >> MotorDiagnostics_GuideOpen" ("State(s) in Front (\"\")") "Wait >> Stop_GuideOpen" ("State(s) in Front (\"\")") "Wait >> SoftwareExit_GuideOpen" ("State(s) in Front (\"\")")] -> w1050
          tunnel: w1036 -> [w1054 w1059 w1072 w1081]
          tunnel: w1049 -> [_ w1064 w1077 _]
          tunnel: [w1054 w1057 w1070 w1081] -> w1035
          frame Default {
          }
          frame "MotorDiagnostics" {
            n302 = call "Output_MI.vi"("Machine Interface Actor in"=w1059, "Output Cluster_MI"=w1064, "State"="LoadingBar", "Sub State"="GuideOpen", "error in (no error)"=w1066) -> ("Machine Interface Actor out"=w1058:refnum<class "Machine Interface.lvclass">, "error out"=w1065:errorcluster)  [unwired: 9 in]
            n303 = call "Output_MI.vi"("Machine Interface Actor in"=w1058, "Output Cluster_MI"=w1064, "State"="ButtonPress", "Sub State"="DisableUIButtons" ("Disable UI Buttons"), "error in (no error)"=w1065) -> ("Machine Interface Actor out"=w1057:refnum<class "Machine Interface.lvclass">, "error out"=w1067:errorcluster)  [unwired: 9 in]
          }
          frame "Stop" {
            n304 = call "Output_MI.vi"("Machine Interface Actor in"=w1072, "Output Cluster_MI"=w1077, "State"="LoadingBar", "Sub State"="GuideOpen", "error in (no error)"=w1079) -> ("Machine Interface Actor out"=w1071:refnum<class "Machine Interface.lvclass">, "error out"=w1078:errorcluster)  [unwired: 9 in]
            n305 = call "Output_MI.vi"("Machine Interface Actor in"=w1071, "Output Cluster_MI"=w1077, "State"="ButtonPress", "Sub State"="DisableUIButtons" ("Disable UI Buttons"), "error in (no error)"=w1078) -> ("Machine Interface Actor out"=w1070:refnum<class "Machine Interface.lvclass">, "error out"=w1080:errorcluster)  [unwired: 9 in]
          }
          frame "SoftwareExit" {
          }
        }
        n306 = Bundle By Name(cluster=w1041, "Timeout"=50000) -> (w1040:T3)
        n307 = call <vilib>:"Add State(s) to Queue__JKI_lib_State_Machine.vi"("State(s) in Front (\"\")"=w1050, "State(s) in (\"\")"=w1052) -> ("States Out"=w1053:string)  [unwired: 13 in]
      }
      frame "GuideOpenResponse" {
        n308 = Unbundle By Name(w1088) -> ("Number of Racks"=w1086:i32, "Output Cluster_MI"=w1087:T5, "Message from Hardware"=w1089:string, "First Call?"=w1090:bool, "State"=w1094:string)
        n309 = case shown="\"MasterSample\", \"Stop\"" w1094 {
          tunnel: [w1113 w1186 w1246 w1302] -> w1097
          tunnel: w1093 -> [w1109 w1190 w1245 w1301]
          tunnel: [w1112 TRUE ("First Call?") TRUE ("First Call?") TRUE ("First Call?")] -> w1096
          tunnel: w1092 -> [w1111 w1188 w1243 w1296]
          tunnel: [w1110 w1187 w1242 w1295] -> w1091
          tunnel: w1090 -> [w1108 _ _ _]
          tunnel: w1089 -> [w1107 w1183 w1239 w1298]
          tunnel: w1085 -> [w1103 w1189 w1244 w1294]
          tunnel: w1087 -> [w1102 w1181 w1237 w1293]
          tunnel: w1086 -> [_ w1180 w1236 w1292]
          tunnel: [w1101 w1179 w1235 w1291] -> w1084
          frame "MotorDiagnostics", Default {
            n310 = String Subset(string=w1107, offset (0)=2, length (rest)=1 ("length (rest)")) -> (substring=w1104:string)
            n311 = case shown="\"P\", Default" w1104 {
              tunnel: ["" w1131] -> w1113
              tunnel: [w1122 w1130] -> w1112
              tunnel: w1111 -> [w1120 w1129]
              tunnel: [w1119 w1128] -> w1110
              tunnel: w1109 -> [_ w1127]
              tunnel: w1108 -> [w1122 w1126]
              tunnel: w1103 -> [w1118 w1125]
              tunnel: w1102 -> [w1117 w1124]
              tunnel: [w1114 w1123] -> w1101
              frame "W" {
                n312 = call "Output_MI.vi"("Machine Interface Actor in"=w1118, "Output Cluster_MI"=w1117, "State"="DiagnosticsResult", "Sub State"="GuideOpenFail", "error in (no error)"=w1120) -> ("Machine Interface Actor out"=w1114:refnum<class "Machine Interface.lvclass">, "error out"=w1119:errorcluster)  [unwired: 9 in]
              }
              frame "P", Default {
                n313 = case shown="\"Rack1\"" w1127 {
                  tunnel: ["" w1143 w1165] -> w1131
                  tunnel: w1126 -> [w1134 w1142 w1164]
                  tunnel: [w1134 w1141 w1163] -> w1130
                  tunnel: w1129 -> [w1133 w1140 w1162]
                  tunnel: [w1133 w1139 w1161] -> w1128
                  tunnel: w1125 -> [w1132 w1138 w1160]
                  tunnel: w1124 -> [_ w1137 w1159]
                  tunnel: [w1132 w1136 w1158] -> w1123
                  frame Default {
                  }
                  frame "Rack1" {
                    n314 = case shown="False" w1142 {
                      selector: w1142 -> [_ w1156]
                      tunnel: ["MotorDiagnostics >> Rack1 Diagnostics Done" "GuideClose >> Rack1 "] -> w1143
                      tunnel: [TRUE w1155] -> w1141
                      tunnel: w1140 -> [w1145 w1153]
                      tunnel: [w1145 w1154] -> w1139
                      tunnel: w1138 -> [w1144 w1152]
                      tunnel: w1137 -> [_ w1151]
                      tunnel: [w1144 w1148] -> w1136
                      frame False {
                        # "Home Reached\nMotor Diagnostics for Rack 1 Done"
                      }
                      frame True {
                        n315 = Not(x=w1156) -> (.not. x?=w1155:bool)
                        n316 = call "Output_MI.vi"("Machine Interface Actor in"=w1152, "Output Cluster_MI"=w1151, "State"="LoadingBar", "Sub State"="HomeReached", "error in (no error)"=w1153) -> ("Machine Interface Actor out"=w1148:refnum<class "Machine Interface.lvclass">, "error out"=w1154:errorcluster)  [unwired: 9 in]
                      }
                    }
                  }
                  frame "Rack2" {
                    n317 = case shown="False" w1164 {
                      selector: w1164 -> [_ w1177]
                      tunnel: ["MotorDiagnostics >> Rack2 Diagnostics Done" "GuideClose >> Rack2 "] -> w1165
                      tunnel: [TRUE w1176] -> w1163
                      tunnel: w1162 -> [w1167 w1175]
                      tunnel: [w1167 w1174] -> w1161
                      tunnel: w1160 -> [w1166 w1173]
                      tunnel: w1159 -> [_ w1172]
                      tunnel: [w1166 w1170] -> w1158
                      frame False {
                        # "Home Reached\nMotor Diagnostics for Rack 2 Done"
                      }
                      frame True {
                        # "Home Reached Message is sent to UI"
                        n318 = Not(x=w1177) -> (.not. x?=w1176:bool)
                        n319 = call "Output_MI.vi"("Machine Interface Actor in"=w1173, "Output Cluster_MI"=w1172, "State"="HomeReached", "error in (no error)"=w1175) -> ("Machine Interface Actor out"=w1170:refnum<class "Machine Interface.lvclass">, "error out"=w1174:errorcluster)  [unwired: 10 in]
                      }
                    }
                  }
                }
              }
            }
          }
          frame "MasterSample", "Stop" {
            n320 = String Subset(string=w1183, offset (0)=2, length (rest)=1 ("length (rest)")) -> (substring=w1182:string)
            n321 = case shown="\"P\", Default" w1182 {
              tunnel: w1190 -> [_ w1208]
              tunnel: w1189 -> [w1196 w1207]
              tunnel: w1188 -> [w1194 w1206]
              tunnel: [w1193 w1205] -> w1187
              tunnel: ["" ("State(s) in Front (\"\")") w1204] -> w1186
              tunnel: w1181 -> [w1197 w1203]
              tunnel: w1180 -> [_ w1202]
              tunnel: [w1192 w1201] -> w1179
              frame "W" {
                n322 = Bundle By Name(cluster=w1197, "Error Message"="Motor_0x03000201") -> (w1199:T5)
                n323 = call "Output_MI.vi"("Machine Interface Actor in"=w1196, "Output Cluster_MI"=w1199, "State"="ErrorMessage", "error in (no error)"=w1194) -> ("Machine Interface Actor out"=w1192:refnum<class "Machine Interface.lvclass">, "error out"=w1193:errorcluster)  [unwired: 10 in]
              }
              frame "P", Default {
                n324 = case shown="\"Rack1\", Default" w1208 {
                  tunnel: w1202 -> [_ w1223]
                  tunnel: ["Wait" ("State(s) in Front (\"\")") w1222] -> w1204
                  tunnel: w1207 -> [w1213 w1221]
                  tunnel: w1206 -> [w1215 w1220]
                  tunnel: [w1214 w1219] -> w1205
                  tunnel: w1203 -> [w1212 w1218]
                  tunnel: [w1209 w1217] -> w1201
                  frame "Rack2" {
                    n325 = call "Output_MI.vi"("Machine Interface Actor in"=w1213, "Output Cluster_MI"=w1212, "State"="MessageToSM", "Sub State"="HomeReached", "error in (no error)"=w1215) -> ("Machine Interface Actor out"=w1209:refnum<class "Machine Interface.lvclass">, "error out"=w1214:errorcluster)  [unwired: 9 in]
                  }
                  frame "Rack1", Default {
                    n326 = case shown="1, Default" w1223 {
                      tunnel: ["Wait" "LimitSwitchStatusCheck >> Rack2" ("State(s) in Front (\"\")")] -> w1222
                      tunnel: w1221 -> [w1228 w1232]
                      tunnel: w1220 -> [w1230 w1233]
                      tunnel: [w1229 w1233] -> w1219
                      tunnel: w1218 -> [w1227 _]
                      tunnel: [w1224 w1232] -> w1217
                      frame 1, Default {
                        n327 = call "Output_MI.vi"("Machine Interface Actor in"=w1228, "Output Cluster_MI"=w1227, "State"="MessageToSM", "Sub State"="HomeReached", "error in (no error)"=w1230) -> ("Machine Interface Actor out"=w1224:refnum<class "Machine Interface.lvclass">, "error out"=w1229:errorcluster)  [unwired: 9 in]
                      }
                      frame 2 {
                      }
                    }
                  }
                }
              }
            }
          }
          frame "SoftwareExit" {
            n328 = String Subset(string=w1239, offset (0)=2, length (rest)=1 ("length (rest)")) -> (substring=w1238:string)
            n329 = case shown="\"P\", Default" w1238 {
              tunnel: ["" ("State(s) in Front (\"\")") w1264] -> w1246
              tunnel: w1245 -> [_ w1263]
              tunnel: w1244 -> [w1252 w1262]
              tunnel: w1243 -> [w1250 w1261]
              tunnel: [w1249 w1260] -> w1242
              tunnel: w1237 -> [w1251 w1259]
              tunnel: w1236 -> [_ w1258]
              tunnel: [w1248 w1257] -> w1235
              frame "W" {
                n330 = Bundle By Name(cluster=w1251, "Error Message"="Motor_0x03000202") -> (w1255:T5)
                n331 = call "Output_MI.vi"("Machine Interface Actor in"=w1252, "Output Cluster_MI"=w1255, "State"="ErrorMessage", "error in (no error)"=w1250) -> ("Machine Interface Actor out"=w1248:refnum<class "Machine Interface.lvclass">, "error out"=w1249:errorcluster)  [unwired: 10 in]
              }
              frame "P", Default {
                n332 = case shown="\"Rack1\", Default" w1263 {
                  tunnel: ["Shutdown" ("State(s) in Front (\"\")") w1279] -> w1264
                  tunnel: w1262 -> [w1271 w1278]
                  tunnel: w1261 -> [w1270 w1277]
                  tunnel: [w1269 w1276] -> w1260
                  tunnel: w1259 -> [w1268 w1275]
                  tunnel: w1258 -> [_ w1274]
                  tunnel: [w1265 w1273] -> w1257
                  frame "Rack2" {
                    n333 = call "Output_MI.vi"("Machine Interface Actor in"=w1271, "Output Cluster_MI"=w1268, "State"="MessageToSM", "Sub State"="HomeReached", "error in (no error)"=w1270) -> ("Machine Interface Actor out"=w1265:refnum<class "Machine Interface.lvclass">, "error out"=w1269:errorcluster)  [unwired: 9 in]
                  }
                  frame "Rack1", Default {
                    n334 = case shown="1, Default" w1274 {
                      tunnel: ["Shutdown" "LimitSwitchStatusCheck >> Rack2" ("State(s) in Front (\"\")")] -> w1279
                      tunnel: w1278 -> [w1284 w1288]
                      tunnel: w1277 -> [w1286 w1289]
                      tunnel: [w1285 w1289] -> w1276
                      tunnel: w1275 -> [w1283 _]
                      tunnel: [w1280 w1288] -> w1273
                      frame 1, Default {
                        n335 = call "Output_MI.vi"("Machine Interface Actor in"=w1284, "Output Cluster_MI"=w1283, "State"="MessageToSM", "Sub State"="HomeReached", "error in (no error)"=w1286) -> ("Machine Interface Actor out"=w1280:refnum<class "Machine Interface.lvclass">, "error out"=w1285:errorcluster)  [unwired: 9 in]
                      }
                      frame 2 {
                      }
                    }
                  }
                }
              }
            }
          }
          frame "Select" {
            n336 = String Subset(string=w1298, offset (0)=2, length (rest)=1 ("length (rest)")) -> (substring=w1297:string)
            n337 = case shown="\"W\"" w1297 {
              tunnel: ["" ("State(s) in Front (\"\")") w1318] -> w1302
              tunnel: w1301 -> [_ w1317]
              tunnel: w1296 -> [w1310 w1316]
              tunnel: [w1309 w1316] -> w1295
              tunnel: w1294 -> [w1308 w1313]
              tunnel: w1293 -> [w1307 _]
              tunnel: w1292 -> [_ w1315]
              tunnel: [w1304 w1314] -> w1291
              frame "W" {
                n338 = Bundle By Name(cluster=w1307, "Error Message"="Motor_0x03000203") -> (w1306:T5)
                n339 = call "Output_MI.vi"("Machine Interface Actor in"=w1308, "Output Cluster_MI"=w1306, "State"="ErrorMessage", "error in (no error)"=w1310) -> ("Machine Interface Actor out"=w1304:refnum<class "Machine Interface.lvclass">, "error out"=w1309:errorcluster)  [unwired: 10 in]
              }
              frame "P", Default {
                n340 = case shown="\"Rack2\"" w1317 {
                  tunnel: w1315 -> [_ w1323]
                  tunnel: ["MoveMotorReadyToInsert >> Rack2" ("State(s) in Front (\"\")") w1322] -> w1318
                  tunnel: [w1319 w1321] -> w1314
                  tunnel: w1313 -> [w1319 w1321]
                  frame "Rack2" {
                  }
                  frame "Rack1", Default {
                    n341 = case shown="2" w1323 {
                      tunnel: ["MoveMotorReadyToInsert >> Rack1" ("State(s) in Front (\"\")") "LimitSwitchStatusCheck >> Rack2" ("State(s) in Front (\"\")")] -> w1322
                      frame 1, Default {
                      }
                      frame 2 {
                      }
                    }
                  }
                }
              }
            }
          }
        }
        n342 = Bundle By Name(cluster=w1088, "First Call?"=w1096) -> (w1095:T3)
        n343 = call <vilib>:"Add State(s) to Queue__JKI_lib_State_Machine.vi"("State(s) in Front (\"\")"=w1097, "State(s) in (\"\")"=w1100) -> ("States Out"=w1099:string)  [unwired: 13 in]
      }
      frame "GuideClose" {
        n344 = Unbundle By Name(w1331) -> ("State"=w1333:string, "MIParameters"=w1339:T4, "Output Cluster_MI"=w1340:T5)
        n345 = Concatenate Strings("GuideClose >> " ("string"), w1338) -> (w1336:string)
        n346 = call "State wise behavior_MI.vi"("error in (no error)"=w1335, "State"=w1336, "MIRecipeOpcodes"=w1339, "VISA Refnum in"=w1329) -> ("error out"=w1334:errorcluster, "VISA Refnum out"=w1328:refnum<visa-resource-name>)  [unwired: 6 in]
        n347 = case shown="\"MotorDiagnostics\"" w1333 {
          tunnel: w1334 -> [w1346 w1356]
          tunnel: [w1346 w1357] -> w1342
          tunnel: w1327 -> [w1345 w1349]
          tunnel: w1340 -> [_ w1354]
          tunnel: [w1345 w1347] -> w1326
          frame Default {
          }
          frame "MotorDiagnostics" {
            n348 = call "Output_MI.vi"("Machine Interface Actor in"=w1349, "Output Cluster_MI"=w1354, "State"="LoadingBar", "Sub State"="GuideClose" ("State"), "error in (no error)"=w1356) -> ("Machine Interface Actor out"=w1348:refnum<class "Machine Interface.lvclass">, "error out"=w1355:errorcluster)  [unwired: 9 in]
            n349 = call "Output_MI.vi"("Machine Interface Actor in"=w1348, "Output Cluster_MI"=w1354, "State"="ButtonPress", "Sub State"="DisableUIButtons" ("Disable UI Buttons"), "error in (no error)"=w1355) -> ("Machine Interface Actor out"=w1347:refnum<class "Machine Interface.lvclass">, "error out"=w1357:errorcluster)  [unwired: 9 in]
          }
        }
        n350 = Bundle By Name(cluster=w1331, "Timeout"=50000) -> (w1330:T3)
        n351 = call <vilib>:"Add State(s) to Queue__JKI_lib_State_Machine.vi"("State(s) in Front (\"\")"="Wait >> MotorDiagnostics_GuideClose" ("State(s) in Front (\"\")"), "State(s) in (\"\")"=w1344) -> ("States Out"=w1343:string)  [unwired: 13 in]
      }
      frame "GuideCloseResponse" {
        n352 = Unbundle By Name(w1365) -> ("Message from Hardware"=w1362:string, "Output Cluster_MI"=w1360:T5)
        n353 = String Subset(string=w1362, offset (0)=2, length (rest)=1 ("length (rest)")) -> (substring=w1361:string)
        n354 = case shown="\"P\", Default" w1361 {
          tunnel: w1369 -> [_ w1387]
          tunnel: ["" w1386] -> w1368
          tunnel: w1367 -> [w1378 w1385]
          tunnel: [w1377 w1384] -> w1366
          tunnel: w1359 -> [w1379 w1383]
          tunnel: w1360 -> [w1376 w1382]
          tunnel: [w1373 w1381] -> w1358
          frame "W" {
            n355 = call "Output_MI.vi"("Machine Interface Actor in"=w1379, "Output Cluster_MI"=w1376, "State"="DiagnosticsResult", "Sub State"="GuideCloseFail", "error in (no error)"=w1378) -> ("Machine Interface Actor out"=w1373:refnum<class "Machine Interface.lvclass">, "error out"=w1377:errorcluster)  [unwired: 9 in]
          }
          frame "P", Default {
            n356 = case shown="\"Rack2\"" w1387 {
              tunnel: ["GuideOpen >> Rack1" "GuideOpen >> Rack2"] -> w1386
              tunnel: w1385 -> [w1397 w1408]
              tunnel: [w1398 w1409] -> w1384
              tunnel: w1383 -> [w1390 w1401]
              tunnel: w1382 -> [w1395 w1407]
              tunnel: [w1388 w1402] -> w1381
              frame "Rack1", Default {
                n357 = call "Output_MI.vi"("Machine Interface Actor in"=w1390, "Output Cluster_MI"=w1395, "State"="LoadingBar", "Sub State"="GuidesClosed" ("State"), "error in (no error)"=w1397) -> ("Machine Interface Actor out"=w1389:refnum<class "Machine Interface.lvclass">, "error out"=w1396:errorcluster)  [unwired: 9 in]
                n358 = call "Output_MI.vi"("Machine Interface Actor in"=w1389, "Output Cluster_MI"=w1395, "State"="ButtonPress", "Sub State"="DisableUIButtons" ("Disable UI Buttons"), "error in (no error)"=w1396) -> ("Machine Interface Actor out"=w1388:refnum<class "Machine Interface.lvclass">, "error out"=w1398:errorcluster)  [unwired: 9 in]
              }
              frame "Rack2" {
                n359 = call "Output_MI.vi"("Machine Interface Actor in"=w1401, "Output Cluster_MI"=w1407, "State"="LoadingBar", "Sub State"="GuidesClosed", "error in (no error)"=w1408) -> ("Machine Interface Actor out"=w1400:refnum<class "Machine Interface.lvclass">, "error out"=w1410:errorcluster)  [unwired: 9 in]
                n360 = call "Output_MI.vi"("Machine Interface Actor in"=w1400, "Output Cluster_MI"=w1407, "State"="ButtonPress", "Sub State"="DisableUIButtons" ("Disable UI Buttons"), "error in (no error)"=w1410) -> ("Machine Interface Actor out"=w1402:refnum<class "Machine Interface.lvclass">, "error out"=w1409:errorcluster)  [unwired: 9 in]
              }
            }
          }
        }
        n361 = call <vilib>:"Add State(s) to Queue__JKI_lib_State_Machine.vi"("State(s) in Front (\"\")"=w1368, "State(s) in (\"\")"=w1372) -> ("States Out"=w1371:string)  [unwired: 13 in]
      }
      frame "RotateReelerMotor" {
        n362 = Unbundle By Name(w1425) -> ("MIParameters"=w1415:T4)
        n363 = call "State wise behavior_MI.vi"("error in (no error)"=w1422, "State"="DHBLS", "MIRecipeOpcodes"=w1415, "VISA Refnum in"=w1413) -> ("error out"=w1417:errorcluster, "VISA Refnum out"=w1412:refnum<visa-resource-name>)  [unwired: 6 in]
        n364 = Concatenate Strings("RotateReelerMotor >> " ("string"), w1420) -> (w1418:string)
        n365 = call "State wise behavior_MI.vi"("error in (no error)"=w1417, "State"=w1418, "MIRecipeOpcodes"=w1415, "VISA Refnum in"=w1412) -> ("error out"=w1416:errorcluster, "VISA Refnum out"=w1414:refnum<visa-resource-name>)  [unwired: 6 in]
        n366 = Bundle By Name(cluster=w1425, "State"="MotorDiagnostics") -> (w1424:T3)
        n367 = call <vilib>:"Add State(s) to Queue__JKI_lib_State_Machine.vi"("State(s) in (\"\")"=w1427) -> ("States Out"=w1428:string)  [unwired: 14 in]
      }
      frame "---------- Hardware Button Diagnostics State ----------" {
        # "Do not put any code in this frame.\n(It is a separator )"
        n368 = call <vilib>:"Add State(s) to Queue__JKI_lib_State_Machine.vi"("State(s) in (\"\")"=w1434) -> ("States Out"=w1433:string)  [unwired: 14 in]
      }
      frame "HardwareButtonDiagnostics" {
        n369 = Unbundle By Name(w1444) -> ("MIParameters"=w1441:T4)
        n370 = call "State wise behavior_MI.vi"("error in (no error)"=w1442, "State"="DHBLS", "MIRecipeOpcodes"=w1441, "VISA Refnum in"=w1436) -> ("error out"=w1439:errorcluster, "VISA Refnum out"=w1437:refnum<visa-resource-name>)  [unwired: 6 in]
        n371 = call "State wise behavior_MI.vi"("error in (no error)"=w1439, "State"="HardwareButtonDiagnostics", "MIRecipeOpcodes"=w1441, "VISA Refnum in"=w1437) -> ("error out"=w1438:errorcluster, "VISA Refnum out"=w1435:refnum<visa-resource-name>)  [unwired: 6 in]
        n372 = Bundle By Name(cluster=w1444, "State"="HardwareButtonDiagnostics") -> (w1446:T3)
        n373 = call <vilib>:"Add State(s) to Queue__JKI_lib_State_Machine.vi"("State(s) in (\"\")"=w1449) -> ("States Out"=w1448:string)  [unwired: 14 in]
      }
      frame "---------- Tower Lamp Diagnostics ----------" {
        # "Do not put any code in this frame.\n(It is a separator )"
        n374 = call <vilib>:"Add State(s) to Queue__JKI_lib_State_Machine.vi"("State(s) in (\"\")"=w1455) -> ("States Out"=w1454:string)  [unwired: 14 in]
      }
      frame "TowerLampDiagnostics" {
        n375 = Unbundle By Name(w1465) -> ("MIParameters"=w1461:T4)
        n376 = call "State wise behavior_MI.vi"("error in (no error)"=w1463, "State"="DHBLS", "MIRecipeOpcodes"=w1461, "VISA Refnum in"=w1458) -> ("error out"=w1462:errorcluster, "VISA Refnum out"=w1456:refnum<visa-resource-name>)  [unwired: 6 in]
        n377 = call "State wise behavior_MI.vi"("error in (no error)"=w1462, "State"="TowerLampDiagnostics", "MIRecipeOpcodes"=w1461, "VISA Refnum in"=w1456) -> ("error out"=w1464:errorcluster, "VISA Refnum out"=w1457:refnum<visa-resource-name>)  [unwired: 6 in]
        n378 = call <vilib>:"Add State(s) to Queue__JKI_lib_State_Machine.vi"("State(s) in (\"\")"=w1468) -> ("States Out"=w1467:string)  [unwired: 14 in]
      }
      frame "---------- Camera Optics Diagnostics State ----------" {
        # "Do not put any code in this frame.\n(It is a separator )"
        n379 = call <vilib>:"Add State(s) to Queue__JKI_lib_State_Machine.vi"("State(s) in (\"\")"=w1474) -> ("States Out"=w1473:string)  [unwired: 14 in]
      }
      frame "CameraOpticsDiagnostics" {
        n380 = Unbundle By Name(w1479) -> ("MIParameters"=w1478:T4)
        n381 = call "State wise behavior_MI.vi"("error in (no error)"=w1481, "State"="DHBLS", "MIRecipeOpcodes"=w1478, "VISA Refnum in"=w1476) -> ("error out"=w1480:errorcluster, "VISA Refnum out"=w1475:refnum<visa-resource-name>)  [unwired: 6 in]
        n382 = call <vilib>:"Add State(s) to Queue__JKI_lib_State_Machine.vi"("State(s) in Front (\"\")"="Wait" ("State(s) in Front (\"\")"), "State(s) in (\"\")"=w1485) -> ("States Out"=w1484:string)  [unwired: 13 in]
      }
      frame "---------- Select State ----------" {
        # "Do not put any code in this frame.\n(It is a separator )"
        n383 = call <vilib>:"Add State(s) to Queue__JKI_lib_State_Machine.vi"("State(s) in (\"\")"=w1491) -> ("States Out"=w1490:string)  [unwired: 14 in]
      }
      frame "Select" {
        n384 = Unbundle By Name(w1499) -> ("MIParameters"=w1494:T4)
        n385 = call "State wise behavior_MI.vi"("error in (no error)"=w1496, "State"="DHBLS", "MIRecipeOpcodes"=w1494, "VISA Refnum in"=w1493) -> ("error out"=w1495:errorcluster, "VISA Refnum out"=w1492:refnum<visa-resource-name>)  [unwired: 6 in]
        n386 = call <vilib>:"Add State(s) to Queue__JKI_lib_State_Machine.vi"("State(s) in (\"\")"=w1501) -> ("States Out"=w1500:string)  [unwired: 14 in]
      }
      frame "PartSelected" {
        # "Part dependent \nopcodes are read"
        n387 = Unbundle By Name(w1503) -> ("MIParameters.MIRecipeOpcodes.PartsList"=w1502:T13)
        n388 = call "Read Part Specfic Parameters.vi"("error in (no error)"=w1507, "Part name"=w1505, "PartsList"=w1502) -> ("error out"=w1506:errorcluster, "PartSpecificParameters"=w1504:T12)  [unwired: 7 in]
        n389 = Bundle By Name(cluster=w1503, "Part details"=w1504, "State"="Select") -> (w1510:T3)
        n390 = call <vilib>:"Add State(s) to Queue__JKI_lib_State_Machine.vi"("State(s) in (\"\")"=w1513) -> ("States Out"=w1512:string)  [unwired: 14 in]
      }
      frame "StartMotorReadyToInsert" {
        n391 = Bundle By Name(cluster=w1519, "State"="Select") -> (w1518:T3)
        n392 = call <vilib>:"Add State(s) to Queue__JKI_lib_State_Machine.vi"("State(s) in Front (\"\")"="LimitSwitchStatusCheck >> Rack1 " ("State(s) in Front (\"\")"), "State(s) in (\"\")"=w1522) -> ("States Out"=w1521:string)  [unwired: 13 in]
      }
      frame "MoveMotorReadyToInsert" {
        n393 = Unbundle By Name(w1526) -> ("Part details.RackDependentOpcodes"=w1527:T14, "MI Offline?"=w1523:bool)
        n394 = case shown="\"Rack2\"" w1535 {
          tunnel: w1527 -> [w1540 w1574]
          tunnel: w1532 -> [w1547 w1571]
          tunnel: w1534 -> [w1546 w1570]
          tunnel: [w1545 w1569] -> w1533
          tunnel: [w1544 w1568] -> w1531
          tunnel: ["Wait >> ReadyToInsert" ("State(s) in Front (\"\")") "Wait" ("State(s) in Front (\"\")")] -> w1530
          tunnel: [w1539 "ReadyToInsert" ("State(s) in Front (\"\")")] -> w1529
          tunnel: w1523 -> [w1538 _]
          frame "Rack1", Default {
            n395 = Index Array(array=w1540, index=0) -> (element=w1548:T15)
            n396 = Unbundle By Name(w1548) -> ("MotorStepsForReadyToInsert"=w1543:string[])
            n397 = for {
              tunnel: w1543 -> [w1556] mode=indexing
              tunnel: w1547 -> [w1557]
              tunnel: w1546 -> [w1555]
              tunnel: [w1554] -> w1545
              tunnel: [w1553] -> w1544
              tunnel: w1538 -> [w1552]
              n398 = case shown="False" w1552 {
                tunnel: w1557 -> [w1562 w1564]
                tunnel: w1556 -> [w1561 _]
                tunnel: w1555 -> [w1560 w1563]
                tunnel: [w1559 w1563] -> w1554
                tunnel: [w1558 w1564] -> w1553
                frame False {
                  n399 = VISA Write(VISA resource name=w1562, write buffer=w1561, error in (no error)=w1560) -> (VISA resource name out=w1558:refnum<visa-resource-name>, error out=w1559:errorcluster)  [unwired: 1 out]
                }
                frame True {
                }
              }
            }
            n400 = Array Size(array=w1540) -> (size(s)=w1541:i32)
            n401 = case shown="1, Default" w1541 {
              tunnel: ["ReadyToInsert" ("State(s) in Front (\"\")") "LimitSwitchStatusCheck >> Rack2"] -> w1539
              frame 1, Default {
                # "Single Rack System"
              }
              frame 2 {
                # "2 Rack System"
              }
            }
          }
          frame "Rack2" {
            n402 = Index Array(array=w1574, index=1) -> (element=w1572:T15)
            n403 = Unbundle By Name(w1572) -> ("MotorStepsForReadyToInsert"=w1567:string[])
            n404 = for {
              tunnel: w1567 -> [w1578] mode=indexing
              tunnel: w1571 -> [w1579]
              tunnel: w1570 -> [w1577]
              tunnel: [w1576] -> w1569
              tunnel: [w1575] -> w1568
              n405 = VISA Write(VISA resource name=w1579, write buffer=w1578, error in (no error)=w1577) -> (VISA resource name out=w1575:refnum<visa-resource-name>, error out=w1576:errorcluster)  [unwired: 1 out]
            }
          }
        }
        n406 = Bundle By Name(cluster=w1526, "Timeout"=20000) -> (w1525:T3)
        n407 = call <vilib>:"Add State(s) to Queue__JKI_lib_State_Machine.vi"("State(s) in Front (\"\")"=w1530, "State(s) in (\"\")"=w1537, "State(s) at Back (\"\")"=w1529) -> ("States Out"=w1536:string)  [unwired: 12 in]
      }
      frame "ReadyToInsert" {
        n408 = Unbundle By Name(w1585) -> ("Output Cluster_MI"=w1584:T5)
        n409 = call "Output_MI.vi"("Machine Interface Actor in"=w1581, "Output Cluster_MI"=w1584, "State"="MessageToSM", "Sub State"="ReadyToInsert", "error in (no error)"=w1586) -> ("Machine Interface Actor out"=w1580:refnum<class "Machine Interface.lvclass">, "error out"=w1587:errorcluster)  [unwired: 9 in]
        n410 = Bundle By Name(cluster=w1585, "State"="Select") -> (w1590:T3)
        n411 = call <vilib>:"Add State(s) to Queue__JKI_lib_State_Machine.vi"("State(s) in Front (\"\")"="Wait" ("State(s) in Front (\"\")"), "State(s) in (\"\")"=w1593) -> ("States Out"=w1592:string)  [unwired: 13 in]
      }
      frame "SetIndex" {
        n412 = Unbundle By Name(w1596) -> ("Part details.RackDependentOpcodes"=w1602:T14, "MI Offline?"=w1594:bool)
        n413 = case shown="\"Rack1\", Default" w1603 {
          tunnel: w1602 -> [w1609 w1640]
          tunnel: w1599 -> [w1614 w1637]
          tunnel: w1601 -> [w1613 w1636]
          tunnel: [w1612 w1635] -> w1600
          tunnel: [w1611 w1634] -> w1598
          tunnel: [w1607 "SelectDone" ("State(s) in Front (\"\")")] -> w1597
          tunnel: w1594 -> [w1606 _]
          frame "Rack1", Default {
            n414 = Index Array(array=w1609, index=0) -> (element=w1615:T15)
            n415 = Unbundle By Name(w1615) -> ("SetIndex"=w1610:string[])
            n416 = for {
              tunnel: w1610 -> [w1623] mode=indexing
              tunnel: w1614 -> [w1624]
              tunnel: w1613 -> [w1622]
              tunnel: [w1621] -> w1612
              tunnel: [w1620] -> w1611
              tunnel: w1606 -> [w1619]
              n417 = case shown="False" w1619 {
                tunnel: w1624 -> [w1629 w1631]
                tunnel: w1623 -> [w1628 _]
                tunnel: w1622 -> [w1627 w1630]
                tunnel: [w1626 w1630] -> w1621
                tunnel: [w1625 w1631] -> w1620
                frame False {
                  n418 = VISA Write(VISA resource name=w1629, write buffer=w1628, error in (no error)=w1627) -> (VISA resource name out=w1625:refnum<visa-resource-name>, error out=w1626:errorcluster)  [unwired: 1 out]
                }
                frame True {
                }
              }
            }
            n419 = Array Size(array=w1609) -> (size(s)=w1608:i32)
            n420 = case shown="1, Default" w1608 {
              tunnel: ["SelectDone" ("State(s) in Front (\"\")") "SetIndex >> Rack2"] -> w1607
              frame 1, Default {
              }
              frame 2 {
              }
            }
          }
          frame "Rack2" {
            n421 = Index Array(array=w1640, index=1) -> (element=w1638:T15)
            n422 = Unbundle By Name(w1638) -> ("SetIndex"=w1633:string[])
            n423 = for {
              tunnel: w1633 -> [w1644] mode=indexing
              tunnel: w1637 -> [w1645]
              tunnel: w1636 -> [w1643]
              tunnel: [w1642] -> w1635
              tunnel: [w1641] -> w1634
              n424 = VISA Write(VISA resource name=w1645, write buffer=w1644, error in (no error)=w1643) -> (VISA resource name out=w1641:refnum<visa-resource-name>, error out=w1642:errorcluster)  [unwired: 1 out]
            }
          }
        }
        n425 = call <vilib>:"Add State(s) to Queue__JKI_lib_State_Machine.vi"("State(s) in Front (\"\")"=w1597, "State(s) in (\"\")"=w1605) -> ("States Out"=w1604:string)  [unwired: 13 in]
      }
      frame "SelectDone" {
        # "Message to SM that Guides are in Ready to Insert Position,\nRun button enabled."
        n426 = Unbundle By Name(w1656) -> ("Output Cluster_MI"=w1652:T5)
        n427 = call "Output_MI.vi"("Machine Interface Actor in"=w1647, "Output Cluster_MI"=w1652, "State"="MessageToSM", "Sub State"="SelectDone", "error in (no error)"=w1648) -> ("Machine Interface Actor out"=w1646:refnum<class "Machine Interface.lvclass">, "error out"=w1653:errorcluster)  [unwired: 9 in]
        n428 = Bundle By Name(cluster=w1656, "State"="Select") -> (w1655:T3)
        n429 = call <vilib>:"Add State(s) to Queue__JKI_lib_State_Machine.vi"("State(s) in (\"\")"=w1658) -> ("States Out"=w1657:string)  [unwired: 14 in]
      }
      frame "SelectionComplete" {
        # "Message to SM that Guides are in Ready to Insert Position,\nRun button enabled."
        n430 = Unbundle By Name(w1668) -> ("MIParameters"=w1663:T4)  [unwired: 1 out]
        n431 = call "State wise behavior_MI.vi"("error in (no error)"=w1664, "State"="SelectDone", "MIRecipeOpcodes"=w1663, "VISA Refnum in"=w1660) -> ("error out"=w1661:errorcluster, "VISA Refnum out"=w1659:refnum<visa-resource-name>)  [unwired: 6 in]
        n432 = Bundle By Name(cluster=w1668, "State"="Select") -> (w1667:T3)
        n433 = call <vilib>:"Add State(s) to Queue__JKI_lib_State_Machine.vi"("State(s) in (\"\")"=w1670) -> ("States Out"=w1669:string)  [unwired: 14 in]
      }
      frame "---------- Run State ----------" {
        # "Do not put any code in this frame.\n(It is a separator )"
        n434 = call <vilib>:"Add State(s) to Queue__JKI_lib_State_Machine.vi"("State(s) in (\"\")"=w1676) -> ("States Out"=w1675:string)  [unwired: 14 in]
      }
      frame "Run" {
        n435 = Unbundle By Name(w1678) -> ("State"=w1680:string)
        n436 = case shown="\"Run\"" w1680 {
          tunnel: ["EnableSensor >> Rack1" ("State(s) in Front (\"\")") "EnableSensor >> Rack1" ("State(s) in Front (\"\")") "MoveMotorReadyToRun >> Rack1" ("State(s) in Front (\"\")")] -> w1681
          frame "Pause" {
          }
          frame "Run" {
          }
          frame "Select", Default {
          }
        }
        n437 = in-place {
          n438 = in-place-cluster #5(w1678) -> ()  [unwired: 2 out]
          n439 = in-place-cluster #5("State"="Run", "Pass after Pause on Fail"=FALSE) -> (w1677:T3)
        }
        n440 = call <vilib>:"Add State(s) to Queue__JKI_lib_State_Machine.vi"("State(s) in Front (\"\")"=w1681, "State(s) in (\"\")"=w1685) -> ("States Out"=w1684:string)  [unwired: 13 in]
      }
      frame "StartMotorReadyToRun" {
        n441 = Bundle By Name(cluster=w1695, "State"="PreRun", "Pass after Pause on Fail"=FALSE) -> (w1694:T3)
        n442 = call <vilib>:"Add State(s) to Queue__JKI_lib_State_Machine.vi"("State(s) in Front (\"\")"="MoveMotorReadyToRun >> Rack1" ("State(s) in Front (\"\")"), "State(s) in (\"\")"=w1700) -> ("States Out"=w1699:string)  [unwired: 13 in]
      }
      frame "HWRunButtonPress" {
        n443 = Unbundle By Name(w1710) -> ("State"=w1709:string, "MIParameters.MIRecipeOpcodes.HardwareButtonDiagnostics.Run"=w1708:string[], "Output Cluster_MI"=w1703:T5)
        n444 = Index Array(array=w1708, index=1) -> (element=w1706:string)
        n445 = case shown="\"HardwareButtonDiagnostics\"" w1709 {
          tunnel: w1712 -> [w1721 w1728]
          tunnel: [w1722 w1731] -> w1711
          tunnel: w1706 -> [_ w1732]
          tunnel: w1705 -> [w1723 w1734]
          tunnel: [w1723 w1733] -> w1704
          tunnel: w1702 -> [w1720 w1725]
          tunnel: w1703 -> [w1719 w1726]
          tunnel: [w1716 w1724] -> w1701
          frame Default {
            n446 = call "Output_MI.vi"("Machine Interface Actor in"=w1720, "Output Cluster_MI"=w1719, "State"="ButtonPress", "Sub State"="Run" ("Button Press"), "error in (no error)"=w1721) -> ("Machine Interface Actor out"=w1716:refnum<class "Machine Interface.lvclass">, "error out"=w1722:errorcluster)  [unwired: 9 in]
          }
          frame "HardwareButtonDiagnostics" {
            n447 = call "Output_MI.vi"("Machine Interface Actor in"=w1725, "Output Cluster_MI"=w1726, "State"="ButtonPress", "Sub State"="Run" ("Button Press"), "error in (no error)"=w1728) -> ("Machine Interface Actor out"=w1724:refnum<class "Machine Interface.lvclass">, "error out"=w1727:errorcluster)  [unwired: 9 in]
            n448 = VISA Write(VISA resource name=w1734, write buffer=w1732, error in (no error)=w1727) -> (VISA resource name out=w1733:refnum<visa-resource-name>, error out=w1731:errorcluster)  [unwired: 1 out]
          }
        }
        n449 = call <vilib>:"Add State(s) to Queue__JKI_lib_State_Machine.vi"("State(s) in Front (\"\")"="Wait" ("State(s) in Front (\"\")"), "State(s) in (\"\")"=w1715) -> ("States Out"=w1714:string)  [unwired: 13 in]
      }
      frame "MoveMotorReadyToRun" {
        n450 = Unbundle By Name(w1738) -> ("Part details.RackDependentOpcodes"=w1739:T14, "MI Offline?"=w1735:bool)
        n451 = case shown="\"Rack2\"" w1747 {
          tunnel: w1739 -> [w1753 w1788]
          tunnel: w1744 -> [w1759 w1785]
          tunnel: w1746 -> [w1758 w1784]
          tunnel: [w1757 w1783] -> w1745
          tunnel: [w1756 w1782] -> w1743
          tunnel: [w1751 "Wait" ("State(s) in Front (\"\")")] -> w1742
          tunnel: [w1752 "RunPositionReached"] -> w1741
          tunnel: w1735 -> [w1750 _]
          frame "Rack1", Default {
            n452 = Index Array(array=w1753, index=0) -> (element=w1760:T15)
            n453 = Unbundle By Name(w1760) -> ("MotorStepsForReadyToRun"=w1755:string[])
            n454 = for {
              tunnel: w1755 -> [w1770] mode=indexing
              tunnel: w1759 -> [w1771]
              tunnel: w1758 -> [w1769]
              tunnel: [w1768] -> w1757
              tunnel: [w1767] -> w1756
              tunnel: w1750 -> [w1766]
              n455 = case shown="True" w1766 {
                tunnel: w1771 -> [w1776 w1778]
                tunnel: w1770 -> [w1775 _]
                tunnel: w1769 -> [w1774 w1777]
                tunnel: [w1773 w1777] -> w1768
                tunnel: [w1772 w1778] -> w1767
                frame False {
                  n456 = VISA Write(VISA resource name=w1776, write buffer=w1775, error in (no error)=w1774) -> (VISA resource name out=w1772:refnum<visa-resource-name>, error out=w1773:errorcluster)  [unwired: 1 out]
                }
                frame True {
                }
              }
            }
            n457 = Array Size(array=w1753) -> (size(s)=w1754:i32)
            n458 = case shown="2" w1754 {
              tunnel: ["RunPositionReached" "MoveMotorReadyToRun >> Rack2"] -> w1752
              tunnel: ["Wait" ("State(s) in Front (\"\")") "Wait" ("State(s) in Front (\"\")")] -> w1751
              frame 1, Default {
              }
              frame 2 {
              }
            }
          }
          frame "Rack2" {
            n459 = Index Array(array=w1788, index=1) -> (element=w1786:T15)
            n460 = Unbundle By Name(w1786) -> ("MotorStepsForReadyToRun"=w1781:string[])
            n461 = for {
              tunnel: w1781 -> [w1792] mode=indexing
              tunnel: w1785 -> [w1793]
              tunnel: w1784 -> [w1791]
              tunnel: [w1790] -> w1783
              tunnel: [w1789] -> w1782
              n462 = VISA Write(VISA resource name=w1793, write buffer=w1792, error in (no error)=w1791) -> (VISA resource name out=w1789:refnum<visa-resource-name>, error out=w1790:errorcluster)  [unwired: 1 out]
            }
          }
        }
        n463 = Bundle By Name(cluster=w1738, "Timeout"=20000) -> (w1737:T3)
        n464 = call <vilib>:"Add State(s) to Queue__JKI_lib_State_Machine.vi"("State(s) in Front (\"\")"=w1742, "State(s) in (\"\")"=w1749, "State(s) at Back (\"\")"=w1741) -> ("States Out"=w1748:string)  [unwired: 12 in]
      }
      frame "RunPositionReached" {
        n465 = Unbundle By Name(w1801) -> ("Output Cluster_MI"=w1798:T5)
        n466 = call "Output_MI.vi"("Machine Interface Actor in"=w1795, "Output Cluster_MI"=w1798, "State"="MessageToSM", "Sub State"="RunPositionReached", "error in (no error)"=w1800) -> ("Machine Interface Actor out"=w1794:refnum<class "Machine Interface.lvclass">, "error out"=w1799:errorcluster)  [unwired: 9 in]
        n467 = call <vilib>:"Add State(s) to Queue__JKI_lib_State_Machine.vi"("State(s) in (\"\")"=w1804) -> ("States Out"=w1803:string)  [unwired: 14 in]
      }
      frame "EnableSensor" {
        n468 = Unbundle By Name(w1807) -> ("Part details.RackDependentOpcodes"=w1815:T14, "MI Offline?"=w1808:bool)
        n469 = case shown="\"Rack1\", Default" w1816 {
          tunnel: w1815 -> [w1822 w1853]
          tunnel: w1812 -> [w1828 w1850]
          tunnel: w1814 -> [w1827 w1849]
          tunnel: [w1820 w1848] -> w1813
          tunnel: [w1826 w1847] -> w1811
          tunnel: [w1821 "PowerOnSensor >> Rack1" ("State(s) in Front (\"\")")] -> w1810
          tunnel: w1808 -> [w1819 _]
          frame "Rack1", Default {
            n470 = Index Array(array=w1822, index=0) -> (element=w1825:T15)
            n471 = Unbundle By Name(w1825) -> ("EnableSensor"=w1824:string[])
            n472 = for {
              tunnel: w1824 -> [w1836] mode=indexing
              tunnel: w1828 -> [w1837]
              tunnel: w1827 -> [w1835]
              tunnel: [w1834] -> w1820
              tunnel: [w1833] -> w1826
              tunnel: w1819 -> [w1832]
              n473 = case shown="True" w1832 {
                tunnel: w1837 -> [w1842 w1844]
                tunnel: w1836 -> [w1841 _]
                tunnel: w1835 -> [w1840 w1843]
                tunnel: [w1839 w1843] -> w1834
                tunnel: [w1838 w1844] -> w1833
                frame False {
                  n474 = VISA Write(VISA resource name=w1842, write buffer=w1841, error in (no error)=w1840) -> (VISA resource name out=w1838:refnum<visa-resource-name>, error out=w1839:errorcluster)  [unwired: 1 out]
                }
                frame True {
                }
              }
            }
            n475 = Array Size(array=w1822) -> (size(s)=w1823:i32)
            n476 = case shown="2" w1823 {
              tunnel: ["PowerOnSensor >> Rack1" ("State(s) in Front (\"\")") "EnableSensor >> Rack2" ("State(s) in Front (\"\")")] -> w1821
              frame 1, Default {
              }
              frame 2 {
              }
            }
          }
          frame "Rack2" {
            n477 = Index Array(array=w1853, index=1) -> (element=w1851:T15)
            n478 = Unbundle By Name(w1851) -> ("EnableSensor"=w1846:string[])
            n479 = for {
              tunnel: w1846 -> [w1857] mode=indexing
              tunnel: w1850 -> [w1858]
              tunnel: [w1854] -> w1847
              shift-right: [w1855] -> w1848
              shift-left: w1849 -> [w1856]
              n480 = VISA Write(VISA resource name=w1858, write buffer=w1857, error in (no error)=w1856) -> (VISA resource name out=w1854:refnum<visa-resource-name>, error out=w1855:errorcluster)  [unwired: 1 out]
            }
          }
        }
        n481 = Bundle By Name(cluster=w1807, "State"="Run") -> (w1806:T3)
        n482 = call <vilib>:"Add State(s) to Queue__JKI_lib_State_Machine.vi"("State(s) in Front (\"\")"=w1810, "State(s) in (\"\")"=w1818) -> ("States Out"=w1817:string)  [unwired: 13 in]
      }
      frame "PowerOnSensor" {
        n483 = Unbundle By Name(w1861) -> ("Part details.RackDependentOpcodes"=w1867:T14, "MI Offline?"=w1859:bool)
        n484 = case shown="\"Rack1\", Default" w1868 {
          tunnel: w1867 -> [w1874 w1905]
          tunnel: w1864 -> [w1880 w1902]
          tunnel: w1866 -> [w1879 w1901]
          tunnel: [w1872 w1900] -> w1865
          tunnel: [w1878 w1899] -> w1863
          tunnel: [w1873 "StartReelerMotor >> Rack 1" ("State(s) in Front (\"\")")] -> w1862
          tunnel: w1859 -> [w1871 _]
          frame "Rack1", Default {
            n485 = Index Array(array=w1874, index=0) -> (element=w1877:T15)
            n486 = Unbundle By Name(w1877) -> ("PowerOnSensor"=w1876:string[])
            n487 = for {
              tunnel: w1876 -> [w1888] mode=indexing
              tunnel: w1880 -> [w1889]
              tunnel: [w1885] -> w1878
              shift-right: [w1886] -> w1872
              shift-left: w1879 -> [w1887]
              tunnel: w1871 -> [w1884]
              n488 = case shown="True" w1884 {
                tunnel: w1889 -> [w1894 w1896]
                tunnel: w1888 -> [w1893 _]
                tunnel: w1887 -> [w1892 w1895]
                tunnel: [w1891 w1895] -> w1886
                tunnel: [w1890 w1896] -> w1885
                frame False {
                  n489 = VISA Write(VISA resource name=w1894, write buffer=w1893, error in (no error)=w1892) -> (VISA resource name out=w1890:refnum<visa-resource-name>, error out=w1891:errorcluster)  [unwired: 1 out]
                }
                frame True {
                }
              }
            }
            n490 = Array Size(array=w1874) -> (size(s)=w1875:i32)
            n491 = case shown="1, Default" w1875 {
              tunnel: ["StartReelerMotor >> Rack1" ("State(s) in Front (\"\")") "PowerOnSensor >> Rack2" ("State(s) in Front (\"\")")] -> w1873
              frame 1, Default {
              }
              frame 2 {
              }
            }
          }
          frame "Rack2" {
            n492 = Index Array(array=w1905, index=1) -> (element=w1903:T15)
            n493 = Unbundle By Name(w1903) -> ("PowerOnSensor"=w1898:string[])
            n494 = for {
              tunnel: w1898 -> [w1909] mode=indexing
              tunnel: w1902 -> [w1910]
              tunnel: [w1906] -> w1899
              shift-right: [w1907] -> w1900
              shift-left: w1901 -> [w1908]
              n495 = VISA Write(VISA resource name=w1910, write buffer=w1909, error in (no error)=w1908) -> (VISA resource name out=w1906:refnum<visa-resource-name>, error out=w1907:errorcluster)  [unwired: 1 out]
            }
          }
        }
        n496 = call <vilib>:"Add State(s) to Queue__JKI_lib_State_Machine.vi"("State(s) in Front (\"\")"=w1862, "State(s) in (\"\")"=w1870) -> ("States Out"=w1869:string)  [unwired: 13 in]
      }
      frame "StartReelerMotor" {
        n497 = Unbundle By Name(w1913) -> ("Part details.RackDependentOpcodes"=w1919:T14, "MI Offline?"=w1911:bool)
        n498 = case shown="\"Rack2\"" w1920 {
          tunnel: w1919 -> [w1926 w1957]
          tunnel: w1916 -> [w1932 w1954]
          tunnel: w1918 -> [w1931 w1953]
          tunnel: [w1924 w1952] -> w1917
          tunnel: [w1930 w1951] -> w1915
          tunnel: [w1925 "ReadyToRun" ("State(s) in Front (\"\")")] -> w1914
          tunnel: w1911 -> [w1923 _]
          frame "Rack1", Default {
            n499 = Index Array(array=w1926, index=0) -> (element=w1929:T15)
            n500 = Unbundle By Name(w1929) -> ("StartReelerMotor"=w1928:string[])
            n501 = for {
              tunnel: w1928 -> [w1940] mode=indexing
              tunnel: w1932 -> [w1941]
              tunnel: [w1937] -> w1930
              shift-right: [w1938] -> w1924
              shift-left: w1931 -> [w1939]
              tunnel: w1923 -> [w1936]
              n502 = case shown="True" w1936 {
                tunnel: w1941 -> [w1946 w1948]
                tunnel: w1940 -> [w1945 _]
                tunnel: w1939 -> [w1944 w1947]
                tunnel: [w1943 w1947] -> w1938
                tunnel: [w1942 w1948] -> w1937
                frame False {
                  n503 = VISA Write(VISA resource name=w1946, write buffer=w1945, error in (no error)=w1944) -> (VISA resource name out=w1942:refnum<visa-resource-name>, error out=w1943:errorcluster)  [unwired: 1 out]
                }
                frame True {
                }
              }
            }
            n504 = Array Size(array=w1926) -> (size(s)=w1927:i32)
            n505 = case shown="2" w1927 {
              tunnel: ["ReadyToRun" ("State(s) in Front (\"\")") "StartReelerMotor >> Rack2" ("State(s) in Front (\"\")")] -> w1925
              frame 1, Default {
              }
              frame 2 {
              }
            }
          }
          frame "Rack2" {
            n506 = Index Array(array=w1957, index=1) -> (element=w1955:T15)
            n507 = Unbundle By Name(w1955) -> ("StartReelerMotor"=w1950:string[])
            n508 = for {
              tunnel: w1950 -> [w1961] mode=indexing
              tunnel: w1954 -> [w1962]
              tunnel: [w1958] -> w1951
              shift-right: [w1959] -> w1952
              shift-left: w1953 -> [w1960]
              n509 = VISA Write(VISA resource name=w1962, write buffer=w1961, error in (no error)=w1960) -> (VISA resource name out=w1958:refnum<visa-resource-name>, error out=w1959:errorcluster)  [unwired: 1 out]
            }
          }
        }
        n510 = call <vilib>:"Add State(s) to Queue__JKI_lib_State_Machine.vi"("State(s) in Front (\"\")"=w1914, "State(s) in (\"\")"=w1922) -> ("States Out"=w1921:string)  [unwired: 13 in]
      }
      frame "ReadyToRun" {
        # "Ready To Run Message to SM"
        n511 = Unbundle By Name(w1963) -> ("Output Cluster_MI"=w1974:T5, "MIParameters"=w1971:T4)
        n512 = call "State wise behavior_MI.vi"("error in (no error)"=w1970, "State"="ReadyToRun", "MIRecipeOpcodes"=w1971, "VISA Refnum in"=w1967) -> ("error out"=w1969:errorcluster, "VISA Refnum out"=w1966:refnum<visa-resource-name>)  [unwired: 6 in]
        n513 = call "Output_MI.vi"("Machine Interface Actor in"=w1965, "Output Cluster_MI"=w1974, "State"="MessageToSM", "Sub State"="ReadyToRun", "error in (no error)"=w1969) -> ("Machine Interface Actor out"=w1964:refnum<class "Machine Interface.lvclass">, "error out"=w1975:errorcluster)  [unwired: 9 in]
        n514 = call <vilib>:"Add State(s) to Queue__JKI_lib_State_Machine.vi"("State(s) in (\"\")"=w1977) -> ("States Out"=w1976:string)  [unwired: 14 in]
      }
      frame "Pass" {
        n515 = Unbundle By Name(w1985) -> ("MIParameters"=w1983:T4)
        n516 = call "State wise behavior_MI.vi"("error in (no error)"=w1981, "State"="Pass", "MIRecipeOpcodes"=w1983, "VISA Refnum in"=w1979) -> ("error out"=w1980:errorcluster, "VISA Refnum out"=w1978:refnum<visa-resource-name>)  [unwired: 6 in]
        n517 = call <vilib>:"Add State(s) to Queue__JKI_lib_State_Machine.vi"("State(s) in (\"\")"=w1987) -> ("States Out"=w1986:string)  [unwired: 14 in]
      }
      frame "---------- Pause State ----------" {
        # "Do not put any code in this frame.\n(It is a separator )"
        n518 = call <vilib>:"Add State(s) to Queue__JKI_lib_State_Machine.vi"("State(s) in (\"\")"=w1993) -> ("States Out"=w1992:string)  [unwired: 14 in]
      }
      frame "HWPauseButtonPress" {
        n519 = Unbundle By Name(w2003) -> ("State"=w2002:string, "MIParameters.MIRecipeOpcodes.HardwareButtonDiagnostics.Pause"=w2001:string[], "Output Cluster_MI"=w1996:T5)
        n520 = Index Array(array=w2001, index=1) -> (element=w1999:string)
        n521 = case shown="\"HardwareButtonDiagnostics\"" w2002 {
          tunnel: w2005 -> [w2013 w2022]
          tunnel: [w2012 w2024] -> w2004
          tunnel: w1999 -> [_ w2025]
          tunnel: w1998 -> [w2016 w2027]
          tunnel: [w2016 w2026] -> w1997
          tunnel: w1996 -> [w2011 w2019]
          tunnel: w1995 -> [w2010 w2018]
          tunnel: [w2009 w2017] -> w1994
          frame Default {
            n522 = call "Output_MI.vi"("Machine Interface Actor in"=w2010, "Output Cluster_MI"=w2011, "State"="ButtonPress", "Sub State"="Pause" ("Button Press"), "error in (no error)"=w2013) -> ("Machine Interface Actor out"=w2009:refnum<class "Machine Interface.lvclass">, "error out"=w2012:errorcluster)  [unwired: 9 in]
          }
          frame "HardwareButtonDiagnostics" {
            n523 = call "Output_MI.vi"("Machine Interface Actor in"=w2018, "Output Cluster_MI"=w2019, "State"="ButtonPress", "Sub State"="Pause" ("Button Press"), "error in (no error)"=w2022) -> ("Machine Interface Actor out"=w2017:refnum<class "Machine Interface.lvclass">, "error out"=w2021:errorcluster)  [unwired: 9 in]
            n524 = VISA Write(VISA resource name=w2027, write buffer=w2025, error in (no error)=w2021) -> (VISA resource name out=w2026:refnum<visa-resource-name>, error out=w2024:errorcluster)  [unwired: 1 out]
          }
        }
        n525 = call <vilib>:"Add State(s) to Queue__JKI_lib_State_Machine.vi"("State(s) in Front (\"\")"="Wait" ("State(s) in Front (\"\")"), "State(s) in (\"\")"=w2008) -> ("States Out"=w2007:string)  [unwired: 13 in]
      }
      frame "Pause" {
        n526 = Unbundle By Name(w2052) -> ("MIParameters.DelayValuesInms.DisableSensors"=w2035:i32, "MIParameters"=w2054:T4, "Part details.RackDependentOpcodes"=w2034:T14, "MI Offline?"=w2028:bool)
        n527 = Array Size(array=w2034) -> (size(s)=w2033:i32)
        n528 = flat-sequence {
          tunnel: w2049 -> [w2066]
          tunnel: w2054 -> [w2067]
          tunnel: w2056 -> [w2064]
          tunnel: [w2063] -> w2043
          tunnel: [w2067] -> w2042
          tunnel: [w2065] -> w2041
          tunnel: [w2061] -> w2038
          tunnel: [w2062] -> w2036
          tunnel: w2035 -> [w2062]
          tunnel: w2034 -> [w2061]
          tunnel: w2033 -> [w2060]
          tunnel: [w2060] -> w2030
          tunnel: w2028 -> [w2059]
          tunnel: [w2096] -> w2047
          tunnel: [w2090] -> w2046
          tunnel: w2043 -> [w2097]
          tunnel: w2042 -> [w2095]
          tunnel: w2041 -> [w2091]
          tunnel: [w2098] -> w2039
          tunnel: w2038 -> [w2098]
          tunnel: [w2093] -> w2037
          tunnel: w2036 -> [w2093]
          tunnel: [w2092] -> w2031
          tunnel: w2030 -> [w2092]
          tunnel: w2047 -> [w2104]
          tunnel: w2046 -> [w2103]
          tunnel: [w2104] -> w2045
          tunnel: [w2103] -> w2044
          tunnel: [w2102] -> w2040
          tunnel: w2039 -> [w2102]
          tunnel: w2037 -> [w2101]
          tunnel: [w2100] -> w2032
          tunnel: w2031 -> [w2100]
          tunnel: [w2099] -> w2029
          tunnel: w2028 -> [w2099]
          tunnel: [w2108] -> w2048
          tunnel: [w2110] -> w2055
          tunnel: w2045 -> [w2111]
          tunnel: w2044 -> [w2109]
          tunnel: w2040 -> [w2107]
          tunnel: w2032 -> [w2106]
          tunnel: w2029 -> [w2105]
          frame #0 {
            n529 = for {
              N: w2060 -> [_]
              tunnel: w2066 -> [w2076]
              tunnel: [w2075] -> w2065
              tunnel: w2061 -> [w2070]
              shift-right: [w2073] -> w2063
              shift-left: w2064 -> [w2074]
              tunnel: w2059 -> [w2068]
              i -> [w2069]
              # "Stop Reeler motor"
              n530 = Index Array(array=w2070, index=w2069) -> (element=w2071:T15)
              n531 = Unbundle By Name(w2071) -> ("StopReelerMotor"=w2072:string[])
              n532 = for {
                tunnel: w2076 -> [w2082]
                tunnel: [w2081] -> w2075
                shift-right: [w2079] -> w2073
                shift-left: w2074 -> [w2080]
                tunnel: w2072 -> [w2078] mode=indexing
                tunnel: w2068 -> [w2077]
                n533 = case shown="False" w2077 {
                  tunnel: w2082 -> [w2087 w2089]
                  tunnel: [w2086 w2089] -> w2081
                  tunnel: w2080 -> [w2085 w2088]
                  tunnel: [w2084 w2088] -> w2079
                  tunnel: w2078 -> [w2083 _]
                  frame False {
                    n534 = VISA Write(VISA resource name=w2087, write buffer=w2083, error in (no error)=w2085) -> (VISA resource name out=w2086:refnum<visa-resource-name>, error out=w2084:errorcluster)  [unwired: 1 out]
                  }
                  frame True {
                  }
                }
              }
            }
          }
          frame #1 {
            # "Pause\nhardware\nchanges"
            n535 = call "State wise behavior_MI.vi"("error in (no error)"=w2097, "State"="Pause", "MIRecipeOpcodes"=w2095, "VISA Refnum in"=w2091) -> ("error out"=w2096:errorcluster, "VISA Refnum out"=w2090:refnum<visa-resource-name>)  [unwired: 6 in]
          }
          frame #2 {
            n536 = Wait (ms)(milliseconds to wait=w2101) -> ()  [unwired: 1 out]
          }
          frame #3 {
            n537 = for {
              N: w2106 -> [_]
              tunnel: w2107 -> [w2115]
              shift-right: [w2119] -> w2110
              shift-left: w2111 -> [w2120]
              shift-right: [w2117] -> w2108
              shift-left: w2109 -> [w2118]
              tunnel: w2105 -> [w2112]
              i -> [w2113]
              n538 = Index Array(array=w2115, index=w2113) -> (element=w2114:T15)
              n539 = Unbundle By Name(w2114) -> ("DisableSensor"=w2116:string[])
              n540 = for {
                shift-right: [w2125] -> w2119
                shift-left: w2120 -> [w2126]
                tunnel: w2116 -> [w2122] mode=indexing
                tunnel: w2118 -> [w2124]
                tunnel: [w2123] -> w2117
                tunnel: w2112 -> [w2121]
                n541 = case shown="False" w2121 {
                  tunnel: w2126 -> [w2131 w2132]
                  tunnel: [w2130 w2132] -> w2125
                  tunnel: w2124 -> [w2129 w2133]
                  tunnel: [w2128 w2133] -> w2123
                  tunnel: w2122 -> [w2127 _]
                  frame False {
                    n542 = VISA Write(VISA resource name=w2129, write buffer=w2127, error in (no error)=w2131) -> (VISA resource name out=w2128:refnum<visa-resource-name>, error out=w2130:errorcluster)  [unwired: 1 out]
                  }
                  frame True {
                  }
                }
              }
            }
          }
        }
        n543 = Bundle By Name(cluster=w2052, "State"="Pause") -> (w2051:T3)
        n544 = call <vilib>:"Add State(s) to Queue__JKI_lib_State_Machine.vi"("State(s) in (\"\")"=w2058) -> ("States Out"=w2057:string)  [unwired: 14 in]
      }
      frame "Fail" {
        n545 = Unbundle By Name(w2157) -> ("MIParameters.DelayValuesInms.DisableSensors"=w2141:i32, "MIParameters"=w2158:T4, "Part details.RackDependentOpcodes"=w2140:T14, "MI Offline?"=w2134:bool)
        n546 = Array Size(array=w2140) -> (size(s)=w2139:i32)
        n547 = flat-sequence {
          tunnel: w2155 -> [w2170]
          tunnel: w2158 -> [w2171]
          tunnel: w2160 -> [w2168]
          tunnel: [w2167] -> w2149
          tunnel: [w2171] -> w2148
          tunnel: [w2169] -> w2147
          tunnel: [w2165] -> w2144
          tunnel: [w2166] -> w2142
          tunnel: w2141 -> [w2166]
          tunnel: w2140 -> [w2165]
          tunnel: w2139 -> [w2164]
          tunnel: [w2164] -> w2136
          tunnel: w2134 -> [w2163]
          tunnel: [w2199] -> w2153
          tunnel: [w2194] -> w2152
          tunnel: w2149 -> [w2200]
          tunnel: w2148 -> [w2198]
          tunnel: w2147 -> [w2201]
          tunnel: [w2202] -> w2145
          tunnel: w2144 -> [w2202]
          tunnel: [w2196] -> w2143
          tunnel: w2142 -> [w2196]
          tunnel: [w2195] -> w2137
          tunnel: w2136 -> [w2195]
          tunnel: w2153 -> [w2208]
          tunnel: w2152 -> [w2207]
          tunnel: [w2208] -> w2151
          tunnel: [w2207] -> w2150
          tunnel: [w2206] -> w2146
          tunnel: w2145 -> [w2206]
          tunnel: w2143 -> [w2205]
          tunnel: [w2204] -> w2138
          tunnel: w2137 -> [w2204]
          tunnel: [w2203] -> w2135
          tunnel: w2134 -> [w2203]
          tunnel: [w2212] -> w2154
          tunnel: [w2214] -> w2159
          tunnel: w2151 -> [w2215]
          tunnel: w2150 -> [w2213]
          tunnel: w2146 -> [w2211]
          tunnel: w2138 -> [w2210]
          tunnel: w2135 -> [w2209]
          frame #0 {
            n548 = for {
              N: w2164 -> [_]
              tunnel: w2170 -> [w2180]
              tunnel: [w2179] -> w2169
              tunnel: w2165 -> [w2174]
              shift-right: [w2177] -> w2167
              shift-left: w2168 -> [w2178]
              tunnel: w2163 -> [w2172]
              i -> [w2173]
              # "Stop Reeler motor"
              n549 = Index Array(array=w2174, index=w2173) -> (element=w2175:T15)
              n550 = Unbundle By Name(w2175) -> ("StopReelerMotor"=w2176:string[])
              n551 = for {
                tunnel: w2180 -> [w2186]
                tunnel: [w2185] -> w2179
                shift-right: [w2183] -> w2177
                shift-left: w2178 -> [w2184]
                tunnel: w2176 -> [w2182] mode=indexing
                tunnel: w2172 -> [w2181]
                n552 = case shown="True" w2181 {
                  tunnel: w2186 -> [w2191 w2193]
                  tunnel: [w2190 w2193] -> w2185
                  tunnel: w2184 -> [w2189 w2192]
                  tunnel: [w2188 w2192] -> w2183
                  tunnel: w2182 -> [w2187 _]
                  frame False {
                    n553 = VISA Write(VISA resource name=w2191, write buffer=w2187, error in (no error)=w2189) -> (VISA resource name out=w2190:refnum<visa-resource-name>, error out=w2188:errorcluster)  [unwired: 1 out]
                  }
                  frame True {
                  }
                }
              }
            }
          }
          frame #1 {
            # "Fail\nhardware\nchanges"
            n554 = call "State wise behavior_MI.vi"("error in (no error)"=w2200, "State"="Fail", "MIRecipeOpcodes"=w2198, "VISA Refnum in"=w2201) -> ("error out"=w2199:errorcluster, "VISA Refnum out"=w2194:refnum<visa-resource-name>)  [unwired: 6 in]
          }
          frame #2 {
            n555 = Wait (ms)(milliseconds to wait=w2205) -> ()  [unwired: 1 out]
          }
          frame #3 {
            n556 = for {
              N: w2210 -> [_]
              tunnel: w2211 -> [w2219]
              shift-right: [w2223] -> w2214
              shift-left: w2215 -> [w2224]
              shift-right: [w2221] -> w2212
              shift-left: w2213 -> [w2222]
              tunnel: w2209 -> [w2216]
              i -> [w2217]
              n557 = Index Array(array=w2219, index=w2217) -> (element=w2218:T15)
              n558 = Unbundle By Name(w2218) -> ("DisableSensor"=w2220:string[])
              n559 = for {
                shift-right: [w2229] -> w2223
                shift-left: w2224 -> [w2230]
                tunnel: w2220 -> [w2226] mode=indexing
                tunnel: w2222 -> [w2228]
                tunnel: [w2227] -> w2221
                tunnel: w2216 -> [w2225]
                n560 = case shown="False" w2225 {
                  tunnel: w2230 -> [w2235 w2236]
                  tunnel: [w2234 w2236] -> w2229
                  tunnel: w2228 -> [w2233 w2237]
                  tunnel: [w2232 w2237] -> w2227
                  tunnel: w2226 -> [w2231 _]
                  frame False {
                    n561 = VISA Write(VISA resource name=w2233, write buffer=w2231, error in (no error)=w2235) -> (VISA resource name out=w2232:refnum<visa-resource-name>, error out=w2234:errorcluster)  [unwired: 1 out]
                  }
                  frame True {
                  }
                }
              }
            }
          }
        }
        n562 = call <vilib>:"Add State(s) to Queue__JKI_lib_State_Machine.vi"("State(s) in (\"\")"=w2162) -> ("States Out"=w2161:string)  [unwired: 14 in]
      }
      frame "HWBuzzerOffButtonPress" {
        n563 = Unbundle By Name(w2251) -> ("State"=w2245:string, "MIParameters.MIRecipeOpcodes.Pause.BuzzerOffButtonPress"=w2250:string[], "MIParameters.MIRecipeOpcodes.HardwareButtonDiagnostics.BuzzerOff"=w2244:string[], "Output Cluster_MI"=w2241:T5, "DisableRun"=w2238:bool)
        n564 = Index Array(array=w2244, index=1) -> (element=w2242:string)
        n565 = case shown="Default" w2245 {
          tunnel: w2250 -> [w2256 _]
          tunnel: w2249 -> [w2262 w2279]
          tunnel: [w2261 w2278] -> w2248
          tunnel: w2247 -> [w2260 w2277]
          tunnel: [w2259 w2273] -> w2246
          tunnel: w2242 -> [_ w2276]
          tunnel: w2240 -> [w2258 w2275]
          tunnel: w2241 -> [_ w2270]
          tunnel: [w2258 w2269] -> w2239
          tunnel: w2238 -> [w2255 _]
          frame Default {
            n566 = case shown="False" w2255 {
              tunnel: w2256 -> [w2264 w2268]
              tunnel: [w2263 w2266] -> w2254
              frame False {
                # "Opcode to Disable run after Buzzer off button is pressed, is sent to Timing unit"
                n567 = Index Array(array=w2264, index=0) -> (element=w2263:string)
              }
              frame True {
                # "Opcode to Enable run after Buzzer off button is pressed, is sent to Timing unit"
                n568 = Index Array(array=w2268, index=1) -> (element=w2266:string)
              }
            }
            n569 = VISA Write(VISA resource name=w2262, write buffer=w2254, error in (no error)=w2260) -> (VISA resource name out=w2261:refnum<visa-resource-name>, error out=w2259:errorcluster)  [unwired: 1 out]
            n570 = Wait (ms)(milliseconds to wait=u32 1) -> ()  [unwired: 1 out]
          }
          frame "HardwareButtonDiagnostics" {
            n571 = VISA Write(VISA resource name=w2279, write buffer=w2276, error in (no error)=w2277) -> (VISA resource name out=w2278:refnum<visa-resource-name>, error out=w2274:errorcluster)  [unwired: 1 out]
            n572 = call "Output_MI.vi"("Machine Interface Actor in"=w2275, "Output Cluster_MI"=w2270, "State"="ButtonPress", "Sub State"="BuzzerOff" ("Button Press"), "error in (no error)"=w2274) -> ("Machine Interface Actor out"=w2269:refnum<class "Machine Interface.lvclass">, "error out"=w2273:errorcluster)  [unwired: 9 in]
          }
        }
        n573 = call <vilib>:"Add State(s) to Queue__JKI_lib_State_Machine.vi"("State(s) in (\"\")"=w2253) -> ("States Out"=w2252:string)  [unwired: 14 in]
      }
      frame "---------- Stop State ----------" {
        # "Do not put any code in this frame.\n(It is a separator )"
        n574 = call <vilib>:"Add State(s) to Queue__JKI_lib_State_Machine.vi"("State(s) in (\"\")"=w2285) -> ("States Out"=w2284:string)  [unwired: 14 in]
      }
      frame "HWStopButtonPress" {
        n575 = Unbundle By Name(w2295) -> ("State"=w2294:string, "MIParameters.MIRecipeOpcodes.HardwareButtonDiagnostics.Stop"=w2293:string[], "Output Cluster_MI"=w2288:T5)
        n576 = Index Array(array=w2293, index=1) -> (element=w2291:string)
        n577 = case shown="\"HardwareButtonDiagnostics\"" w2294 {
          tunnel: w2297 -> [w2303 w2314]
          tunnel: [w2302 w2316] -> w2296
          tunnel: w2291 -> [_ w2317]
          tunnel: w2290 -> [w2308 w2319]
          tunnel: [w2308 w2318] -> w2289
          tunnel: w2287 -> [w2305 w2310]
          tunnel: w2288 -> [w2304 w2311]
          tunnel: [w2301 w2309] -> w2286
          frame Default {
            n578 = call "Output_MI.vi"("Machine Interface Actor in"=w2305, "Output Cluster_MI"=w2304, "State"="ButtonPress", "Sub State"="Stop" ("Button Press"), "error in (no error)"=w2303) -> ("Machine Interface Actor out"=w2301:refnum<class "Machine Interface.lvclass">, "error out"=w2302:errorcluster)  [unwired: 9 in]
          }
          frame "HardwareButtonDiagnostics" {
            n579 = call "Output_MI.vi"("Machine Interface Actor in"=w2310, "Output Cluster_MI"=w2311, "State"="ButtonPress", "Sub State"="Stop" ("Button Press"), "error in (no error)"=w2314) -> ("Machine Interface Actor out"=w2309:refnum<class "Machine Interface.lvclass">, "error out"=w2313:errorcluster)  [unwired: 9 in]
            n580 = VISA Write(VISA resource name=w2319, write buffer=w2317, error in (no error)=w2313) -> (VISA resource name out=w2318:refnum<visa-resource-name>, error out=w2316:errorcluster)  [unwired: 1 out]
          }
        }
        n581 = call <vilib>:"Add State(s) to Queue__JKI_lib_State_Machine.vi"("State(s) in Front (\"\")"="Wait" ("State(s) in Front (\"\")"), "State(s) in (\"\")"=w2300) -> ("States Out"=w2299:string)  [unwired: 13 in]
      }
      frame "Stop" {
        n582 = Unbundle By Name(w2329) -> ("MIParameters"=w2324:T4)
        n583 = call "State wise behavior_MI.vi"("error in (no error)"=w2323, "State"="DHBLS", "MIRecipeOpcodes"=w2324, "VISA Refnum in"=w2321) -> ("error out"=w2322:errorcluster, "VISA Refnum out"=w2320:refnum<visa-resource-name>)  [unwired: 6 in]
        n584 = Bundle By Name(cluster=w2329, "State"="Stop") -> (w2328:T3)
        n585 = call <vilib>:"Add State(s) to Queue__JKI_lib_State_Machine.vi"("State(s) in (\"\")"=w2331) -> ("States Out"=w2330:string)  [unwired: 14 in]
      }
      frame "HardwareReset" {
        n586 = Unbundle By Name(w2332) -> ("MIParameters"=w2337:T4)
        n587 = call "State wise behavior_MI.vi"("error in (no error)"=w2336, "State"="DHBLS", "MIRecipeOpcodes"=w2337, "VISA Refnum in"=w2334) -> ("error out"=w2335:errorcluster, "VISA Refnum out"=w2333:refnum<visa-resource-name>)  [unwired: 6 in]
        n588 = call <vilib>:"Add State(s) to Queue__JKI_lib_State_Machine.vi"("State(s) in (\"\")"=w2341) -> ("States Out"=w2340:string)  [unwired: 14 in]
      }
      frame "EnableDoorLimitSwitch" {
        n589 = Unbundle By Name(w2342) -> ("MIParameters"=w2347:T4)
        n590 = call "State wise behavior_MI.vi"("error in (no error)"=w2346, "State"="EnableDoorLimitSwitch", "MIRecipeOpcodes"=w2347, "VISA Refnum in"=w2344) -> ("error out"=w2345:errorcluster, "VISA Refnum out"=w2343:refnum<visa-resource-name>)  [unwired: 6 in]
        n591 = call <vilib>:"Add State(s) to Queue__JKI_lib_State_Machine.vi"("State(s) in (\"\")"=w2351) -> ("States Out"=w2350:string)  [unwired: 14 in]
      }
      frame "DisableDoorLimitSwitch" {
        n592 = Unbundle By Name(w2352) -> ("MIParameters"=w2357:T4)
        n593 = call "State wise behavior_MI.vi"("error in (no error)"=w2356, "State"="DisableDoorLimitSwitch", "MIRecipeOpcodes"=w2357, "VISA Refnum in"=w2354) -> ("error out"=w2355:errorcluster, "VISA Refnum out"=w2353:refnum<visa-resource-name>)  [unwired: 6 in]
        n594 = call <vilib>:"Add State(s) to Queue__JKI_lib_State_Machine.vi"("State(s) in (\"\")"=w2361) -> ("States Out"=w2360:string)  [unwired: 14 in]
      }
      frame "MoveMotorToHomePosition" {
        n595 = call <vilib>:"Add State(s) to Queue__JKI_lib_State_Machine.vi"("State(s) in Front (\"\")"="LimitSwitchStatusCheck >> Rack1" ("State(s) in Front (\"\")"), "State(s) in (\"\")"=w2368) -> ("States Out"=w2367:string)  [unwired: 13 in]
      }
      frame "---------- SoftwareExit State ----------" {
        # "Do not put any code in this frame.\n(It is a separator )"
        n596 = call <vilib>:"Add State(s) to Queue__JKI_lib_State_Machine.vi"("State(s) in (\"\")"=w2374) -> ("States Out"=w2373:string)  [unwired: 14 in]
      }
      frame "SoftwareExit" {
        n597 = Unbundle By Name(w2379) -> ("MIParameters"=w2380:T4)
        n598 = call "State wise behavior_MI.vi"("error in (no error)"=w2378, "State"="DHBLS", "MIRecipeOpcodes"=w2380, "VISA Refnum in"=w2376) -> ("error out"=w2377:errorcluster, "VISA Refnum out"=w2375:refnum<visa-resource-name>)  [unwired: 6 in]
        n599 = Bundle By Name(cluster=w2379, "State"="SoftwareExit") -> (w2384:T3)
        n600 = call <vilib>:"Add State(s) to Queue__JKI_lib_State_Machine.vi"("State(s) in Front (\"\")"="Wait" ("State(s) in Front (\"\")"), "State(s) in (\"\")"=w2387) -> ("States Out"=w2386:string)  [unwired: 13 in]
      }
      frame "Shutdown" {
        n601 = Unbundle By Name(w2400) -> ("Output Cluster_MI"=w2396:T5, "MIParameters"=w2395:T4)
        n602 = call "State wise behavior_MI.vi"("error in (no error)"=w2393, "State"="Shutdown", "MIRecipeOpcodes"=w2395, "VISA Refnum in"=w2391) -> ("error out"=w2392:errorcluster, "VISA Refnum out"=w2390:refnum<visa-resource-name>)  [unwired: 6 in]
        n603 = call "Output_MI.vi"("Machine Interface Actor in"=w2389, "Output Cluster_MI"=w2396, "State"="ButtonPress", "Sub State"="ExitApplication" ("Button Press"), "error in (no error)"=w2392) -> ("Machine Interface Actor out"=w2388:refnum<class "Machine Interface.lvclass">, "error out"=w2397:errorcluster)  [unwired: 9 in]
        n604 = call <vilib>:"Add State(s) to Queue__JKI_lib_State_Machine.vi"("State(s) in (\"\")"=w2402) -> ("States Out"=w2401:string)  [unwired: 14 in]
      }
      frame "----------  ----------" {
        n605 = call <vilib>:"Add State(s) to Queue__JKI_lib_State_Machine.vi"("State(s) in Front (\"\")"="Wait" ("State(s) in Front (\"\")"), "State(s) in (\"\")"=w2409) -> ("States Out"=w2408:string)  [unwired: 13 in]
      }
      frame "ReadyPositionReached" {
        n606 = call <vilib>:"Add State(s) to Queue__JKI_lib_State_Machine.vi"("State(s) in (\"\")"=w2415) -> ("States Out"=w2414:string)  [unwired: 14 in]
      }
      frame "IncorrectOpcode" {
        n607 = Unbundle By Name(w2420) -> ("Output Cluster_MI"=w2419:T5)
        n608 = Bundle By Name(cluster=w2419, "Error Message"="TMConfigurationError_0x03000102") -> (w2418:T5)
        n609 = call "Output_MI.vi"("Machine Interface Actor in"=w2417, "Output Cluster_MI"=w2418, "State"="ErrorMessage", "error in (no error)"=w2422) -> ("Machine Interface Actor out"=w2416:refnum<class "Machine Interface.lvclass">, "error out"=w2421:errorcluster)  [unwired: 10 in]
        n610 = call <vilib>:"Add State(s) to Queue__JKI_lib_State_Machine.vi"("State(s) in Front (\"\")"="Wait" ("State(s) in Front (\"\")"), "State(s) in (\"\")"=w2428) -> ("States Out"=w2427:string)  [unwired: 13 in]
      }
      frame "DoorUnlock" {
        n611 = Unbundle By Name(w2430) -> ("State"=w2429:string)
        n612 = case shown="\"Run\"" w2429 {
          tunnel: w2434 -> [w2445 w2446]
          tunnel: [w2444 w2446] -> w2433
          tunnel: w2430 -> [w2443 _]
          tunnel: w2432 -> [w2442 w2447]
          tunnel: [w2441 w2447] -> w2431
          frame "Run" {
            n613 = Unbundle By Name(w2443) -> ("Output Cluster_MI"=w2439:T5)
            n614 = call "Output_MI.vi"("Machine Interface Actor in"=w2442, "Output Cluster_MI"=w2439, "State"="ButtonPress", "Sub State"="DoorUnlock", "error in (no error)"=w2445) -> ("Machine Interface Actor out"=w2441:refnum<class "Machine Interface.lvclass">, "error out"=w2444:errorcluster)  [unwired: 9 in]
          }
          frame "PreRun", Default {
            # "On DoorUnlock message \nfrom time machine,\nPause is not sent to SM if\ncurrent state is PreRun"
          }
        }
        n615 = call <vilib>:"Add State(s) to Queue__JKI_lib_State_Machine.vi"("State(s) in (\"\")"=w2437) -> ("States Out"=w2436:string)  [unwired: 14 in]
      }
      frame "PreRun" {
        n616 = Bundle By Name(cluster=w2450, "State"="PreRun") -> (w2449:T3)
        n617 = call <vilib>:"Add State(s) to Queue__JKI_lib_State_Machine.vi"("State(s) in (\"\")"=w2455) -> ("States Out"=w2454:string)  [unwired: 14 in]
      }
      frame "Unknown Response" {
        n618 = Unbundle By Name(w2465) -> ("Output Cluster_MI"=w2459:T5, "Message from Hardware"=w2464:string)
        n619 = Concatenate Strings("TMConfigurationError_0x03000103", w2464) -> (w2460:string)
        n620 = Bundle By Name(cluster=w2459, "Error Message"=w2460) -> (w2458:T5)
        n621 = call "Output_MI.vi"("Machine Interface Actor in"=w2457, "Output Cluster_MI"=w2458, "State"="ErrorMessage", "error in (no error)"=w2462) -> ("Machine Interface Actor out"=w2456:refnum<class "Machine Interface.lvclass">, "error out"=w2461:errorcluster)  [unwired: 10 in]
        n622 = call <vilib>:"Add State(s) to Queue__JKI_lib_State_Machine.vi"("State(s) in Front (\"\")"="Wait" ("State(s) in Front (\"\")"), "State(s) in (\"\")"=w2470) -> ("States Out"=w2469:string)  [unwired: 13 in]
      }
    }
  }
  n623 = while {
    shift-right: [w2479] -> _
    shift-left: -1 -> [w2480]
    tunnel: "Machine Interface Actor in" -> [w2477]
    shift-right: [w2476] -> _
    shift-left: "" ("Message from Arduino") -> [w2475]
    tunnel: w23 -> [w2474]
    shift-right: [w2473] -> w9
    shift-left: w22 -> [w2472]
    shift-right: [w2471] -> _
    shift-left: refnum<visa-resource-name> refnum ("VISA resource") -> [w2478]
    stop <- w2481 stop-if-true
    # "Receiver loop"
    n624 = event shown="[0] Timeout" {
      selector: w2474 -> [w2487 _ _ w2536]
      dyn-events: _ -> [_ _ _ _]
      timeout: w2480 -> [_ _ _ _]
      tunnel: [_ _ _ TRUE] -> w2481
      tunnel: [w2488 0 0 -1] -> w2479
      tunnel: w2478 -> [w2491 _ w2524 w2537]
      tunnel: w2477 -> [w2490 _ _ w2530]
      tunnel: [w2482 "" ("Message from Arduino") "Message from Arduino" w2535] -> w2476
      tunnel: w2475 -> [w2489 _ _ w2535]
      tunnel: [w2486 w2520 w2525 w2532] -> w2473
      tunnel: w2472 -> [w2485 w2520 w2525 w2531]
      tunnel: [w2483 w2523 w2524 w2537] -> w2471
      event Timeout {
        n625 = event-data() -> ()  [unwired: 1 in, 1 out]
        n626 = property class="Instr"(reference=w2491, error in=w2485) -> (error out=w2484:errorcluster, "Bytes at Port"=w2492:u32)  [unwired: 1 out]
        "Bytes at Port" <- w2492
        n627 = case shown="1.." w2492 {
          selector: w2492 -> [_ w2510]
          tunnel: w2491 -> [w2494 w2509]
          tunnel: w2490 -> [_ w2508]
          tunnel: w2489 -> [w2493 w2505]
          tunnel: [50 50] -> w2488
          tunnel: w2487 -> [_ w2502]
          tunnel: [w2495 w2501] -> w2486
          tunnel: w2484 -> [w2495 w2500]
          tunnel: [w2494 w2498] -> w2483
          tunnel: [w2493 w2497] -> w2482
          frame 0, Default {
          }
          frame 1.. {
            n628 = Unbundle By Name(w2508) -> ("Message from Arduino"=w2507:refnum<user-event>)
            n629 = disable-structure shown="Enabled" {
              disable-tunnel: w2510 -> [_ _]
              disable-tunnel: w2509 -> [w2515 w2517]
              disable-tunnel: [w2514 w2519] -> w2497
              disable-tunnel: w2505 -> [_ w2519]
              disable-tunnel: w2500 -> [w2513 w2518]
              disable-tunnel: [w2516 w2518] -> w2499
              disable-tunnel: [w2512 w2517] -> w2498
              frame Enabled {
                n630 = VISA Read(VISA resource name=w2515, byte count=u32 7, error in (no error)=w2513) -> (VISA resource name out=w2512:refnum<visa-resource-name>, read buffer=w2514:string, error out=w2516:errorcluster)  [unwired: 1 out]
              }
              frame Disabled {
              }
            }
            "Arduino Read buffer" <- w2497
            n631 = Generate User Event(priority (normal)=usereventprio."high priority", user event=w2507, event data cluster=w2497, error in=w2499) -> (error out=w2503:errorcluster)  [unwired: 1 out]
            n632 = Flush Event Queue(0:w2502, 3:w2503) -> (11:w2501:errorcluster)  [unwired: 4 in, 2 out]
          }
        }
      }
      event User Event {
        n633 = event-data() -> ("VISA resource"=w2523:refnum<visa-resource-name>)  [unwired: 1 in]
        "VISA resource" <- w2523
      }
      event "Message from Arduino": Value Change {
        n634 = event-data() -> ()  [unwired: 1 in, 3 out]
      }
      event User Event {
        n635 = event-data() -> ()  [unwired: 1 in, 3 out]
        n636 = Unbundle By Name(w2530) -> ("Stop Arduino Rx Loop"=w2534:refnum<user-event>)  [unwired: 1 out]
        n637 = Unregister For Events(event registration refnum=w2536, error in=w2531) -> (error out=w2533:errorcluster)
        n638 = Destroy User Event(user event=w2534, error in=w2531) -> (error out=w2528:errorcluster)
        n639 = case shown="No Error" w2528 {
          selector: w2528 -> [w2540 _]
          tunnel: [w2540 errorcluster {"status"=FALSE, "code"=0, "source"=""} ("error constant")] -> w2529
          frame No Error {
          }
          frame Error {
          }
        }
        n640 = Merge Errors(w2529, w2533) -> (w2532:errorcluster)
      }
    }
  }
  n641 = Merge Errors(w28, w10, w9) -> (→"error out":errorcluster)
